vi "Laser_MAIN.vi"() -> ()   [LabVIEW 2013]
doc: "Пограмма управления мишенью лазерного источника ионов."
uses:
  <vilib>/Utility/miscctls.llb/LVPositionTypeDef.ctl
  <vilib>/Utility/inputDevices.llb/closeMouse.vi
panel:
  out "Текущая мишень:":string
  out "Флаг резерв. сохр.":bool
  in  "Шаг \nручного \nсдвига":string(combo)="5" caption="Шаг"
  in  "RightButton":bool
  in  "LeftButton":bool
  in  "DownButton":bool
  in  "UpButton":bool
  in  "М3":T1
  out "Знак перех. dX М10":i8
  out "Выстрелов осталось M10":u16=3
  in  "М10":T1
  in  "выстрел X М10":u16 step=1
  in  "выстрел Y М10":u16 step=1
  out "Знак перех. dX М9":i8
  out "Выстрелов осталось M9":u16=3
  in  "М9":T1
  in  "выстрел X М9":u16 step=1
  in  "выстрел Y М9":u16 step=1
  out "Выстрелов осталось M8":u16=3
  out "Знак перех. dX М8":i8
  in  "М8":T1
  in  "выстрел X М8":u16 step=1
  in  "выстрел Y М8":u16 step=1
  out "Выстрелов осталось M7":u16=3
  out "Знак перех. dX М7":i8
  in  "М7":T1
  in  "выстрел X М7":u16 step=1
  in  "выстрел Y М7":u16 step=1
  out "Выстрелов осталось M6":u16=3
  out "Знак перех. dX М6":i8
  in  "М6":T1
  in  "выстрел X М6":u16 step=1
  in  "выстрел Y М6":u16 step=1
  out "Выстрелов осталось M5":u16=3
  in  "М2":T1
  in  "М5":T1
  out "Знак перех. dX М5":i8
  in  "выстрел Y М5":u16 step=1
  in  "выстрел X М5":u16 step=1
  in  "М4":T1
  out "Знак перех. dX М4":i8
  in  "выстрел Y М4":u16 step=1
  in  "выстрел X М4":u16 step=1
  out "Знак перех. dX М3":i8
  in  "выстрел Y М3":u16 step=1
  in  "выстрел X М3":u16 step=1
  out "Знак перех. dX М2":i8
  in  "выстрел Y М2":u16 step=1
  in  "выстрел X М2":u16 step=1
  in  "выстрел Y М1":u16 step=1
  in  "выстрел X М1":u16 step=1
  out "Знак перех. dX М1":i8
  in  "М1":T1
  out "Выстрелов осталось M4":u16=3
  out "Выстрелов осталось M3":u16=3
  out "Выстрелов осталось M2":u16=3
  out "Выстрелов осталось M1":u16=3
  out "Статус":bool=TRUE caption="Готов!"
  in  "Tab control":enum32{" Мишени", " Настройки TCP"}(tab)
  in  "Перемотка пленки":bool
  in  "Фокус --":bool
  in  "Фокус +":bool
  in  "Сбросить конфигурацию":bool
  in  "Шаг вперед":bool
  in  "XY лазера":bool caption="осталось: 1"
  in  "текущ. инфо":bool caption="4"
  out "флаг закрытия с сохр.":bool
  in  "Загрузить настройки":bool
  in  "Конфигурация сохранена":bool
  in  "Мишень 10":picture
  in  "Мишень 9":picture
  in  "Мишень 8":picture
  in  "Мишень 7":picture
  in  "Мишень 6":picture
  in  "Упр. звуком":bool
  in  "Мишень 5":picture
  in  "Мишень 4":picture
  in  "Мишень 3":picture
  in  "Добавить мишень":bool
  in  "Мишень 2":picture
  in  "Мишень 1":picture
  in  "Выстрелов до перемотки пленки":u16=100
  out "Осталось:":u16(slide)=3 scale=100.0..1.0
  out "id мишени":u16=1
  in  "Счетчик выстрелов:":u32
  in  "TCP read data":string
  out "Slide X axis":u8(slide) max=100 scale=0.0..100.0
  out "Slide Y axis":u8(slide) max=50 step=1
  in  "Снимок сохранен":bool
  out "con err":bool caption="Connect"
  in  "Выстрел по мишени!":u32
  out "Счетчик мишеней":u8=3
  out "Соединение с блоком":bool
  out "Флаг соединения с прибором":bool caption="Connect"
  in  "порт":u16=10001
  in  "IP-адрес":string="172.16.21.200"
  in  "Disconnect":bool caption="Disconn"
  out "Соединение":bool
  in  "Connect":bool
  out "TCP error source":string
  in  "stop":bool
  out "code out":i32 format="%0.0f"
  out "read_error_indicator":bool
  in  "Connect 2":bool caption="Connect"
  in  "flag1":bool caption="Disconn"
  out "x+1":dbl
  out "TCP con ID":refnum<k5>
  out "Текущая конфигурация:":path
  out "Con.err.text":bool caption="Ошибка соединения с блоком..."
  # "Ручное управление \nлазером в пределах \nвыбранной мишени"
  # "Шаг перехода по Y, мм"
  # "Доп. настройки"
  # "Файлы"
  # "Мишени"
  # "Задано:"
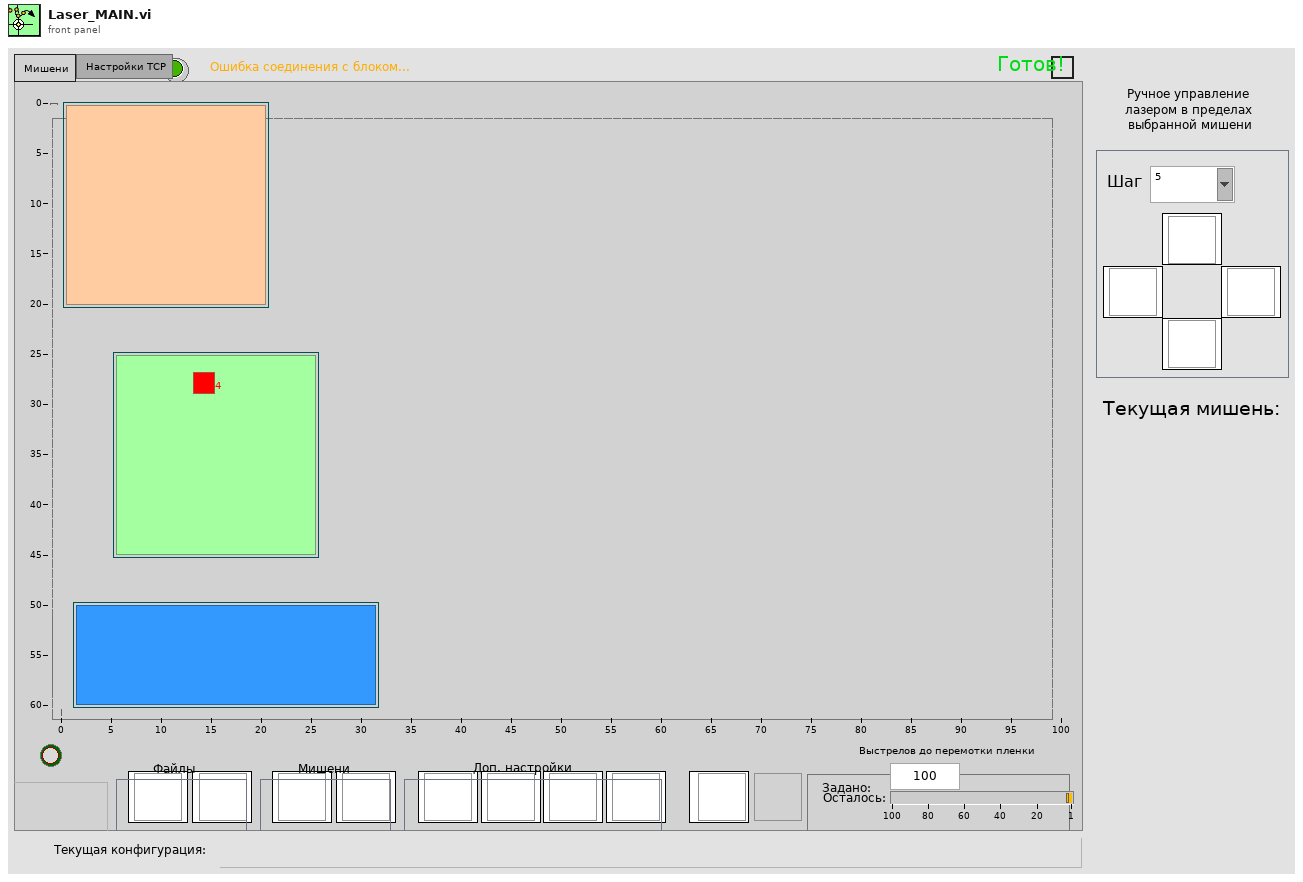
[diagram p1: front panel]
types:
  T1 = cluster{"Название мишени":string, "Х0_position":u16, "Y0_position":u16, "Длина, мм":u16, "Ширина, мм":u16, "Шаг перехода по горизонтали":dbl, "Шаг перехода по вертикали":dbl, "Выстрелов до перехода":u16, "Xo to send ":u16, "Yo to send":u16}
  T2 = enum8{"Enabled", "Disabled", "Disabled and Grayed Out"}
  T3 = typedef "LVPositionTypeDef.ctl" = cluster{"Left":i32, "Top":i32}
  T4 = typedef "imagedata.ctl" = cluster{"image type":i32, "image depth":i32, "image":u8[], "mask":u8[], "colors":u32[], "Rectangle":cluster{"left":i16, "top":i16, "right":i16, "bottom":i16}}
  T5 = cluster{"id команды":u8, "№ мишени":u8, "Коорд. выстрела X ст.байт":u8, "Коорд. выстрела X мл.байт":u8, "Коорд. выстрела Y cт.байт":u8, "Коорд. выстрела Y мл.байт":u8, "Знак dX":i8, "выст. до перех. cт. байт":u8, "выст. до перех. мл. байт":u8, "выст. до перем. пленки ст. байт":u8, "выст. до перем. пленки мл. байт":u8}
  T6 = cluster{"номер мишени (id)":u8, u8, u8, u8, u8, u8, u8, u8, u8, u8, u8, u8, u8, u8, u8, u8, u8, u8, u8, u8}
  T7 = cluster{"доп команда":u8, u8, u8, u8, u8, u8, u8, u8, u8, u8, u8, u8, u8, u8, u8, u8, u8, u8, u8, u8}
  T8 = cluster{"М1":cluster{"Название мишени":string, "Х0_position":u16, "Y0_position":u16, "Длина, мм":u16, "Ширина, мм":u16, "Шаг перехода по горизонтали":dbl, "Шаг перехода по вертикали":dbl, "Выстрелов до перехода":u16, "Xo to send ":u16, "Yo to send":u16}, "М2":cluster{"Название мишени":string, "Х0_position":u16, "Y0_position":u16, "Длина, мм":u16, "Ширина, мм":u16, "Шаг перехода по горизонтали":dbl, "Шаг перехода по вертикали":dbl, "Выстрелов до перехода":u16, "Xo to send ":u16, "Yo to send":u16}, "М3":cluster{"Название мишени":string, "Х0_position":u16, "Y0_position":u16, "Длина, мм":u16, "Ширина, мм":u16, "Шаг перехода по горизонтали":dbl, "Шаг перехода по вертикали":dbl, "Выстрелов до перехода":u16, "Xo to send ":u16, "Yo to send":u16}, "М4":cluster{"Название мишени":string, "Х0_position":u16, "Y0_position":u16, "Длина, мм":u16, "Ширина, мм":u16, "Шаг перехода по горизонтали":dbl, "Шаг перехода по вертикали":dbl, "Выстрелов до перехода":u16, "Xo to send ":u16, "Yo to send":u16}, "М5":cluster{"Название мишени":string, "Х0_position":u16, "Y0_position":u16, "Длина, мм":u16, "Ширина, мм":u16, "Шаг перехода по горизонтали":dbl, "Шаг перехода по вертикали":dbl, "Выстрелов до перехода":u16, "Xo to send ":u16, "Yo to send":u16}, "М6":cluster{"Название мишени":string, "Х0_position":u16, "Y0_position":u16, "Длина, мм":u16, "Ширина, мм":u16, "Шаг перехода по горизонтали":dbl, "Шаг перехода по вертикали":dbl, "Выстрелов до перехода":u16, "Xo to send ":u16, "Yo to send":u16}, "М7":cluster{"Название мишени":string, "Х0_position":u16, "Y0_position":u16, "Длина, мм":u16, "Ширина, мм":u16, "Шаг перехода по горизонтали":dbl, "Шаг перехода по вертикали":dbl, "Выстрелов до перехода":u16, "Xo to send ":u16, "Yo to send":u16}, "М8":cluster{"Название мишени":string, "Х0_position":u16, "Y0_position":u16, "Длина, мм":u16, "Ширина, мм":u16, "Шаг перехода по горизонтали":dbl, "Шаг перехода по вертикали":dbl, "Выстрелов до перехода":u16, "Xo to send ":u16, "Yo to send":u16}, "М9":cluster{"Название мишени":string, "Х0_position":u16, "Y0_position":u16, "Длина, мм":u16, "Ширина, мм":u16, "Шаг перехода по горизонтали":dbl, "Шаг перехода по вертикали":dbl, "Выстрелов до перехода":u16, "Xo to send ":u16, "Yo to send":u16}, "М10":cluster{"Название мишени":string, "Х0_position":u16, "Y0_position":u16, "Длина, мм":u16, "Ширина, мм":u16, "Шаг перехода по горизонтали":dbl, "Шаг перехода по вертикали":dbl, "Выстрелов до перехода":u16, "Xo to send ":u16, "Yo to send":u16}}
  T9 = cluster{"выстрел X М1":u16, "выстрел Y М1":u16, "выстрел X М2":u16, "выстрел Y М2":u16, "выстрел X М3":u16, "выстрел Y М3":u16, "выстрел X М4":u16, "выстрел Y М4":u16, "выстрел X М5":u16, "выстрел Y М5":u16}
  T10 = cluster{"выстрел X М6":u16, "выстрел Y М6":u16, "выстрел X М7":u16, "выстрел Y М7":u16, "выстрел X М8":u16, "выстрел Y М8":u16, "выстрел X М9":u16, "выстрел Y М9":u16, "выстрел X М10":u16, "выстрел Y М10":u16}
  T11 = cluster{"Знак перех. dX М1":i8, "Знак перех. dX М2":i8, "Знак перех. dX М3":i8, "Знак перех. dX М4":i8, "Знак перех. dX М5":i8, "Знак перех. dX М6":i8, "Знак перех. dX М7":i8, "Знак перех. dX М8":i8, "Знак перех. dX М9":i8, "Знак перех. dX М10":i8}
  T12 = cluster{"Мишень 1":picture, "Мишень 2":picture, "Мишень 3":picture, "Мишень 4":picture, "Мишень 5":picture, "Мишень 6":picture, "Мишень 7":picture, "Мишень 8":picture, "Мишень 9":picture, "Мишень 10":picture}
  T13 = cluster{"Visible":bool, "Visible":bool, "Visible":bool, "Visible":bool, "Visible":bool, "Visible":bool, "Visible":bool, "Visible":bool, "Visible":bool, "Visible":bool}
  T14 = cluster{"Выстрелов осталось M1 ":u16, "Выстрелов осталось M2":u16, "Выстрелов осталось M3":u16, "Выстрелов осталось M4":u16, "Выстрелов осталось M5":u16, "Выстрелов осталось M6":u16, "Выстрелов осталось M7":u16, "Выстрелов осталось M8":u16, "Выстрелов осталось M9":u16, "Выстрелов осталось M10":u16}
  T15 = cluster{"Счетчик мишеней":u32, "Счетчик мишеней":u32}
  T16 = cluster{"Счетчик мишеней":i32, "Счетчик мишеней":i32}
  T17 = cluster{"Мишень 1":refnum<vi>, "Мишень 2":refnum<vi>, "Мишень 3":refnum<vi>, "Мишень 4":refnum<vi>, "Мишень 5":refnum<vi>, "Мишень 6":refnum<vi>, "Мишень 7":refnum<vi>, "Мишень 8":refnum<vi>, "Мишень 9":refnum<vi>, "Мишень 10":refnum<vi>}
  T18 = cluster{"Pict Refnum":refnum<vi>, "Pict Refnum 2":refnum<vi>, "Pict Refnum 3":refnum<vi>, "Pict Refnum 4":refnum<vi>, "Pict Refnum 5":refnum<vi>, "Pict Refnum 6":refnum<vi>, "Pict Refnum 7":refnum<vi>, "Pict Refnum 8":refnum<vi>, "Picture in Refnum 9":refnum<vi>, "Pict Refnum 10":refnum<vi>}
  T19 = cluster{"1":u16, "2":u16, "3":u16, "4":u16, "5":u16, "6":u16, "7":u16, "8":u16, "9":u16, "10":u16}
  T20 = cluster{"default value 1":i8, "default value 1":i8, "default value 1":i8, "default value 1":i8, "default value 1":i8, "default value 1":i8, "default value 1":i8, "default value 1":i8, "default value 1":i8, "default value 1":i8}
  T21 = cluster{"Кластер параметров мишени":cluster{"Название мишени":string, "Х0_position":u16, "Y0_position":u16, "Длина, мм":u16, "Ширина, мм":u16, "Шаг перехода по горизонтали":dbl, "Шаг перехода по вертикали":dbl, "Выстрелов до перехода":u16, "Xo to send ":u16, "Yo to send":u16}, "Кластер параметров мишени":cluster{"Название мишени":string, "Х0_position":u16, "Y0_position":u16, "Длина, мм":u16, "Ширина, мм":u16, "Шаг перехода по горизонтали":dbl, "Шаг перехода по вертикали":dbl, "Выстрелов до перехода":u16, "Xo to send ":u16, "Yo to send":u16}, "Кластер параметров мишени":cluster{"Название мишени":string, "Х0_position":u16, "Y0_position":u16, "Длина, мм":u16, "Ширина, мм":u16, "Шаг перехода по горизонтали":dbl, "Шаг перехода по вертикали":dbl, "Выстрелов до перехода":u16, "Xo to send ":u16, "Yo to send":u16}, "Кластер параметров мишени":cluster{"Название мишени":string, "Х0_position":u16, "Y0_position":u16, "Длина, мм":u16, "Ширина, мм":u16, "Шаг перехода по горизонтали":dbl, "Шаг перехода по вертикали":dbl, "Выстрелов до перехода":u16, "Xo to send ":u16, "Yo to send":u16}, "Кластер параметров мишени":cluster{"Название мишени":string, "Х0_position":u16, "Y0_position":u16, "Длина, мм":u16, "Ширина, мм":u16, "Шаг перехода по горизонтали":dbl, "Шаг перехода по вертикали":dbl, "Выстрелов до перехода":u16, "Xo to send ":u16, "Yo to send":u16}, "Кластер параметров мишени":cluster{"Название мишени":string, "Х0_position":u16, "Y0_position":u16, "Длина, мм":u16, "Ширина, мм":u16, "Шаг перехода по горизонтали":dbl, "Шаг перехода по вертикали":dbl, "Выстрелов до перехода":u16, "Xo to send ":u16, "Yo to send":u16}, "Кластер параметров мишени":cluster{"Название мишени":string, "Х0_position":u16, "Y0_position":u16, "Длина, мм":u16, "Ширина, мм":u16, "Шаг перехода по горизонтали":dbl, "Шаг перехода по вертикали":dbl, "Выстрелов до перехода":u16, "Xo to send ":u16, "Yo to send":u16}, "Кластер параметров мишени":cluster{"Название мишени":string, "Х0_position":u16, "Y0_position":u16, "Длина, мм":u16, "Ширина, мм":u16, "Шаг перехода по горизонтали":dbl, "Шаг перехода по вертикали":dbl, "Выстрелов до перехода":u16, "Xo to send ":u16, "Yo to send":u16}, "Кластер параметров мишени":cluster{"Название мишени":string, "Х0_position":u16, "Y0_position":u16, "Длина, мм":u16, "Ширина, мм":u16, "Шаг перехода по горизонтали":dbl, "Шаг перехода по вертикали":dbl, "Выстрелов до перехода":u16, "Xo to send ":u16, "Yo to send":u16}, "Кластер параметров мишени":cluster{"Название мишени":string, "Х0_position":u16, "Y0_position":u16, "Длина, мм":u16, "Ширина, мм":u16, "Шаг перехода по горизонтали":dbl, "Шаг перехода по вертикали":dbl, "Выстрелов до перехода":u16, "Xo to send ":u16, "Yo to send":u16}}
  T22 = enum16{"Left Button", "Center Button", "Right Button", "Window Close"}
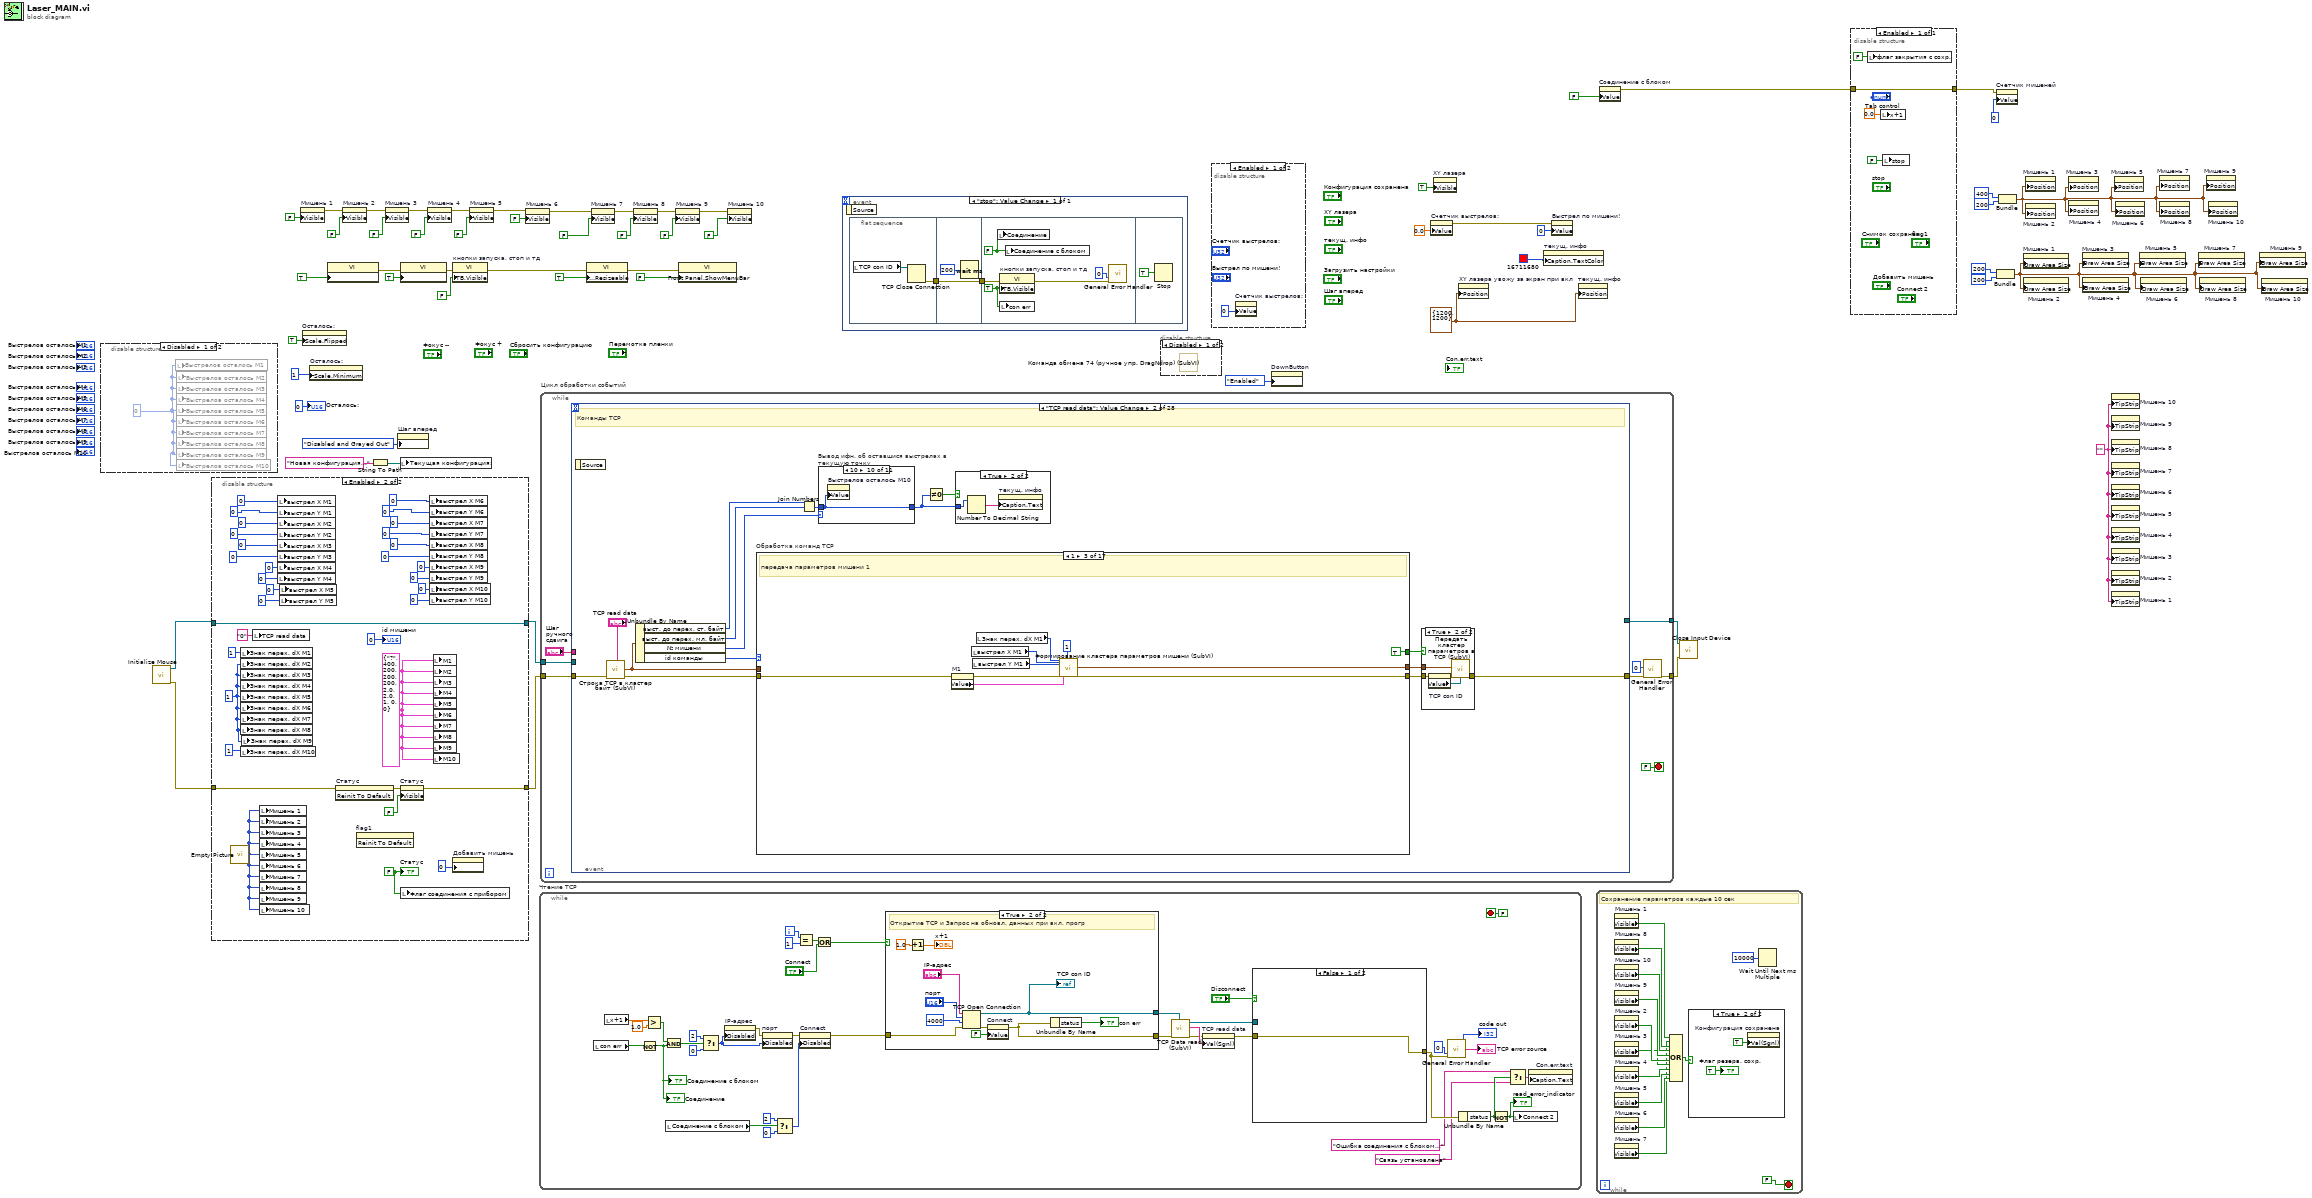
[diagram p0: block diagram]
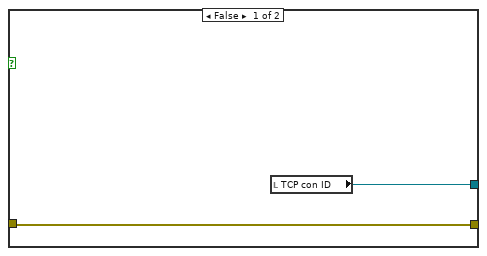
[diagram p5: hidden frame]
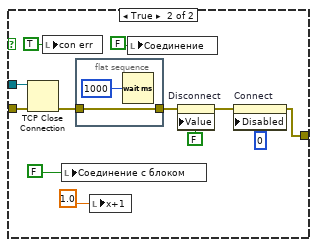
[diagram p6: hidden frame]
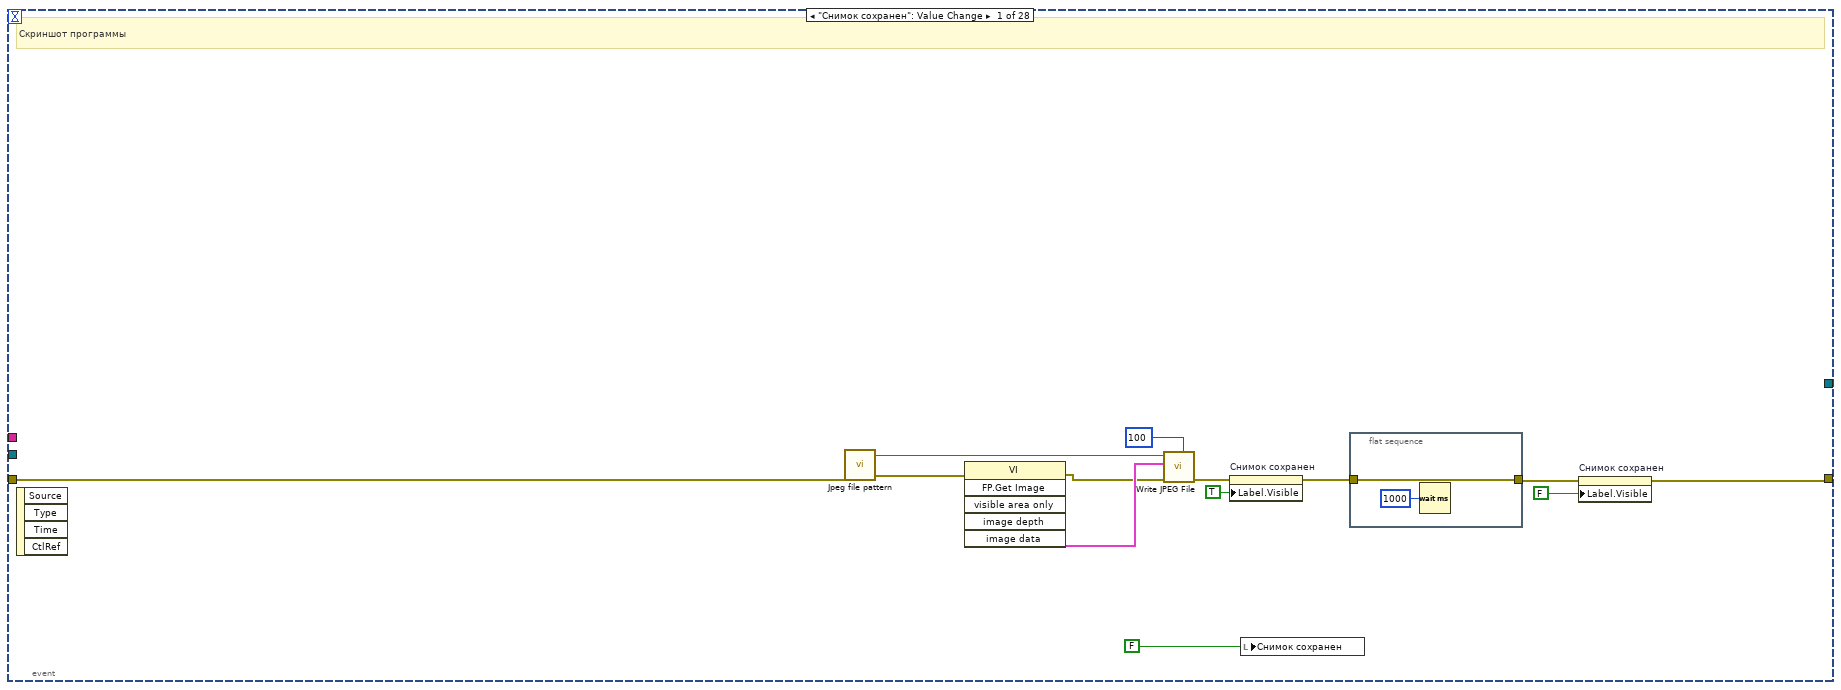
[diagram p9: hidden frame]
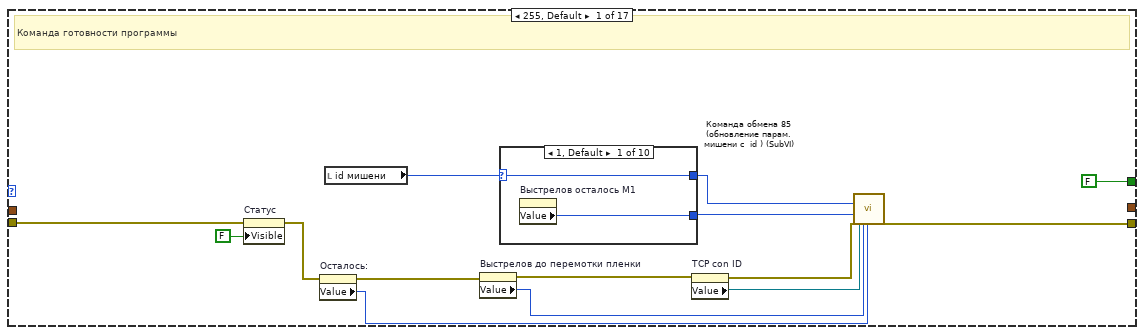
[diagram p12: hidden frame]
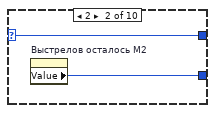
[diagram p13: hidden frame]
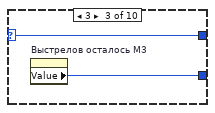
[diagram p14: hidden frame]
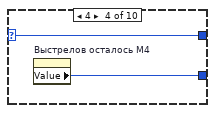
[diagram p15: hidden frame]
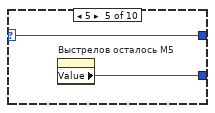
[diagram p16: hidden frame]
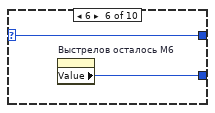
[diagram p17: hidden frame]
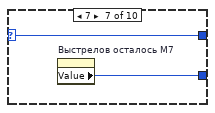
[diagram p18: hidden frame]
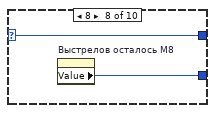
[diagram p19: hidden frame]
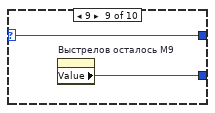
[diagram p20: hidden frame]
diagram:
  w8 = "" ("Tip Strip")
  w49 = T3 {"Left"=1200, "Top"=1200} ("Position")
  n1 = disable-structure shown="Disabled" {
    frame Disabled {
      w59 = u16 0
      n2 = local write "Выстрелов осталось M1"(w59) -> ()
      n3 = local write "Выстрелов осталось M2"(w59) -> ()
      n4 = local write "Выстрелов осталось M3"(w59) -> ()
      n5 = local write "Выстрелов осталось M4"(w59) -> ()
      n6 = local write "Выстрелов осталось M5"(w59) -> ()
      n7 = local write "Выстрелов осталось M6"(w59) -> ()
      n8 = local write "Выстрелов осталось M7"(w59) -> ()
      n9 = local write "Выстрелов осталось M8"(w59) -> ()
      n10 = local write "Выстрелов осталось M9"(w59) -> ()
      n11 = local write "Выстрелов осталось M10"(w59) -> ()
    }
    frame Enabled {
    }
  }
  n12 = call <vilib>:"Initialize Mouse.vi"() -> ("error out"=w51:errorcluster, "device ID"=w53:refnum<k1>)  [unwired: 1 in, 9 out]
  n13 = disable-structure shown="Enabled" {
    disable-tunnel: [_ w93] -> w54
    disable-tunnel: w53 -> [_ w93]
    disable-tunnel: [_ w64] -> w52
    disable-tunnel: w51 -> [_ w92]
    frame Disabled {
    }
    frame Enabled {
      w88 = i8 1 ("Выстрелов осталось M1")
      w89 = T1 {"Название мишени"="?", "Х0_position"=400, "Y0_position"=200, "Длина, мм"=200, "Ширина, мм"=200, "Шаг перехода по горизонтали"=2.0, "Шаг перехода по вертикали"=2.0, "Выстрелов до перехода"=1, "Xo to send "=0, "Yo to send"=0} ("Параметры М1")
      w61 = FALSE ("Готов")
      n14 = call "Empty Picture"() -> ("empty picture"=w65:picture)
      n15 = local write "Знак перех. dX М1"(i8 1 ("Знак перех. dX М1")) -> ()
      n16 = local write "Знак перех. dX М2"(w88) -> ()
      n17 = local write "Знак перех. dX М3"(w88) -> ()
      n18 = local write "Знак перех. dX М4"(w88) -> ()
      n19 = local write "Знак перех. dX М5"(w88) -> ()
      n20 = local write "Знак перех. dX М6"(w88) -> ()
      n21 = local write "Знак перех. dX М7"(w88) -> ()
      n22 = local write "Знак перех. dX М8"(w88) -> ()
      n23 = local write "Знак перех. dX М10"(i8 1 ("Выстрелов осталось M1")) -> ()
      n24 = local write "Знак перех. dX М9"(w88) -> ()
      n25 = local write "TCP read data"("0" ("TCP read data")) -> ()
      n26 = local write "Мишень 1"(w65) -> ()
      n27 = local write "Мишень 2"(w65) -> ()
      n28 = local write "Мишень 3"(w65) -> ()
      n29 = local write "Мишень 4"(w65) -> ()
      n30 = local write "Мишень 5"(w65) -> ()
      n31 = local write "Мишень 6"(w65) -> ()
      n32 = local write "Мишень 7"(w65) -> ()
      n33 = local write "Мишень 8"(w65) -> ()
      n34 = local write "Мишень 9"(w65) -> ()
      n35 = local write "Мишень 10"(w65) -> ()
      n36 = local write "выстрел X М1"(u16 0 ("Выстрелов осталось M1")) -> ()
      n37 = local write "выстрел Y М1"(u16 0 ("Выстрелов осталось M2")) -> ()
      n38 = local write "выстрел X М2"(u16 0 ("Выстрелов осталось M3")) -> ()
      n39 = local write "выстрел Y М2"(u16 0 ("Выстрелов осталось M4")) -> ()
      n40 = local write "выстрел X М3"(u16 0 ("Выстрелов осталось M5")) -> ()
      n41 = local write "выстрел Y М3"(u16 0 ("Выстрелов осталось M6")) -> ()
      n42 = local write "выстрел X М4"(u16 0 ("выстрел X М9")) -> ()
      n43 = local write "выстрел Y М4"(u16 0 ("выстрел Y М9")) -> ()
      n44 = local write "выстрел X М5"(u16 0 ("выстрел X М10")) -> ()
      n45 = local write "выстрел Y М5"(u16 0 ("выстрел Y М10")) -> ()
      n46 = invoke on="Статус" class="Bool (strict)" method="Reinit To Default"(error in=w92) -> (error out=w90:errorcluster)  [unwired: 2 in, 2 out]
      n47 = invoke on="flag1" class="Bool (strict)" method="Reinit To Default"() -> ()  [unwired: 3 in, 3 out]
      n48 = property on="Статус" class="Bool (strict)"(error in=w90, "Visible"=FALSE) -> (error out=w64:errorcluster)  [unwired: 1 in, 1 out]
      n49 = local write "Флаг соединения с прибором"(w61) -> ()
      n50 = local write "выстрел X М6"(u16 0 ("Выстрелов осталось M1")) -> ()
      n51 = local write "выстрел Y М6"(u16 0 ("Выстрелов осталось M2")) -> ()
      n52 = local write "выстрел X М7"(u16 0 ("Выстрелов осталось M3")) -> ()
      n53 = local write "выстрел Y М7"(u16 0 ("Выстрелов осталось M4")) -> ()
      n54 = local write "выстрел X М8"(u16 0 ("Выстрелов осталось M5")) -> ()
      n55 = local write "выстрел Y М8"(u16 0 ("Выстрелов осталось M6")) -> ()
      n56 = local write "выстрел X М9"(u16 0 ("выстрел X М9")) -> ()
      n57 = local write "выстрел Y М9"(u16 0 ("выстрел Y М9")) -> ()
      n58 = local write "выстрел X М10"(u16 0 ("выстрел X М10")) -> ()
      n59 = local write "выстрел Y М10"(u16 0 ("выстрел Y М10")) -> ()
      n60 = local write "М1"(w89) -> ()
      n61 = local write "М2"(w89) -> ()
      n62 = local write "М3"(w89) -> ()
      n63 = local write "М4"(w89) -> ()
      n64 = local write "М5"(w89) -> ()
      n65 = local write "М6"(w89) -> ()
      n66 = local write "М7"(w89) -> ()
      n67 = local write "М8"(w89) -> ()
      n68 = local write "М9"(w89) -> ()
      n69 = local write "М10"(w89) -> ()
      n70 = property on="Добавить мишень" class="Bool (strict)"("DisabledEnum"=i8 0 ("Выстрелов осталось M1")) -> ()  [unwired: 2 in, 2 out]
      "Статус" <- w61
      "id мишени" <- u16 0 ("id мишени")
    }
  }
  n71 = property on="Мишень 1" class="Pict"("Visible"=FALSE) -> (error out=w35:errorcluster)  [unwired: 2 in, 1 out]
  n72 = property on="Осталось:" class="Slide (strict)"("Scale.Flipped"=TRUE) -> ()  [unwired: 2 in, 2 out]
  n73 = property on="Осталось:" class="Slide (strict)"("Scale.Minimum"=u16 1 ("До перемотки осталось")) -> ()  [unwired: 2 in, 2 out]
  n74 = property class="VI"("Front Panel.Minimizeable"=TRUE ("Front Panel Window:Minimizable")) -> (error out=w41:errorcluster)  [unwired: 2 in, 1 out]
  n75 = property on="Мишень 2" class="Pict"(error in=w35, "Visible"=FALSE) -> (error out=w32:errorcluster)  [unwired: 1 in, 1 out]
  n76 = String To Path(string="Новая конфигурация...") -> (path=w7:path)
  n77 = property on="Мишень 3" class="Pict"(error in=w32, "Visible"=FALSE) -> (error out=w30:errorcluster)  [unwired: 1 in, 1 out]
  n78 = property on="Шаг вперед" class="Bool (strict)"("DisabledEnum"=T2."Disabled and Grayed Out" ("Disabled")) -> ()  [unwired: 2 in, 2 out]
  n79 = property class="VI"(error in=w41, "Front Panel.TitleBarVis"=TRUE ("Front Panel Window:Title Bar Visible")) -> (error out=w40:errorcluster)  [unwired: 1 in, 1 out]
  n80 = local write "Текущая конфигурация:"(w7) -> ()
  n81 = property on="Мишень 4" class="Pict"(error in=w30, "Visible"=FALSE) -> (error out=w28:errorcluster)  [unwired: 1 in, 1 out]
  n82 = property on="кнопки запуска, стоп и тд" class="VI"(error in=w40, "TB.Visible"=FALSE ("Tool Bar:Visible")) -> (error out=w39:errorcluster)  [unwired: 1 in, 1 out]
  n83 = property on="Мишень 5" class="Pict"(error in=w28, "Visible"=FALSE) -> (error out=w16:errorcluster)  [unwired: 1 in, 1 out]
  n84 = property on="Мишень 6" class="Pict"(error in=w16, "Visible"=FALSE) -> (error out=w17:errorcluster)  [unwired: 1 in, 1 out]
  n85 = while "Чтение TCP" {
    i -> [w124]
    stop <- FALSE stop-if-true
    n86 = local read "con err"() -> (w112:bool)
    n87 = local read "x+1"() -> (w115:dbl)
    n88 = Not(x=w112) -> (.not. x?=w101:bool)
    "Соединение" <- w101
    "Соединение с блоком" <- w101
    n89 = Greater?(x=w115, y=1.0) -> (0:w113:bool)
    n90 = And(x=w113, y=w101) -> (x .and. y?=w109:bool)
    n91 = local read "Соединение с блоком"() -> (w106:bool)
    n92 = Select(t=u8 2 ("Disabled"), s=w109, f=u8 0 ("Disabled")) -> (s? t:f=w130:u8)
    n93 = property on="IP-адрес" class="Str"("Disabled"=w130) -> (error out=w129:errorcluster)  [unwired: 2 in, 1 out]
    n94 = property on="порт" class="DigNum (strict)"(error in=w129, "Disabled"=w130) -> (error out=w128:errorcluster)  [unwired: 1 in, 1 out]
    n95 = Select(t=u8 2 ("Disabled"), s=w106, f=u8 0 ("Disabled")) -> (s? t:f=w117:u8)
    n96 = Equal?(x=w124, y=1) -> (x = y?=w125:bool)
    n97 = property on="Connect" class="Bool (strict)"(error in=w128, "Disabled"=w117) -> (error out=w122:errorcluster)  [unwired: 1 in, 1 out]
    n98 = Or(x=w125, y="Connect") -> (x .or. y?=w127:bool)
    n99 = case shown="True" w127 {
      tunnel: [w133 w134] -> w103
      tunnel: w122 -> [w133 w136]
      tunnel: [w132 w135] -> w102
      frame False {
        n100 = local read "TCP con ID"() -> (w132:refnum<k5>)
      }
      frame True {
        # "Открытие TCP и Запрос на обновл. данных при вкл. прогр"
        n101 = Increment(x=1.0) -> (x+1=→"x+1":dbl)
        n102 = TCP Open Connection(address="IP-адрес", remote port or service name="порт", timeout ms (60000)=4000, error in (no error)=w136) -> (connection ID=w135:refnum<k5>, error out=w138:errorcluster)  [unwired: 1 out]
        "TCP con ID" <- w135
        n103 = property on="Connect" class="Bool (strict)"(error in=w138, "Value"=FALSE ("Connect")) -> (error out=w134:errorcluster)  [unwired: 1 in, 1 out]
        n104 = Unbundle By Name(w134) -> ("status"=→"con err":bool)
      }
    }
    n105 = call "TCP Data read (SubVI).vi"("error in (no error)"=w103, "TCP Network Connection in"=w102) -> ("error out"=w104:errorcluster, "Read data"=w118:string, "TCP Network Connection out"=w120:refnum<k5>)  [unwired: 1 in, 6 out]
    n106 = property on="TCP read data" class="Str"(error in=w104, "Val(Sgnl)"=w118) -> (error out=w105:errorcluster)  [unwired: 1 in, 1 out]
    n107 = case shown="False" "Disconnect" {
      tunnel: [w145 w154] -> w100
      tunnel: w105 -> [w145 w153]
      tunnel: w120 -> [_ w152]
      frame False {
      }
      frame True {
        n108 = TCP Close Connection(connection ID=w152, error in (no error)=w153) -> (error out=w155:errorcluster)  [unwired: 2 out]
        n109 = local write "con err"(TRUE ("con err")) -> ()
        n110 = local write "Соединение с блоком"(FALSE ("Disconnect")) -> ()
        n111 = flat-sequence {
          tunnel: w155 -> [w158]
          tunnel: [w158] -> w150
          frame #0 {
            n112 = Wait (ms)(milliseconds to wait=u32 1000) -> ()  [unwired: 1 out]
          }
        }
        n113 = local write "x+1"(1.0 ("1")) -> ()
        n114 = local write "Соединение"(FALSE ("Disconnect")) -> ()
        n115 = property on="Disconnect" class="Bool (strict)"(error in=w150, "Value"=FALSE ("Disconnect")) -> (error out=w156:errorcluster)  [unwired: 1 in, 1 out]
        n116 = property on="Connect" class="Bool (strict)"(error in=w156, "Disabled"=u8 0) -> (error out=w154:errorcluster)  [unwired: 1 in, 1 out]
      }
    }
    n117 = call <vilib>:"General Error Handler.vi"("type of dialog (OK msg:1)"=u8 0, "error in (no error)"=w100) -> ("code out"=→"code out":i32, "source out"=→"TCP error source":string)  [unwired: 12 out]
    n118 = Unbundle By Name(w100) -> ("status"=w97:bool)
    n119 = Not(x=w97) -> (.not. x?=w98:bool)
    "read_error_indicator" <- w98
    n120 = Select(t="Ошибка соединения с блоком..." ("Caption.Text"), s=w97, f="Связь установлена" ("Caption.Text")) -> (s? t:f=w95:string)
    n121 = local write "Connect 2"(w98) -> ()
    n122 = property on="Con.err.text" class="Bool (strict)"("Caption.Text"=w95) -> ()  [unwired: 2 in, 2 out]
  }
  n123 = while "Цикл обработки событий" {
    tunnel: w52 -> [w166]
    tunnel: w54 -> [w165]
    tunnel: [w162] -> w50
    tunnel: [w161] -> w48
    stop <- FALSE stop-if-true
    n124 = event shown="[1] \"TCP read data\": Value Change" {
      selector: _ -> [_ _ _ _ _ _ _ _ _ _ _ _ _ _ _ _ _ _ _ _ _ _ _ _ _ _ _ _]
      dyn-events: _ -> [_ _ _ _ _ _ _ _ _ _ _ _ _ _ _ _ _ _ _ _ _ _ _ _ _ _ _ _]
      timeout: _ -> [_ _ _ _ _ _ _ _ _ _ _ _ _ _ _ _ _ _ _ _ _ _ _ _ _ _ _ _]
      tunnel: [w168 w197 w755 w867 w882 w917 w944 w970 w996 w1022 w1048 w1074 w1100 w1126 w1152 w1186 w1219 w1225 w1229 w1234 w1250 w1289 w1346 w1394 w1432 _ w1613 _] -> w163
      tunnel: w166 -> [w176 w196 w761 w871 w881 w918 w943 w969 w995 w1021 w1047 w1073 w1099 w1125 w1151 w1179 w1220 w1228 w1233 w1238 w1242 w1292 w1340 w1388 w1433 _ w1618 _]
      tunnel: w165 -> [_ _ _ w872 _ _ _ _ _ _ _ _ _ _ _ _ _ _ _ _ _ _ _ _ _ _ _ _]
      tunnel: [_ _ _ w870 _ _ _ _ _ _ _ _ _ _ _ _ _ _ _ _ _ _ _ _ _ _ _ _] -> w161
      tunnel: "Шаг \nручного \nсдвига" -> [_ _ _ _ _ _ _ _ _ _ _ _ _ _ _ _ _ _ _ _ w1244 w1294 w1342 w1390 _ _ _ _]
      event "Снимок сохранен": Value Change {
        # "Скриншот программы"
        n125 = event-data() -> ()  [unwired: 5 out]
        n126 = call "Jpeg file pattern.vi"("error in"=w176) -> ("path to JPG file"=w177:path, "error out"=w175:errorcluster)  [unwired: 7 in]
        n127 = invoke class="VI" method="FP.Get Image"(error in=w175) -> (error out=w174:errorcluster, "image data"=w178:T4)  [unwired: 5 in, 4 out]
        n128 = call <vilib>:"Write JPEG File.vi"("quality (80)"=100, "error in (no error)"=w174, "image data"=w178, "path to JPEG file"=w177) -> ("error out"=w171:errorcluster)  [unwired: 7 out]
        n129 = property on="Снимок сохранен" class="Bool (strict)"(error in=w171, "Label.Visible"=TRUE) -> (error out=w169:errorcluster)  [unwired: 1 in, 1 out]
        n130 = local write "Снимок сохранен"(FALSE ("Снимок")) -> ()
        n131 = flat-sequence {
          tunnel: [w182] -> w170
          tunnel: w169 -> [w182]
          frame #0 {
            n132 = Wait (ms)(milliseconds to wait=u32 1000) -> ()  [unwired: 1 out]
          }
        }
        n133 = property on="Снимок сохранен" class="Bool (strict)"(error in=w170, "Label.Visible"=FALSE) -> (error out=w168:errorcluster)  [unwired: 1 in, 1 out]
      }
      event "TCP read data": Value Change {
        # "Команды TCP"
        n134 = event-data() -> ()  [unwired: 2 out]
        n135 = call "Строка TCP в кластер байт (SubVI).vi"("TCP read data"="TCP read data", "error in"=w196) -> ("Кластер прочитанных байт"=w193:T5, "error out"=w190:errorcluster)  [unwired: 12 in]
        n136 = Unbundle By Name(w193) -> ("выст. до перех. cт. байт"=w188:u8, "выст. до перех. мл. байт"=w187:u8, "№ мишени"=w186:u8, "id команды"=w194:u8)
        n137 = case "Обработка команд TCP" shown="1" w194 {
          tunnel: w193 -> [_ _ _ _ _ _ _ _ _ _ _ _ _ w374 w459 w603 _]
          tunnel: w190 -> [w217 w241 w249 w259 w269 w279 w289 w299 w309 w319 w329 w339 w346 w365 w470 w602 _]
          tunnel: [w216 w241 w252 w262 w272 w282 w292 w302 w312 w322 w332 w342 w345 w355 w458 w599 _] -> w192
          tunnel: [_ _ w244 w254 w264 w274 w284 w294 w304 w314 w324 w334 w344 _ _ _ _] -> w191
          tunnel: [FALSE FALSE TRUE TRUE TRUE TRUE TRUE TRUE TRUE TRUE TRUE TRUE FALSE FALSE FALSE FALSE _] -> w189
          frame 255, Default {
            # "Команда готовности программы"
            n138 = property on="Статус" class="Bool (strict)"(error in=w217, "Visible"=FALSE) -> (error out=w218:errorcluster)  [unwired: 1 in, 1 out]
            n139 = property on="Осталось:" class="Slide (strict)"(error in=w218) -> (error out=w213:errorcluster, "Value"=w211:u16)  [unwired: 1 in, 1 out]
            n140 = local read "id мишени"() -> (w214:u16)
            n141 = property on="Выстрелов до перемотки пленки" class="DigNum (strict)"(error in=w213) -> (error out=w212:errorcluster, "Value"=w210:u16)  [unwired: 1 in, 1 out]
            n142 = case shown="1, Default" w214 {
              selector: w214 -> [w220 w222 w224 w226 w228 w230 w232 w234 w236 w238]
              tunnel: [w221 w223 w225 w227 w229 w231 w233 w235 w237 w239] -> w207
              tunnel: [w220 w222 w224 w226 w228 w230 w232 w234 w236 w238] -> w206
              frame 1, Default {
                n143 = property on="Выстрелов осталось M1" class="DigNum (strict)"() -> ("Value"=w221:u16)  [unwired: 2 in, 2 out]
              }
              frame 2 {
                n144 = property on="Выстрелов осталось M2" class="DigNum (strict)"() -> ("Value"=w223:u16)  [unwired: 2 in, 2 out]
              }
              frame 3 {
                n145 = property on="Выстрелов осталось M3" class="DigNum (strict)"() -> ("Value"=w225:u16)  [unwired: 2 in, 2 out]
              }
              frame 4 {
                n146 = property on="Выстрелов осталось M4" class="DigNum (strict)"() -> ("Value"=w227:u16)  [unwired: 2 in, 2 out]
              }
              frame 5 {
                n147 = property on="Выстрелов осталось M5" class="DigNum (strict)"() -> ("Value"=w229:u16)  [unwired: 2 in, 2 out]
              }
              frame 6 {
                n148 = property on="Выстрелов осталось M6" class="DigNum (strict)"() -> ("Value"=w231:u16)  [unwired: 2 in, 2 out]
              }
              frame 7 {
                n149 = property on="Выстрелов осталось M7" class="DigNum (strict)"() -> ("Value"=w233:u16)  [unwired: 2 in, 2 out]
              }
              frame 8 {
                n150 = property on="Выстрелов осталось M8" class="DigNum (strict)"() -> ("Value"=w235:u16)  [unwired: 2 in, 2 out]
              }
              frame 9 {
                n151 = property on="Выстрелов осталось M9" class="DigNum (strict)"() -> ("Value"=w237:u16)  [unwired: 2 in, 2 out]
              }
              frame 10 {
                n152 = property on="Выстрелов осталось M10" class="DigNum (strict)"() -> ("Value"=w239:u16)  [unwired: 2 in, 2 out]
              }
            }
            n153 = property on="TCP con ID" class="Ref (strict)"(error in=w212) -> (error out=w209:errorcluster, "Value"=w208:refnum<k5>)  [unwired: 1 in, 1 out]
            n154 = call "Команда обмена 85 (обновление парам. мишени с  id ) (SubVI).vi"("id мишени"=w206, "Выстрелов осталось"=w207, "error in"=w209, "TCP connection ID"=w208, "Выстрелов до перемотки"=w210, "До перемотки осталось"=w211) -> ("error out"=w216:errorcluster)  [unwired: 21 in]
          }
          frame 254 {
            # "Команда анализа активного соединения с прибором"
            "Флаг соединения с прибором" <- TRUE ("Флаг соединения с прибором")
          }
          frame 1 {
            # "передача параметров мишени 1"
            n155 = property on="М1" class="Clust (strict)"(error in=w249) -> (error out=w251:errorcluster, "Value"=w250:T1)  [unwired: 1 in, 1 out]
            n156 = local read "выстрел X М1"() -> (w246:u16)
            n157 = local read "выстрел Y М1"() -> (w245:u16)
            n158 = local read "Знак перех. dX М1"() -> (w247:i8)
            n159 = call "Формирование кластера параметров мишени (SubVI).vi"("Знак перемещения Dx"=w247, "выстрел X мишени"=w246, "выстрел Y мишени"=w245, "error in (no error)"=w251, "Параметры Мишени"=w250, "номер мишени (id)"=u8 1) -> ("Кластер параметров мишени"=w244:T6, "error out"=w252:errorcluster)  [unwired: 20 in]
          }
          frame 2 {
            # "передача параметров мишени 2"
            n160 = property on="М2" class="Clust (strict)"(error in=w259) -> (error out=w261:errorcluster, "Value"=w260:T1)  [unwired: 1 in, 1 out]
            n161 = local read "выстрел X М2"() -> (w256:u16)
            n162 = local read "выстрел Y М2"() -> (w255:u16)
            n163 = local read "Знак перех. dX М2"() -> (w257:i8)
            n164 = call "Формирование кластера параметров мишени (SubVI).vi"("Знак перемещения Dx"=w257, "выстрел X мишени"=w256, "выстрел Y мишени"=w255, "error in (no error)"=w261, "Параметры Мишени"=w260, "номер мишени (id)"=u8 2) -> ("Кластер параметров мишени"=w254:T6, "error out"=w262:errorcluster)  [unwired: 20 in]
          }
          frame 3 {
            # "передача параметров мишени 3"
            n165 = property on="М3" class="Clust (strict)"(error in=w269) -> (error out=w271:errorcluster, "Value"=w270:T1)  [unwired: 1 in, 1 out]
            n166 = local read "выстрел X М3"() -> (w266:u16)
            n167 = local read "выстрел Y М3"() -> (w265:u16)
            n168 = local read "Знак перех. dX М3"() -> (w267:i8)
            n169 = call "Формирование кластера параметров мишени (SubVI).vi"("Знак перемещения Dx"=w267, "выстрел X мишени"=w266, "выстрел Y мишени"=w265, "error in (no error)"=w271, "Параметры Мишени"=w270, "номер мишени (id)"=u8 3) -> ("Кластер параметров мишени"=w264:T6, "error out"=w272:errorcluster)  [unwired: 20 in]
          }
          frame 4 {
            # "передача параметров мишени 4"
            n170 = property on="М4" class="Clust (strict)"(error in=w279) -> (error out=w281:errorcluster, "Value"=w280:T1)  [unwired: 1 in, 1 out]
            n171 = local read "выстрел X М4"() -> (w276:u16)
            n172 = local read "выстрел Y М4"() -> (w275:u16)
            n173 = local read "Знак перех. dX М4"() -> (w277:i8)
            n174 = call "Формирование кластера параметров мишени (SubVI).vi"("Знак перемещения Dx"=w277, "выстрел X мишени"=w276, "выстрел Y мишени"=w275, "error in (no error)"=w281, "Параметры Мишени"=w280, "номер мишени (id)"=u8 4) -> ("Кластер параметров мишени"=w274:T6, "error out"=w282:errorcluster)  [unwired: 20 in]
          }
          frame 5 {
            # "передача параметров мишени 5"
            n175 = property on="М5" class="Clust (strict)"(error in=w289) -> (error out=w291:errorcluster, "Value"=w290:T1)  [unwired: 1 in, 1 out]
            n176 = local read "выстрел X М5"() -> (w286:u16)
            n177 = local read "выстрел Y М5"() -> (w285:u16)
            n178 = local read "Знак перех. dX М5"() -> (w287:i8)
            n179 = call "Формирование кластера параметров мишени (SubVI).vi"("Знак перемещения Dx"=w287, "выстрел X мишени"=w286, "выстрел Y мишени"=w285, "error in (no error)"=w291, "Параметры Мишени"=w290, "номер мишени (id)"=u8 5) -> ("Кластер параметров мишени"=w284:T6, "error out"=w292:errorcluster)  [unwired: 20 in]
          }
          frame 6 {
            # "передача параметров мишени 6"
            n180 = property on="М6" class="Clust (strict)"(error in=w299) -> (error out=w301:errorcluster, "Value"=w300:T1)  [unwired: 1 in, 1 out]
            n181 = local read "выстрел X М6"() -> (w296:u16)
            n182 = local read "выстрел Y М6"() -> (w295:u16)
            n183 = local read "Знак перех. dX М6"() -> (w297:i8)
            n184 = call "Формирование кластера параметров мишени (SubVI).vi"("Знак перемещения Dx"=w297, "выстрел X мишени"=w296, "выстрел Y мишени"=w295, "error in (no error)"=w301, "Параметры Мишени"=w300, "номер мишени (id)"=u8 6) -> ("Кластер параметров мишени"=w294:T6, "error out"=w302:errorcluster)  [unwired: 20 in]
          }
          frame 7 {
            # "передача параметров мишени 7"
            n185 = property on="М7" class="Clust (strict)"(error in=w309) -> (error out=w311:errorcluster, "Value"=w310:T1)  [unwired: 1 in, 1 out]
            n186 = local read "выстрел X М7"() -> (w306:u16)
            n187 = local read "выстрел Y М7"() -> (w305:u16)
            n188 = local read "Знак перех. dX М7"() -> (w307:i8)
            n189 = call "Формирование кластера параметров мишени (SubVI).vi"("Знак перемещения Dx"=w307, "выстрел X мишени"=w306, "выстрел Y мишени"=w305, "error in (no error)"=w311, "Параметры Мишени"=w310, "номер мишени (id)"=u8 7) -> ("Кластер параметров мишени"=w304:T6, "error out"=w312:errorcluster)  [unwired: 20 in]
          }
          frame 8 {
            # "передача параметров мишени 8"
            n190 = property on="М8" class="Clust (strict)"(error in=w319) -> (error out=w321:errorcluster, "Value"=w320:T1)  [unwired: 1 in, 1 out]
            n191 = local read "выстрел X М8"() -> (w316:u16)
            n192 = local read "выстрел Y М8"() -> (w315:u16)
            n193 = local read "Знак перех. dX М8"() -> (w317:i8)
            n194 = call "Формирование кластера параметров мишени (SubVI).vi"("Знак перемещения Dx"=w317, "выстрел X мишени"=w316, "выстрел Y мишени"=w315, "error in (no error)"=w321, "Параметры Мишени"=w320, "номер мишени (id)"=u8 8) -> ("Кластер параметров мишени"=w314:T6, "error out"=w322:errorcluster)  [unwired: 20 in]
          }
          frame 9 {
            # "передача параметров мишени 9"
            n195 = property on="М9" class="Clust (strict)"(error in=w329) -> (error out=w331:errorcluster, "Value"=w330:T1)  [unwired: 1 in, 1 out]
            n196 = local read "выстрел X М9"() -> (w326:u16)
            n197 = local read "выстрел Y М9"() -> (w325:u16)
            n198 = local read "Знак перех. dX М9"() -> (w327:i8)
            n199 = call "Формирование кластера параметров мишени (SubVI).vi"("Знак перемещения Dx"=w327, "выстрел X мишени"=w326, "выстрел Y мишени"=w325, "error in (no error)"=w331, "Параметры Мишени"=w330, "номер мишени (id)"=u8 9) -> ("Кластер параметров мишени"=w324:T6, "error out"=w332:errorcluster)  [unwired: 20 in]
          }
          frame 10 {
            # "передача параметров мишени 10"
            n200 = property on="М10" class="Clust (strict)"(error in=w339) -> (error out=w341:errorcluster, "Value"=w340:T1)  [unwired: 1 in, 1 out]
            n201 = local read "выстрел X М10"() -> (w336:u16)
            n202 = local read "выстрел Y М10"() -> (w335:u16)
            n203 = local read "Знак перех. dX М10"() -> (w337:i8)
            n204 = call "Формирование кластера параметров мишени (SubVI).vi"("Знак перемещения Dx"=w337, "выстрел X мишени"=w336, "выстрел Y мишени"=w335, "error in (no error)"=w341, "Параметры Мишени"=w340, "номер мишени (id)"=u8 10) -> ("Кластер параметров мишени"=w334:T6, "error out"=w342:errorcluster)  [unwired: 20 in]
          }
          frame 15 {
            # "Доп. команда"
            n205 = disable-structure shown="Disabled" {
              disable-tunnel: "Выстрелов до перемотки пленки" -> [w352 _]
              disable-tunnel: w346 -> [w351 w353]
              disable-tunnel: [w350 w353] -> w345
              disable-tunnel: [w349 _] -> w344
              frame Disabled {
                n206 = local read "id мишени"() -> (w348:u16)
                n207 = call "Команда обмена 5 (доп. команда) (SubVI).vi"("Выстрелов до перемотки"=w352, "error in"=w351, "номер мишени (id)"=w348) -> ("Кластер параметров 15-ой команды"=w349:T7, "error out"=w350:errorcluster)  [unwired: 23 in]
              }
              frame Enabled {
              }
            }
          }
          frame 170 {
            # "ВЫСТРЕЛ!"
            n208 = Unbundle By Name(w374) -> ("№ мишени"=w368:u8, "Коорд. выстрела X ст.байт"=w373:u8, "Коорд. выстрела X мл.байт"=w372:u8, "Коорд. выстрела Y cт.байт"=w371:u8, "Коорд. выстрела Y мл.байт"=w370:u8, "Знак dX"=w369:i8, "выст. до перем. пленки ст. байт"=w367:u8, "выст. до перем. пленки мл. байт"=w366:u8)
            n209 = Join Numbers(hi=w367, lo=w366) -> ((hi.lo)=w363:u16)
            n210 = property on="Осталось:" class="Slide (strict)"(error in=w365, "Value"=w363) -> (error out=w364:errorcluster)  [unwired: 1 in, 1 out]
            n211 = case shown="1, Default" w368 {
              tunnel: w373 -> [w385 w393 w400 w409 w417 w425 w433 w441 w449 w457]
              tunnel: w372 -> [w384 w392 w399 w408 w416 w424 w432 w440 w448 w456]
              tunnel: w371 -> [w383 w391 w398 w407 w415 w423 w431 w439 w447 w455]
              tunnel: w370 -> [w382 w390 w401 w406 w414 w422 w430 w438 w446 w454]
              tunnel: w369 -> [w380 w386 w396 w404 w410 w418 w426 w434 w442 w450]
              tunnel: w364 -> [w381 w389 w397 w405 w413 w421 w429 w437 w445 w453]
              tunnel: [w381 w389 w397 w405 w413 w421 w429 w437 w445 w453] -> w359
              frame 1, Default {
                n212 = Join Numbers(hi=w385, lo=w384) -> ((hi.lo)=w379:u16)
                n213 = Join Numbers(hi=w383, lo=w382) -> ((hi.lo)=w378:u16)
                n214 = local write "выстрел X М1"(w379) -> ()
                n215 = local write "выстрел Y М1"(w378) -> ()
                "Знак перех. dX М1" <- w380
              }
              frame 2 {
                n216 = Join Numbers(hi=w393, lo=w392) -> ((hi.lo)=w388:u16)
                n217 = Join Numbers(hi=w391, lo=w390) -> ((hi.lo)=w387:u16)
                n218 = local write "выстрел X М2"(w388) -> ()
                n219 = local write "выстрел Y М2"(w387) -> ()
                "Знак перех. dX М2" <- w386
              }
              frame 3 {
                n220 = Join Numbers(hi=w400, lo=w399) -> ((hi.lo)=w395:u16)
                n221 = Join Numbers(hi=w398, lo=w401) -> ((hi.lo)=w394:u16)
                n222 = local write "выстрел X М3"(w395) -> ()
                n223 = local write "выстрел Y М3"(w394) -> ()
                "Знак перех. dX М3" <- w396
              }
              frame 4 {
                n224 = Join Numbers(hi=w409, lo=w408) -> ((hi.lo)=w403:u16)
                n225 = Join Numbers(hi=w407, lo=w406) -> ((hi.lo)=w402:u16)
                n226 = local write "выстрел X М4"(w403) -> ()
                n227 = local write "выстрел Y М4"(w402) -> ()
                "Знак перех. dX М4" <- w404
              }
              frame 5 {
                n228 = Join Numbers(hi=w417, lo=w416) -> ((hi.lo)=w412:u16)
                n229 = Join Numbers(hi=w415, lo=w414) -> ((hi.lo)=w411:u16)
                n230 = local write "выстрел X М5"(w412) -> ()
                n231 = local write "выстрел Y М5"(w411) -> ()
                "Знак перех. dX М5" <- w410
              }
              frame 6 {
                n232 = Join Numbers(hi=w425, lo=w424) -> ((hi.lo)=w420:u16)
                n233 = Join Numbers(hi=w423, lo=w422) -> ((hi.lo)=w419:u16)
                n234 = local write "выстрел X М6"(w420) -> ()
                n235 = local write "выстрел Y М6"(w419) -> ()
                "Знак перех. dX М6" <- w418
              }
              frame 7 {
                n236 = Join Numbers(hi=w433, lo=w432) -> ((hi.lo)=w428:u16)
                n237 = Join Numbers(hi=w431, lo=w430) -> ((hi.lo)=w427:u16)
                n238 = local write "выстрел X М7"(w428) -> ()
                n239 = local write "выстрел Y М7"(w427) -> ()
                "Знак перех. dX М7" <- w426
              }
              frame 8 {
                n240 = Join Numbers(hi=w441, lo=w440) -> ((hi.lo)=w436:u16)
                n241 = Join Numbers(hi=w439, lo=w438) -> ((hi.lo)=w435:u16)
                n242 = local write "выстрел X М8"(w436) -> ()
                n243 = local write "выстрел Y М8"(w435) -> ()
                "Знак перех. dX М8" <- w434
              }
              frame 9 {
                n244 = Join Numbers(hi=w449, lo=w448) -> ((hi.lo)=w444:u16)
                n245 = Join Numbers(hi=w447, lo=w446) -> ((hi.lo)=w443:u16)
                n246 = local write "выстрел X М9"(w444) -> ()
                n247 = local write "выстрел Y М9"(w443) -> ()
                "Знак перех. dX М9" <- w442
              }
              frame 10 {
                n248 = Join Numbers(hi=w457, lo=w456) -> ((hi.lo)=w452:u16)
                n249 = Join Numbers(hi=w455, lo=w454) -> ((hi.lo)=w451:u16)
                n250 = local write "выстрел X М10"(w452) -> ()
                n251 = local write "выстрел Y М10"(w451) -> ()
                "Знак перех. dX М10" <- w450
              }
            }
            n252 = property on="XY лазера" class="Bool (strict)"(error in=w359, "Visible"=TRUE) -> (error out=w376:errorcluster)  [unwired: 1 in, 1 out]
            n253 = property on="текущ. инфо" class="Bool (strict)"(error in=w376, "Visible"=TRUE) -> (error out=w362:errorcluster)  [unwired: 1 in, 1 out]
            n254 = property on="Выстрел по мишени!" class="DigNum (strict)"(error in=w362) -> (error out=w361:errorcluster, "Value"=w360:u32)  [unwired: 1 in, 1 out]
            n255 = Increment(x=w360) -> (x+1=w377:u32)
            n256 = property on="Выстрел по мишени!" class="DigNum (strict)"(error in=w361, "Val(Sgnl)"=w377) -> (error out=w358:errorcluster)  [unwired: 1 in, 1 out]
            n257 = call "Управление звуком (SubVI).vi"("Звук выстрела"="Упр. звуком", "error in (no error)"=w358) -> ("error out"=w355:errorcluster)  [unwired: 7 in]
          }
          frame 171 {
            # "Текущее положение лазера, Готовность!"
            n258 = Unbundle By Name(w459) -> ("№ мишени"=w471:u8, "Коорд. выстрела X ст.байт"=w466:u8, "Коорд. выстрела X мл.байт"=w465:u8, "Знак dX"=w464:i8, "Коорд. выстрела Y cт.байт"=w463:u8, "Коорд. выстрела Y мл.байт"=w462:u8, "выст. до перем. пленки ст. байт"=w469:u8, "выст. до перем. пленки мл. байт"=w468:u8)
            n259 = Join Numbers(hi=w469, lo=w468) -> ((hi.lo)=w473:u16)
            n260 = property on="Осталось:" class="Slide (strict)"(error in=w470, "Value"=w473) -> (error out=w467:errorcluster)  [unwired: 1 in, 1 out]
            n261 = case shown="5" w471 {
              tunnel: [w486 w498 w510 w522 w534 w546 w558 w570 w582 w594] -> w458
              tunnel: w467 -> [w481 w493 w505 w517 w529 w541 w553 w565 w577 w589]
              tunnel: w466 -> [w490 w502 w514 w526 w538 w550 w562 w574 w586 w598]
              tunnel: w465 -> [w489 w501 w513 w525 w537 w549 w561 w573 w585 w597]
              tunnel: w464 -> [w479 w491 w503 w515 w527 w539 w551 w563 w575 w587]
              tunnel: w463 -> [w488 w500 w512 w524 w536 w548 w560 w572 w584 w596]
              tunnel: w462 -> [w487 w499 w511 w523 w535 w547 w559 w571 w583 w595]
              frame 1, Default {
                n262 = Join Numbers(hi=w490, lo=w489) -> ((hi.lo)=w483:u16)
                n263 = Join Numbers(hi=w488, lo=w487) -> ((hi.lo)=w480:u16)
                n264 = local write "Знак перех. dX М1"(w479) -> ()
                n265 = control-ref of="Мишень 1"() -> (w482:refnum<vi>)
                n266 = control-ref of="XY лазера"() -> (w485:refnum<vi>)
                n267 = control-ref of="текущ. инфо"() -> (w484:refnum<vi>)
                n268 = call "Положение лазера (SubVI).vi"("Мишень reference"=w482, "XY лазера reference"=w485, "Текущ. инфо reference"=w484, "error in"=w481, "X коорд."=w483, "Y коорд."=w480) -> ("error out"=w486:errorcluster)  [unwired: 21 in]
                n269 = local write "выстрел X М1"(w483) -> ()
                n270 = local write "выстрел Y М1"(w480) -> ()
              }
              frame 2 {
                n271 = Join Numbers(hi=w502, lo=w501) -> ((hi.lo)=w495:u16)
                n272 = Join Numbers(hi=w500, lo=w499) -> ((hi.lo)=w492:u16)
                n273 = local write "Знак перех. dX М2"(w491) -> ()
                n274 = control-ref of="Мишень 2"() -> (w494:refnum<vi>)
                n275 = control-ref of="XY лазера"() -> (w497:refnum<vi>)
                n276 = control-ref of="текущ. инфо"() -> (w496:refnum<vi>)
                n277 = call "Положение лазера (SubVI).vi"("Мишень reference"=w494, "XY лазера reference"=w497, "Текущ. инфо reference"=w496, "error in"=w493, "X коорд."=w495, "Y коорд."=w492) -> ("error out"=w498:errorcluster)  [unwired: 21 in]
                n278 = local write "выстрел X М2"(w495) -> ()
                n279 = local write "выстрел Y М2"(w492) -> ()
              }
              frame 3 {
                n280 = Join Numbers(hi=w514, lo=w513) -> ((hi.lo)=w507:u16)
                n281 = Join Numbers(hi=w512, lo=w511) -> ((hi.lo)=w504:u16)
                n282 = local write "Знак перех. dX М3"(w503) -> ()
                n283 = control-ref of="Мишень 3"() -> (w506:refnum<vi>)
                n284 = control-ref of="XY лазера"() -> (w509:refnum<vi>)
                n285 = control-ref of="текущ. инфо"() -> (w508:refnum<vi>)
                n286 = call "Положение лазера (SubVI).vi"("Мишень reference"=w506, "XY лазера reference"=w509, "Текущ. инфо reference"=w508, "error in"=w505, "X коорд."=w507, "Y коорд."=w504) -> ("error out"=w510:errorcluster)  [unwired: 21 in]
                n287 = local write "выстрел X М3"(w507) -> ()
                n288 = local write "выстрел Y М3"(w504) -> ()
              }
              frame 4 {
                n289 = Join Numbers(hi=w526, lo=w525) -> ((hi.lo)=w519:u16)
                n290 = Join Numbers(hi=w524, lo=w523) -> ((hi.lo)=w516:u16)
                n291 = local write "Знак перех. dX М4"(w515) -> ()
                n292 = control-ref of="Мишень 4"() -> (w518:refnum<vi>)
                n293 = control-ref of="XY лазера"() -> (w521:refnum<vi>)
                n294 = control-ref of="текущ. инфо"() -> (w520:refnum<vi>)
                n295 = call "Положение лазера (SubVI).vi"("Мишень reference"=w518, "XY лазера reference"=w521, "Текущ. инфо reference"=w520, "error in"=w517, "X коорд."=w519, "Y коорд."=w516) -> ("error out"=w522:errorcluster)  [unwired: 21 in]
                n296 = local write "выстрел X М4"(w519) -> ()
                n297 = local write "выстрел Y М4"(w516) -> ()
              }
              frame 5 {
                n298 = Join Numbers(hi=w538, lo=w537) -> ((hi.lo)=w531:u16)
                n299 = Join Numbers(hi=w536, lo=w535) -> ((hi.lo)=w528:u16)
                n300 = local write "Знак перех. dX М5"(w527) -> ()
                n301 = control-ref of="Мишень 5"() -> (w530:refnum<vi>)
                n302 = control-ref of="XY лазера"() -> (w533:refnum<vi>)
                n303 = control-ref of="текущ. инфо"() -> (w532:refnum<vi>)
                n304 = call "Положение лазера (SubVI).vi"("Мишень reference"=w530, "XY лазера reference"=w533, "Текущ. инфо reference"=w532, "error in"=w529, "X коорд."=w531, "Y коорд."=w528) -> ("error out"=w534:errorcluster)  [unwired: 21 in]
                n305 = local write "выстрел X М5"(w531) -> ()
                n306 = local write "выстрел Y М5"(w528) -> ()
              }
              frame 6 {
                n307 = Join Numbers(hi=w550, lo=w549) -> ((hi.lo)=w543:u16)
                n308 = Join Numbers(hi=w548, lo=w547) -> ((hi.lo)=w540:u16)
                n309 = local write "Знак перех. dX М6"(w539) -> ()
                n310 = control-ref of="Мишень 6"() -> (w542:refnum<vi>)
                n311 = control-ref of="XY лазера"() -> (w545:refnum<vi>)
                n312 = control-ref of="текущ. инфо"() -> (w544:refnum<vi>)
                n313 = call "Положение лазера (SubVI).vi"("Мишень reference"=w542, "XY лазера reference"=w545, "Текущ. инфо reference"=w544, "error in"=w541, "X коорд."=w543, "Y коорд."=w540) -> ("error out"=w546:errorcluster)  [unwired: 21 in]
                n314 = local write "выстрел X М6"(w543) -> ()
                n315 = local write "выстрел Y М6"(w540) -> ()
              }
              frame 7 {
                n316 = Join Numbers(hi=w562, lo=w561) -> ((hi.lo)=w555:u16)
                n317 = Join Numbers(hi=w560, lo=w559) -> ((hi.lo)=w552:u16)
                n318 = local write "Знак перех. dX М7"(w551) -> ()
                n319 = control-ref of="Мишень 7"() -> (w554:refnum<vi>)
                n320 = control-ref of="XY лазера"() -> (w557:refnum<vi>)
                n321 = control-ref of="текущ. инфо"() -> (w556:refnum<vi>)
                n322 = call "Положение лазера (SubVI).vi"("Мишень reference"=w554, "XY лазера reference"=w557, "Текущ. инфо reference"=w556, "error in"=w553, "X коорд."=w555, "Y коорд."=w552) -> ("error out"=w558:errorcluster)  [unwired: 21 in]
                n323 = local write "выстрел X М7"(w555) -> ()
                n324 = local write "выстрел Y М7"(w552) -> ()
              }
              frame 8 {
                n325 = Join Numbers(hi=w574, lo=w573) -> ((hi.lo)=w567:u16)
                n326 = Join Numbers(hi=w572, lo=w571) -> ((hi.lo)=w564:u16)
                n327 = local write "Знак перех. dX М8"(w563) -> ()
                n328 = control-ref of="Мишень 8"() -> (w566:refnum<vi>)
                n329 = control-ref of="XY лазера"() -> (w569:refnum<vi>)
                n330 = control-ref of="текущ. инфо"() -> (w568:refnum<vi>)
                n331 = call "Положение лазера (SubVI).vi"("Мишень reference"=w566, "XY лазера reference"=w569, "Текущ. инфо reference"=w568, "error in"=w565, "X коорд."=w567, "Y коорд."=w564) -> ("error out"=w570:errorcluster)  [unwired: 21 in]
                n332 = local write "выстрел X М8"(w567) -> ()
                n333 = local write "выстрел Y М8"(w564) -> ()
              }
              frame 9 {
                n334 = Join Numbers(hi=w586, lo=w585) -> ((hi.lo)=w579:u16)
                n335 = Join Numbers(hi=w584, lo=w583) -> ((hi.lo)=w576:u16)
                n336 = local write "Знак перех. dX М9"(w575) -> ()
                n337 = control-ref of="Мишень 9"() -> (w578:refnum<vi>)
                n338 = control-ref of="XY лазера"() -> (w581:refnum<vi>)
                n339 = control-ref of="текущ. инфо"() -> (w580:refnum<vi>)
                n340 = call "Положение лазера (SubVI).vi"("Мишень reference"=w578, "XY лазера reference"=w581, "Текущ. инфо reference"=w580, "error in"=w577, "X коорд."=w579, "Y коорд."=w576) -> ("error out"=w582:errorcluster)  [unwired: 21 in]
                n341 = local write "выстрел X М9"(w579) -> ()
                n342 = local write "выстрел Y М9"(w576) -> ()
              }
              frame 10 {
                n343 = Join Numbers(hi=w598, lo=w597) -> ((hi.lo)=w591:u16)
                n344 = Join Numbers(hi=w596, lo=w595) -> ((hi.lo)=w588:u16)
                n345 = local write "Знак перех. dX М10"(w587) -> ()
                n346 = control-ref of="Мишень 10"() -> (w590:refnum<vi>)
                n347 = control-ref of="XY лазера"() -> (w593:refnum<vi>)
                n348 = control-ref of="текущ. инфо"() -> (w592:refnum<vi>)
                n349 = call "Положение лазера (SubVI).vi"("Мишень reference"=w590, "XY лазера reference"=w593, "Текущ. инфо reference"=w592, "error in"=w589, "X коорд."=w591, "Y коорд."=w588) -> ("error out"=w594:errorcluster)  [unwired: 21 in]
                n350 = local write "выстрел X М10"(w591) -> ()
                n351 = local write "выстрел Y М10"(w588) -> ()
              }
            }
            n352 = property on="XY лазера" class="Bool (strict)"("Visible"=TRUE) -> ()  [unwired: 2 in, 2 out]
            n353 = property on="Шаг вперед" class="Bool (strict)"("DisabledEnum"=u8 0 ("y")) -> ()  [unwired: 2 in, 2 out]
            n354 = property on="текущ. инфо" class="Bool (strict)"("Visible"=TRUE) -> ()  [unwired: 2 in, 2 out]
            n355 = property on="Статус" class="Bool (strict)"("Caption.Text"="Готов!" ("Label.Text")) -> (error out=w474:errorcluster)  [unwired: 2 in, 1 out]
            n356 = property on="Статус" class="Bool (strict)"(error in=w474, "Caption.Position"=T3 {"Left"=970, "Top"=-32}) -> ()  [unwired: 1 in, 2 out]
            n357 = property on="Статус" class="Bool (strict)"("Caption.TextColor"=u32 56339 ("цвет")) -> ()  [unwired: 2 in, 2 out]
          }
          frame 172 {
            # "Команда занятости"
            n358 = Unbundle By Name(w603) -> ("№ мишени"=w614:u8, "Коорд. выстрела X ст.байт"=w610:u8, "Коорд. выстрела X мл.байт"=w609:u8, "Знак dX"=w601:i8, "Коорд. выстрела Y cт.байт"=w608:u8, "Коорд. выстрела Y мл.байт"=w607:u8, "выст. до перем. пленки ст. байт"=w613:u8, "выст. до перем. пленки мл. байт"=w612:u8)
            n359 = property on="XY лазера" class="Bool (strict)"("Visible"=FALSE) -> (error out=w617:errorcluster)  [unwired: 2 in, 1 out]
            n360 = property on="текущ. инфо" class="Bool (strict)"(error in=w617, "Visible"=FALSE) -> (error out=w618:errorcluster)  [unwired: 1 in, 1 out]
            n361 = Join Numbers(hi=w613, lo=w612) -> ((hi.lo)=w615:u16)
            n362 = property on="Осталось:" class="Slide (strict)"(error in=w602, "Value"=w615) -> (error out=w611:errorcluster)  [unwired: 1 in, 1 out]
            n363 = case shown="2" w614 {
              tunnel: [w631 w643 w655 w667 w679 w691 w703 w715 w727 w739] -> w599
              tunnel: w611 -> [w628 w640 w652 w664 w676 w688 w700 w712 w724 w736]
              tunnel: w610 -> [w635 w647 w659 w671 w683 w695 w707 w719 w731 w743]
              tunnel: w609 -> [w634 w646 w658 w670 w682 w694 w706 w718 w730 w742]
              tunnel: w601 -> [w624 w636 w648 w660 w672 w684 w696 w708 w720 w732]
              tunnel: w608 -> [w633 w645 w657 w669 w681 w693 w705 w717 w729 w741]
              tunnel: w607 -> [w632 w644 w656 w668 w680 w692 w704 w716 w728 w740]
              frame 1, Default {
                n364 = Join Numbers(hi=w635, lo=w634) -> ((hi.lo)=w625:u16)
                n365 = Join Numbers(hi=w633, lo=w632) -> ((hi.lo)=w626:u16)
                n366 = local write "Знак перех. dX М1"(w624) -> ()
                n367 = control-ref of="Мишень 1"() -> (w627:refnum<vi>)
                n368 = control-ref of="XY лазера"() -> (w630:refnum<vi>)
                n369 = control-ref of="текущ. инфо"() -> (w629:refnum<vi>)
                n370 = call "Положение лазера (SubVI).vi"("Мишень reference"=w627, "XY лазера reference"=w630, "Текущ. инфо reference"=w629, "error in"=w628, "X коорд."=w625, "Y коорд."=w626) -> ("error out"=w631:errorcluster)  [unwired: 21 in]
                n371 = local write "выстрел X М1"(w625) -> ()
                n372 = local write "выстрел Y М1"(w626) -> ()
              }
              frame 2 {
                n373 = Join Numbers(hi=w647, lo=w646) -> ((hi.lo)=w637:u16)
                n374 = Join Numbers(hi=w645, lo=w644) -> ((hi.lo)=w638:u16)
                n375 = local write "Знак перех. dX М2"(w636) -> ()
                n376 = control-ref of="Мишень 2"() -> (w639:refnum<vi>)
                n377 = control-ref of="XY лазера"() -> (w642:refnum<vi>)
                n378 = control-ref of="текущ. инфо"() -> (w641:refnum<vi>)
                n379 = call "Положение лазера (SubVI).vi"("Мишень reference"=w639, "XY лазера reference"=w642, "Текущ. инфо reference"=w641, "error in"=w640, "X коорд."=w637, "Y коорд."=w638) -> ("error out"=w643:errorcluster)  [unwired: 21 in]
                n380 = local write "выстрел X М2"(w637) -> ()
                n381 = local write "выстрел Y М2"(w638) -> ()
              }
              frame 3 {
                n382 = Join Numbers(hi=w659, lo=w658) -> ((hi.lo)=w649:u16)
                n383 = Join Numbers(hi=w657, lo=w656) -> ((hi.lo)=w650:u16)
                n384 = local write "Знак перех. dX М3"(w648) -> ()
                n385 = control-ref of="Мишень 3"() -> (w651:refnum<vi>)
                n386 = control-ref of="XY лазера"() -> (w654:refnum<vi>)
                n387 = control-ref of="текущ. инфо"() -> (w653:refnum<vi>)
                n388 = call "Положение лазера (SubVI).vi"("Мишень reference"=w651, "XY лазера reference"=w654, "Текущ. инфо reference"=w653, "error in"=w652, "X коорд."=w649, "Y коорд."=w650) -> ("error out"=w655:errorcluster)  [unwired: 21 in]
                n389 = local write "выстрел X М3"(w649) -> ()
                n390 = local write "выстрел Y М3"(w650) -> ()
              }
              frame 4 {
                n391 = Join Numbers(hi=w671, lo=w670) -> ((hi.lo)=w661:u16)
                n392 = Join Numbers(hi=w669, lo=w668) -> ((hi.lo)=w662:u16)
                n393 = local write "Знак перех. dX М4"(w660) -> ()
                n394 = control-ref of="Мишень 4"() -> (w663:refnum<vi>)
                n395 = control-ref of="XY лазера"() -> (w666:refnum<vi>)
                n396 = control-ref of="текущ. инфо"() -> (w665:refnum<vi>)
                n397 = call "Положение лазера (SubVI).vi"("Мишень reference"=w663, "XY лазера reference"=w666, "Текущ. инфо reference"=w665, "error in"=w664, "X коорд."=w661, "Y коорд."=w662) -> ("error out"=w667:errorcluster)  [unwired: 21 in]
                n398 = local write "выстрел X М4"(w661) -> ()
                n399 = local write "выстрел Y М4"(w662) -> ()
              }
              frame 5 {
                n400 = Join Numbers(hi=w683, lo=w682) -> ((hi.lo)=w673:u16)
                n401 = Join Numbers(hi=w681, lo=w680) -> ((hi.lo)=w674:u16)
                n402 = local write "Знак перех. dX М5"(w672) -> ()
                n403 = control-ref of="Мишень 5"() -> (w675:refnum<vi>)
                n404 = control-ref of="XY лазера"() -> (w678:refnum<vi>)
                n405 = control-ref of="текущ. инфо"() -> (w677:refnum<vi>)
                n406 = call "Положение лазера (SubVI).vi"("Мишень reference"=w675, "XY лазера reference"=w678, "Текущ. инфо reference"=w677, "error in"=w676, "X коорд."=w673, "Y коорд."=w674) -> ("error out"=w679:errorcluster)  [unwired: 21 in]
                n407 = local write "выстрел X М5"(w673) -> ()
                n408 = local write "выстрел Y М5"(w674) -> ()
              }
              frame 6 {
                n409 = Join Numbers(hi=w695, lo=w694) -> ((hi.lo)=w685:u16)
                n410 = Join Numbers(hi=w693, lo=w692) -> ((hi.lo)=w686:u16)
                n411 = local write "Знак перех. dX М6"(w684) -> ()
                n412 = control-ref of="Мишень 6"() -> (w687:refnum<vi>)
                n413 = control-ref of="XY лазера"() -> (w690:refnum<vi>)
                n414 = control-ref of="текущ. инфо"() -> (w689:refnum<vi>)
                n415 = call "Положение лазера (SubVI).vi"("Мишень reference"=w687, "XY лазера reference"=w690, "Текущ. инфо reference"=w689, "error in"=w688, "X коорд."=w685, "Y коорд."=w686) -> ("error out"=w691:errorcluster)  [unwired: 21 in]
                n416 = local write "выстрел X М6"(w685) -> ()
                n417 = local write "выстрел Y М6"(w686) -> ()
              }
              frame 7 {
                n418 = Join Numbers(hi=w707, lo=w706) -> ((hi.lo)=w697:u16)
                n419 = Join Numbers(hi=w705, lo=w704) -> ((hi.lo)=w698:u16)
                n420 = local write "Знак перех. dX М7"(w696) -> ()
                n421 = control-ref of="Мишень 7"() -> (w699:refnum<vi>)
                n422 = control-ref of="XY лазера"() -> (w702:refnum<vi>)
                n423 = control-ref of="текущ. инфо"() -> (w701:refnum<vi>)
                n424 = call "Положение лазера (SubVI).vi"("Мишень reference"=w699, "XY лазера reference"=w702, "Текущ. инфо reference"=w701, "error in"=w700, "X коорд."=w697, "Y коорд."=w698) -> ("error out"=w703:errorcluster)  [unwired: 21 in]
                n425 = local write "выстрел X М7"(w697) -> ()
                n426 = local write "выстрел Y М7"(w698) -> ()
              }
              frame 8 {
                n427 = Join Numbers(hi=w719, lo=w718) -> ((hi.lo)=w709:u16)
                n428 = Join Numbers(hi=w717, lo=w716) -> ((hi.lo)=w710:u16)
                n429 = local write "Знак перех. dX М8"(w708) -> ()
                n430 = control-ref of="Мишень 8"() -> (w711:refnum<vi>)
                n431 = control-ref of="XY лазера"() -> (w714:refnum<vi>)
                n432 = control-ref of="текущ. инфо"() -> (w713:refnum<vi>)
                n433 = call "Положение лазера (SubVI).vi"("Мишень reference"=w711, "XY лазера reference"=w714, "Текущ. инфо reference"=w713, "error in"=w712, "X коорд."=w709, "Y коорд."=w710) -> ("error out"=w715:errorcluster)  [unwired: 21 in]
                n434 = local write "выстрел X М8"(w709) -> ()
                n435 = local write "выстрел Y М8"(w710) -> ()
              }
              frame 9 {
                n436 = Join Numbers(hi=w731, lo=w730) -> ((hi.lo)=w721:u16)
                n437 = Join Numbers(hi=w729, lo=w728) -> ((hi.lo)=w722:u16)
                n438 = local write "Знак перех. dX М9"(w720) -> ()
                n439 = control-ref of="Мишень 9"() -> (w723:refnum<vi>)
                n440 = control-ref of="XY лазера"() -> (w726:refnum<vi>)
                n441 = control-ref of="текущ. инфо"() -> (w725:refnum<vi>)
                n442 = call "Положение лазера (SubVI).vi"("Мишень reference"=w723, "XY лазера reference"=w726, "Текущ. инфо reference"=w725, "error in"=w724, "X коорд."=w721, "Y коорд."=w722) -> ("error out"=w727:errorcluster)  [unwired: 21 in]
                n443 = local write "выстрел X М9"(w721) -> ()
                n444 = local write "выстрел Y М9"(w722) -> ()
              }
              frame 10 {
                n445 = Join Numbers(hi=w743, lo=w742) -> ((hi.lo)=w733:u16)
                n446 = Join Numbers(hi=w741, lo=w740) -> ((hi.lo)=w734:u16)
                n447 = local write "Знак перех. dX М10"(w732) -> ()
                n448 = control-ref of="Мишень 10"() -> (w735:refnum<vi>)
                n449 = control-ref of="XY лазера"() -> (w738:refnum<vi>)
                n450 = control-ref of="текущ. инфо"() -> (w737:refnum<vi>)
                n451 = call "Положение лазера (SubVI).vi"("Мишень reference"=w735, "XY лазера reference"=w738, "Текущ. инфо reference"=w737, "error in"=w736, "X коорд."=w733, "Y коорд."=w734) -> ("error out"=w739:errorcluster)  [unwired: 21 in]
                n452 = local write "выстрел X М10"(w733) -> ()
                n453 = local write "выстрел Y М10"(w734) -> ()
              }
            }
            n454 = property on="Статус" class="Bool (strict)"(error in=w618, "Visible"=TRUE) -> (error out=w604:errorcluster)  [unwired: 1 in, 1 out]
            n455 = property on="Статус" class="Bool (strict)"(error in=w604, "Caption.Text"="Идет перемещение..." ("Label.Text")) -> (error out=w605:errorcluster)  [unwired: 1 in, 1 out]
            n456 = property on="Статус" class="Bool (strict)"(error in=w605, "Caption.TextColor"=u32 16711680 ("цвет")) -> (error out=w606:errorcluster)  [unwired: 1 in, 1 out]
            n457 = property on="Статус" class="Bool (strict)"(error in=w606, "Caption.Position"=T3 {"Left"=800, "Top"=-32}) -> ()  [unwired: 1 in, 2 out]
          }
          frame 199 {
            # "Команда \"Блок на связи, режим ожидания\""
          }
        }
        n458 = Join Numbers(hi=w188, lo=w187) -> ((hi.lo)=w184:u16)
        n459 = case "Вывод ифн. об оставшися выстрелах в текущую точку" shown="10" w186 {
          tunnel: w184 -> [w744 w745 w746 w747 w748 w749 w750 w751 w752 w753 _]
          tunnel: [w744 w745 w746 w747 w748 w749 w750 w751 w752 w753 _] -> w185
          frame 1 {
            n460 = property on="Выстрелов осталось M1" class="DigNum (strict)"("Value"=w744) -> ()  [unwired: 2 in, 2 out]
          }
          frame 2 {
            n461 = property on="Выстрелов осталось M2" class="DigNum (strict)"("Value"=w745) -> ()  [unwired: 2 in, 2 out]
          }
          frame 3 {
            n462 = property on="Выстрелов осталось M3" class="DigNum (strict)"("Value"=w746) -> ()  [unwired: 2 in, 2 out]
          }
          frame 4 {
            n463 = property on="Выстрелов осталось M4" class="DigNum (strict)"("Value"=w747) -> ()  [unwired: 2 in, 2 out]
          }
          frame 5 {
            n464 = property on="Выстрелов осталось M5" class="DigNum (strict)"("Value"=w748) -> ()  [unwired: 2 in, 2 out]
          }
          frame 6 {
            n465 = property on="Выстрелов осталось M6" class="DigNum (strict)"("Value"=w749) -> ()  [unwired: 2 in, 2 out]
          }
          frame 7 {
            n466 = property on="Выстрелов осталось M7" class="DigNum (strict)"("Value"=w750) -> ()  [unwired: 2 in, 2 out]
          }
          frame 8 {
            n467 = property on="Выстрелов осталось M8" class="DigNum (strict)"("Value"=w751) -> ()  [unwired: 2 in, 2 out]
          }
          frame 9 {
            n468 = property on="Выстрелов осталось M9" class="DigNum (strict)"("Value"=w752) -> ()  [unwired: 2 in, 2 out]
          }
          frame 10 {
            n469 = property on="Выстрелов осталось M10" class="DigNum (strict)"("Value"=w753) -> ()  [unwired: 2 in, 2 out]
          }
          frame 11, Default {
          }
        }
        n470 = Not Equal To 0?(x=w185) -> (x != 0?=w183:bool)
        n471 = case shown="True" w183 {
          tunnel: w185 -> [_ w205]
          frame False {
          }
          frame True {
            n472 = Number To Decimal String(number=w205) -> (decimal integer string=w204:string)  [unwired: 1 in]
            n473 = property on="текущ. инфо" class="Bool (strict)"("Caption.Text"=w204) -> ()  [unwired: 2 in, 2 out]
          }
        }
        n474 = case shown="True" w189 {
          tunnel: [w198 w203] -> w197
          tunnel: w192 -> [w198 w200]
          tunnel: w191 -> [_ w199]
          frame False {
          }
          frame True {
            n475 = property on="TCP con ID" class="Ref (strict)"(error in=w200) -> (error out=w202:errorcluster, "Value"=w201:refnum<k5>)  [unwired: 1 in, 1 out]
            n476 = call "Передать кластер параметров в TCP (SubVI).vi"("Кластер параметров мишени"=w199, "error in"=w202, "TCP connection ID"=w201) -> ("error out"=w203:errorcluster)  [unwired: 11 in, 1 out]
          }
        }
      }
      event "Выстрел по мишени!": Value Change {
        # "Отрисовка точек на мишенях"
        n477 = event-data() -> ()  [unwired: 2 out]
        n478 = property on="id мишени" class="DigNum (strict)"(error in=w761) -> (error out=w763:errorcluster, "Value"=w766:u16)  [unwired: 1 in, 1 out]
        n479 = case "Считывание состояния \n  мишени до выстрела" shown="7" w766 {
          selector: w766 -> [w821 w826 w831 w836 w841 w846 w851 w856 w861 w866]
          tunnel: ["выстрел Y М1" "выстрел Y М2" "выстрел Y М3" "выстрел Y М4" "выстрел Y М5" "выстрел Y М6" "выстрел Y М7" "выстрел Y М8" "выстрел Y М9" "выстрел Y М10"] -> w759
          tunnel: ["выстрел X М1" "выстрел X М2" "выстрел X М3" "выстрел X М4" "выстрел X М5" "выстрел X М6" "выстрел X М7" "выстрел X М8" "выстрел X М9" "выстрел X М10"] -> w760
          tunnel: [w821 w826 w831 w836 w841 w846 w851 w856 w861 w866] -> w758
          tunnel: w763 -> [w820 w825 w830 w835 w840 w845 w850 w855 w860 w865]
          tunnel: [w820 w825 w830 w835 w840 w845 w850 w855 w860 w865] -> w762
          tunnel: ["Мишень 1" "Мишень 2" "Мишень 3" "Мишень 4" "Мишень 5" "Мишень 6" "Мишень 7" "Мишень 8" "Мишень 9" "Мишень 10"] -> w756
          frame 1, Default {
          }
          frame 2 {
          }
          frame 3 {
          }
          frame 4 {
          }
          frame 5 {
          }
          frame 6 {
          }
          frame 7 {
          }
          frame 8 {
          }
          frame 9 {
          }
          frame 10 {
          }
        }
        n480 = call "Добавить точку на рисунок (SubVI).vi"("in picture"=w756, "id мишени вх"=w758, "цвет"=u32 16777222, "error in"=w762, "dot х"=w760, "dot y"=w759) -> ("error out"=w765:errorcluster, "id мишени вых"=w757:u16, "out picture"=w764:picture)  [unwired: 11 in]
        n481 = case "Обновление мишени при выстреле" shown="1, Default" w757 {
          tunnel: w760 -> [w771 w776 w781 w785 w790 w795 w800 w805 w810 w815]
          tunnel: w759 -> [w770 w775 w780 w786 w791 w796 w801 w806 w811 w816]
          tunnel: w765 -> [w769 w774 w779 w783 w789 w794 w799 w804 w809 w814]
          tunnel: w764 -> [w767 w772 w777 w784 w787 w792 w797 w802 w807 w812]
          tunnel: [w768 w773 w778 w782 w788 w793 w798 w803 w808 w813] -> w755
          frame 1, Default {
            n482 = local write "выстрел X М1"(w771) -> ()
            n483 = property on="Мишень 1" class="Pict"(error in=w769, "Value"=w767) -> (error out=w768:errorcluster)  [unwired: 1 in, 1 out]
            n484 = local write "выстрел Y М1"(w770) -> ()
          }
          frame 2 {
            n485 = property on="Мишень 2" class="Pict"(error in=w774, "Value"=w772) -> (error out=w773:errorcluster)  [unwired: 1 in, 1 out]
            n486 = local write "выстрел X М2"(w776) -> ()
            n487 = local write "выстрел Y М2"(w775) -> ()
          }
          frame 3 {
            n488 = local write "выстрел X М3"(w781) -> ()
            n489 = property on="Мишень 3" class="Pict"(error in=w779, "Value"=w777) -> (error out=w778:errorcluster)  [unwired: 1 in, 1 out]
            n490 = local write "выстрел Y М3"(w780) -> ()
          }
          frame 4 {
            n491 = local write "выстрел X М4"(w785) -> ()
            n492 = property on="Мишень 4" class="Pict"(error in=w783, "Value"=w784) -> (error out=w782:errorcluster)  [unwired: 1 in, 1 out]
            n493 = local write "выстрел Y М4"(w786) -> ()
          }
          frame 5 {
            n494 = local write "выстрел X М5"(w790) -> ()
            n495 = local write "выстрел Y М5"(w791) -> ()
            n496 = property on="Мишень 5" class="Pict"(error in=w789, "Value"=w787) -> (error out=w788:errorcluster)  [unwired: 1 in, 1 out]
          }
          frame 6 {
            n497 = local write "выстрел X М6"(w795) -> ()
            n498 = local write "выстрел Y М6"(w796) -> ()
            n499 = property on="Мишень 6" class="Pict"(error in=w794, "Value"=w792) -> (error out=w793:errorcluster)  [unwired: 1 in, 1 out]
          }
          frame 7 {
            n500 = local write "выстрел X М7"(w800) -> ()
            n501 = local write "выстрел Y М7"(w801) -> ()
            n502 = property on="Мишень 7" class="Pict"(error in=w799, "Value"=w797) -> (error out=w798:errorcluster)  [unwired: 1 in, 1 out]
          }
          frame 8 {
            n503 = local write "выстрел X М8"(w805) -> ()
            n504 = local write "выстрел Y М8"(w806) -> ()
            n505 = property on="Мишень 8" class="Pict"(error in=w804, "Value"=w802) -> (error out=w803:errorcluster)  [unwired: 1 in, 1 out]
          }
          frame 9 {
            n506 = local write "выстрел X М9"(w810) -> ()
            n507 = local write "выстрел Y М9"(w811) -> ()
            n508 = property on="Мишень 9" class="Pict"(error in=w809, "Value"=w807) -> (error out=w808:errorcluster)  [unwired: 1 in, 1 out]
          }
          frame 10 {
            n509 = local write "выстрел X М10"(w815) -> ()
            n510 = local write "выстрел Y М10"(w816) -> ()
            n511 = property on="Мишень 10" class="Pict"(error in=w814, "Value"=w812) -> (error out=w813:errorcluster)  [unwired: 1 in, 1 out]
          }
        }
      }
      event Mouse Move {
        # "Работа с курсором - линейка"
        n512 = event-data() -> ()  [unwired: 2 out]
        n513 = control-ref of="This VI"() -> (w873:refnum<vi>)
        n514 = call "Линейка (SubVI).vi"("Mouse ID in"=w872, "VI reference"=w873, "error in (no error)"=w871) -> ("Mouse ID out"=w870:refnum<k1>, "Slide Horizontal"=→"Slide X axis":u8, "Slide Vertical"=→"Slide Y axis":u8, "error out"=w868:errorcluster)  [unwired: 13 in]
        n515 = local read "Выстрелов до перемотки пленки"() -> (w869:u16)
        n516 = property on="Осталось:" class="Slide (strict)"(error in=w868, "Scale.Maximum"=w869) -> (error out=w867:errorcluster)  [unwired: 1 in, 1 out]
      }
      event "Добавить мишень": Value Change {
        n517 = event-data() -> ("OldVal"=w880:bool)  [unwired: 1 out]
        n518 = property on="Добавить мишень" class="Bool (strict)"(error in=w881, "Value"=w880) -> (error out=w879:errorcluster)  [unwired: 1 in, 1 out]
        n519 = property on="Счетчик мишеней" class="DigNum (strict)"(error in=w879) -> (error out=w883:errorcluster, "Value"=w876:u8)  [unwired: 1 in, 1 out]
        n520 = Increment(x=w876) -> (x+1=w884:u8)
        "Счетчик мишеней" <- w884
        n521 = Greater Or Equal?(x=w876, y=u8 10) -> (x >= y?=w877:bool)
        n522 = case shown="True" w877 {
          frame False {
          }
          frame True {
            n523 = property on="Добавить мишень" class="Bool (strict)"("DisabledEnum"=T2."Disabled and Grayed Out" ("Disabled")) -> ()  [unwired: 2 in, 2 out]
          }
        }
        n524 = case shown="1" w884 {
          tunnel: w883 -> [w886 w889 w890 w893 w896 w899 w902 w905 w908 w911 w914]
          tunnel: [w886 w887 w891 w895 w898 w900 w903 w906 w909 w912 w915] -> w882
          frame 0, Default {
          }
          frame 1 {
            n525 = property on="Мишень 1" class="Pict"(error in=w889, "Visible"=TRUE) -> (error out=w887:errorcluster)  [unwired: 1 in, 1 out]
          }
          frame 2 {
            n526 = property on="Мишень 2" class="Pict"(error in=w890, "Visible"=TRUE) -> (error out=w891:errorcluster)  [unwired: 1 in, 1 out]
          }
          frame 3 {
            n527 = property on="Мишень 3" class="Pict"(error in=w893, "Visible"=TRUE) -> (error out=w895:errorcluster)  [unwired: 1 in, 1 out]
          }
          frame 4 {
            n528 = property on="Мишень 4" class="Pict"(error in=w896, "Visible"=TRUE) -> (error out=w898:errorcluster)  [unwired: 1 in, 1 out]
          }
          frame 5 {
            n529 = property on="Мишень 5" class="Pict"(error in=w899, "Visible"=TRUE) -> (error out=w900:errorcluster)  [unwired: 1 in, 1 out]
          }
          frame 6 {
            n530 = property on="Мишень 6" class="Pict"(error in=w902, "Visible"=TRUE) -> (error out=w903:errorcluster)  [unwired: 1 in, 1 out]
          }
          frame 7 {
            n531 = property on="Мишень 7" class="Pict"(error in=w905, "Visible"=TRUE) -> (error out=w906:errorcluster)  [unwired: 1 in, 1 out]
          }
          frame 8 {
            n532 = property on="Мишень 8" class="Pict"(error in=w908, "Visible"=TRUE) -> (error out=w909:errorcluster)  [unwired: 1 in, 1 out]
          }
          frame 9 {
            n533 = property on="Мишень 9" class="Pict"(error in=w911, "Visible"=TRUE) -> (error out=w912:errorcluster)  [unwired: 1 in, 1 out]
          }
          frame 10 {
            n534 = property on="Мишень 10" class="Pict"(error in=w914, "Visible"=TRUE) -> (error out=w915:errorcluster)  [unwired: 1 in, 1 out]
          }
        }
      }
      event "Мишень 1": Shortcut Menu Selection (User) {
        n535 = event-data() -> ("ItemTag"=w919:string)  [unwired: 1 out]
        n536 = case shown="\"Выбрать\"" w919 {
          tunnel: [w925 w933] -> w917
          tunnel: w918 -> [w920 w932]
          frame "Настроить", Default {
            n537 = call "Настройки мишени (Sub VI).vi"("Параметры мишеней вх"="М1", "error in"=w920) -> ("Параметры мишеней вых"=w924:T1, "error out"=w926:errorcluster)  [unwired: 16 in]
            n538 = Unbundle(w924) -> ("Название мишени"=w923:string, "Х0_position"=w931:u16, "Y0_position"=w930:u16, "Длина, мм"=w929:u16, "Ширина, мм"=w928:u16)  [unwired: 5 out]
            n539 = property on="М1" class="Clust (strict)"(error in=w926, "Val(Sgnl)"=w924) -> (error out=w925:errorcluster)  [unwired: 1 in, 1 out]
            n540 = Bundle("Х0_position"=w931, "Y0_position"=w930) -> (w922:cluster{"Х0_position":u16, "Y0_position":u16})  [unwired: 1 in]
            n541 = Bundle("Длина, мм"=w929, "Ширина, мм"=w928) -> (w921:cluster{"Длина, мм":u16, "Ширина, мм":u16})  [unwired: 1 in]
            n542 = property on="Мишень 1" class="Pict"("TipStrip"=w923) -> ()  [unwired: 2 in, 2 out]
            n543 = property on="Мишень 1" class="Pict"("Position"=w922) -> ()  [unwired: 2 in, 2 out]
            n544 = property on="Мишень 1" class="Pict"("Draw Area Size"=w921) -> ()  [unwired: 2 in, 2 out]
          }
          frame "Выбрать" {
            n545 = Two Button Dialog(message="Вы уверены, что хотите выбрать эту мишень?", 1:"Нет" ("F button name (\"Cancel\")"), 2:"Да" ("T button name (\"OK\")")) -> (T button?=w934:bool)
            n546 = case shown="True" w934 {
              tunnel: [w938 w940] -> w933
              tunnel: w932 -> [w938 w939]
              frame False {
              }
              frame True {
                w941 = u16 1 ("id мишени")
                n547 = property on="id мишени" class="DigNum (strict)"(error in=w939, "Value"=w941) -> (error out=w942:errorcluster)  [unwired: 1 in, 1 out]
                n548 = property on="id мишени" class="DigNum (strict)"(error in=w942, "Val(Sgnl)"=w941) -> (error out=w940:errorcluster)  [unwired: 1 in, 1 out]
              }
            }
          }
        }
      }
      event "Мишень 2": Shortcut Menu Selection (User) {
        n549 = event-data() -> ("ItemTag"=w945:string)  [unwired: 1 out]
        n550 = case shown="\"Настроить\", Default" w945 {
          tunnel: w943 -> [w953 w960]
          tunnel: [w947 w959] -> w944
          frame "Настроить", Default {
            n551 = call "Настройки мишени (Sub VI).vi"("Параметры мишеней вх"="М2", "error in"=w953) -> ("Параметры мишеней вых"=w948:T1, "error out"=w949:errorcluster)  [unwired: 16 in]
            n552 = Unbundle(w948) -> ("Название мишени"=w952:string, "Х0_position"=w957:u16, "Y0_position"=w956:u16, "Длина, мм"=w955:u16, "Ширина, мм"=w954:u16)  [unwired: 5 out]
            n553 = property on="М2" class="Clust (strict)"(error in=w949, "Val(Sgnl)"=w948) -> (error out=w947:errorcluster)  [unwired: 1 in, 1 out]
            n554 = Bundle("Х0_position"=w957, "Y0_position"=w956) -> (w951:cluster{"Х0_position":u16, "Y0_position":u16})  [unwired: 1 in]
            n555 = Bundle("Длина, мм"=w955, "Ширина, мм"=w954) -> (w950:cluster{"Длина, мм":u16, "Ширина, мм":u16})  [unwired: 1 in]
            n556 = property on="Мишень 2" class="Pict"("TipStrip"=w952) -> ()  [unwired: 2 in, 2 out]
            n557 = property on="Мишень 2" class="Pict"("Position"=w951) -> ()  [unwired: 2 in, 2 out]
            n558 = property on="Мишень 2" class="Pict"("Draw Area Size"=w950) -> ()  [unwired: 2 in, 2 out]
          }
          frame "Выбрать" {
            n559 = Two Button Dialog(message="Вы уверены, что хотите выбрать эту мишень?", 1:"Нет" ("F button name (\"Cancel\")"), 2:"Да" ("T button name (\"OK\")")) -> (T button?=w963:bool)
            n560 = case shown="True" w963 {
              tunnel: [w964 w966] -> w959
              tunnel: w960 -> [w964 w965]
              frame False {
              }
              frame True {
                w967 = u16 2 ("id мишени")
                n561 = property on="id мишени" class="DigNum (strict)"(error in=w965, "Value"=w967) -> (error out=w968:errorcluster)  [unwired: 1 in, 1 out]
                n562 = property on="id мишени" class="DigNum (strict)"(error in=w968, "Val(Sgnl)"=w967) -> (error out=w966:errorcluster)  [unwired: 1 in, 1 out]
              }
            }
          }
        }
      }
      event "Мишень 3": Shortcut Menu Selection (User) {
        n563 = event-data() -> ("ItemTag"=w971:string)  [unwired: 1 out]
        n564 = case shown="\"Настроить\", Default" w971 {
          tunnel: w969 -> [w979 w986]
          tunnel: [w972 w985] -> w970
          frame "Настроить", Default {
            n565 = call "Настройки мишени (Sub VI).vi"("Параметры мишеней вх"="М3", "error in"=w979) -> ("Параметры мишеней вых"=w973:T1, "error out"=w974:errorcluster)  [unwired: 16 in]
            n566 = Unbundle(w973) -> ("Название мишени"=w978:string, "Х0_position"=w983:u16, "Y0_position"=w982:u16, "Длина, мм"=w981:u16, "Ширина, мм"=w980:u16)  [unwired: 5 out]
            n567 = property on="М3" class="Clust (strict)"(error in=w974, "Val(Sgnl)"=w973) -> (error out=w972:errorcluster)  [unwired: 1 in, 1 out]
            n568 = Bundle("Х0_position"=w983, "Y0_position"=w982) -> (w977:cluster{"Х0_position":u16, "Y0_position":u16})  [unwired: 1 in]
            n569 = Bundle("Длина, мм"=w981, "Ширина, мм"=w980) -> (w976:cluster{"Длина, мм":u16, "Ширина, мм":u16})  [unwired: 1 in]
            n570 = property on="Мишень 3" class="Pict"("TipStrip"=w978) -> ()  [unwired: 2 in, 2 out]
            n571 = property on="Мишень 3" class="Pict"("Position"=w977) -> ()  [unwired: 2 in, 2 out]
            n572 = property on="Мишень 3" class="Pict"("Draw Area Size"=w976) -> ()  [unwired: 2 in, 2 out]
          }
          frame "Выбрать" {
            n573 = Two Button Dialog(message="Вы уверены, что хотите выбрать эту мишень?", 1:"Нет" ("F button name (\"Cancel\")"), 2:"Да" ("T button name (\"OK\")")) -> (T button?=w989:bool)
            n574 = case shown="True" w989 {
              tunnel: [w990 w992] -> w985
              tunnel: w986 -> [w990 w991]
              frame False {
              }
              frame True {
                w993 = u16 3 ("id мишени")
                n575 = property on="id мишени" class="DigNum (strict)"(error in=w991, "Value"=w993) -> (error out=w994:errorcluster)  [unwired: 1 in, 1 out]
                n576 = property on="id мишени" class="DigNum (strict)"(error in=w994, "Val(Sgnl)"=w993) -> (error out=w992:errorcluster)  [unwired: 1 in, 1 out]
              }
            }
          }
        }
      }
      event "Мишень 4": Shortcut Menu Selection (User) {
        n577 = event-data() -> ("ItemTag"=w997:string)  [unwired: 1 out]
        n578 = case shown="\"Настроить\", Default" w997 {
          tunnel: w995 -> [w1005 w1010]
          tunnel: [w998 w1011] -> w996
          frame "Настроить", Default {
            n579 = call "Настройки мишени (Sub VI).vi"("Параметры мишеней вх"="М4", "error in"=w1005) -> ("Параметры мишеней вых"=w999:T1, "error out"=w1000:errorcluster)  [unwired: 16 in]
            n580 = Unbundle(w999) -> ("Название мишени"=w1004:string, "Х0_position"=w1009:u16, "Y0_position"=w1008:u16, "Длина, мм"=w1007:u16, "Ширина, мм"=w1006:u16)  [unwired: 5 out]
            n581 = property on="М4" class="Clust (strict)"(error in=w1000, "Val(Sgnl)"=w999) -> (error out=w998:errorcluster)  [unwired: 1 in, 1 out]
            n582 = Bundle("Х0_position"=w1009, "Y0_position"=w1008) -> (w1003:cluster{"Х0_position":u16, "Y0_position":u16})  [unwired: 1 in]
            n583 = Bundle("Длина, мм"=w1007, "Ширина, мм"=w1006) -> (w1002:cluster{"Длина, мм":u16, "Ширина, мм":u16})  [unwired: 1 in]
            n584 = property on="Мишень 4" class="Pict"("TipStrip"=w1004) -> ()  [unwired: 2 in, 2 out]
            n585 = property on="Мишень 4" class="Pict"("Position"=w1003) -> ()  [unwired: 2 in, 2 out]
            n586 = property on="Мишень 4" class="Pict"("Draw Area Size"=w1002) -> ()  [unwired: 2 in, 2 out]
          }
          frame "Выбрать" {
            n587 = Two Button Dialog(message="Вы уверены, что хотите выбрать эту мишень?", 1:"Нет" ("F button name (\"Cancel\")"), 2:"Да" ("T button name (\"OK\")")) -> (T button?=w1015:bool)
            n588 = case shown="True" w1015 {
              tunnel: [w1016 w1018] -> w1011
              tunnel: w1010 -> [w1016 w1017]
              frame False {
              }
              frame True {
                w1019 = u16 4 ("id мишени")
                n589 = property on="id мишени" class="DigNum (strict)"(error in=w1017, "Value"=w1019) -> (error out=w1020:errorcluster)  [unwired: 1 in, 1 out]
                n590 = property on="id мишени" class="DigNum (strict)"(error in=w1020, "Val(Sgnl)"=w1019) -> (error out=w1018:errorcluster)  [unwired: 1 in, 1 out]
              }
            }
          }
        }
      }
      event "Мишень 5": Shortcut Menu Selection (User) {
        n591 = event-data() -> ("ItemTag"=w1023:string)  [unwired: 1 out]
        n592 = case shown="\"Настроить\", Default" w1023 {
          tunnel: w1021 -> [w1031 w1037]
          tunnel: [w1024 w1036] -> w1022
          frame "Настроить", Default {
            n593 = call "Настройки мишени (Sub VI).vi"("Параметры мишеней вх"="М5", "error in"=w1031) -> ("Параметры мишеней вых"=w1025:T1, "error out"=w1026:errorcluster)  [unwired: 16 in]
            n594 = Unbundle(w1025) -> ("Название мишени"=w1030:string, "Х0_position"=w1035:u16, "Y0_position"=w1034:u16, "Длина, мм"=w1033:u16, "Ширина, мм"=w1032:u16)  [unwired: 5 out]
            n595 = property on="М5" class="Clust (strict)"(error in=w1026, "Val(Sgnl)"=w1025) -> (error out=w1024:errorcluster)  [unwired: 1 in, 1 out]
            n596 = Bundle("Х0_position"=w1035, "Y0_position"=w1034) -> (w1029:cluster{"Х0_position":u16, "Y0_position":u16})  [unwired: 1 in]
            n597 = Bundle("Длина, мм"=w1033, "Ширина, мм"=w1032) -> (w1028:cluster{"Длина, мм":u16, "Ширина, мм":u16})  [unwired: 1 in]
            n598 = property on="Мишень 5" class="Pict"("TipStrip"=w1030) -> ()  [unwired: 2 in, 2 out]
            n599 = property on="Мишень 5" class="Pict"("Position"=w1029) -> ()  [unwired: 2 in, 2 out]
            n600 = property on="Мишень 5" class="Pict"("Draw Area Size"=w1028) -> ()  [unwired: 2 in, 2 out]
          }
          frame "Выбрать" {
            n601 = Two Button Dialog(message="Вы уверены, что хотите выбрать эту мишень?", 1:"Нет" ("F button name (\"Cancel\")"), 2:"Да" ("T button name (\"OK\")")) -> (T button?=w1041:bool)
            n602 = case shown="True" w1041 {
              tunnel: [w1042 w1044] -> w1036
              tunnel: w1037 -> [w1042 w1043]
              frame False {
              }
              frame True {
                w1045 = u16 5 ("id мишени")
                n603 = property on="id мишени" class="DigNum (strict)"(error in=w1043, "Value"=w1045) -> (error out=w1046:errorcluster)  [unwired: 1 in, 1 out]
                n604 = property on="id мишени" class="DigNum (strict)"(error in=w1046, "Val(Sgnl)"=w1045) -> (error out=w1044:errorcluster)  [unwired: 1 in, 1 out]
              }
            }
          }
        }
      }
      event "Мишень 6": Shortcut Menu Selection (User) {
        n605 = event-data() -> ("ItemTag"=w1049:string)  [unwired: 1 out]
        n606 = case shown="\"Настроить\", Default" w1049 {
          tunnel: w1047 -> [w1057 w1063]
          tunnel: [w1050 w1062] -> w1048
          frame "Настроить", Default {
            n607 = call "Настройки мишени (Sub VI).vi"("Параметры мишеней вх"="М6", "error in"=w1057) -> ("Параметры мишеней вых"=w1051:T1, "error out"=w1052:errorcluster)  [unwired: 16 in]
            n608 = Unbundle(w1051) -> ("Название мишени"=w1056:string, "Х0_position"=w1061:u16, "Y0_position"=w1060:u16, "Длина, мм"=w1059:u16, "Ширина, мм"=w1058:u16)  [unwired: 5 out]
            n609 = property on="М6" class="Clust (strict)"(error in=w1052, "Val(Sgnl)"=w1051) -> (error out=w1050:errorcluster)  [unwired: 1 in, 1 out]
            n610 = Bundle("Х0_position"=w1061, "Y0_position"=w1060) -> (w1055:cluster{"Х0_position":u16, "Y0_position":u16})  [unwired: 1 in]
            n611 = Bundle("Длина, мм"=w1059, "Ширина, мм"=w1058) -> (w1054:cluster{"Длина, мм":u16, "Ширина, мм":u16})  [unwired: 1 in]
            n612 = property on="Мишень 6" class="Pict"("TipStrip"=w1056) -> ()  [unwired: 2 in, 2 out]
            n613 = property on="Мишень 6" class="Pict"("Position"=w1055) -> ()  [unwired: 2 in, 2 out]
            n614 = property on="Мишень 6" class="Pict"("Draw Area Size"=w1054) -> ()  [unwired: 2 in, 2 out]
          }
          frame "Выбрать" {
            n615 = Two Button Dialog(message="Вы уверены, что хотите выбрать эту мишень?", 1:"Нет" ("F button name (\"Cancel\")"), 2:"Да" ("T button name (\"OK\")")) -> (T button?=w1067:bool)
            n616 = case shown="True" w1067 {
              tunnel: [w1068 w1070] -> w1062
              tunnel: w1063 -> [w1068 w1069]
              frame False {
              }
              frame True {
                w1071 = u16 6 ("id мишени")
                n617 = property on="id мишени" class="DigNum (strict)"(error in=w1069, "Value"=w1071) -> (error out=w1072:errorcluster)  [unwired: 1 in, 1 out]
                n618 = property on="id мишени" class="DigNum (strict)"(error in=w1072, "Val(Sgnl)"=w1071) -> (error out=w1070:errorcluster)  [unwired: 1 in, 1 out]
              }
            }
          }
        }
      }
      event "Мишень 7": Shortcut Menu Selection (User) {
        n619 = event-data() -> ("ItemTag"=w1075:string)  [unwired: 1 out]
        n620 = case shown="\"Настроить\", Default" w1075 {
          tunnel: w1073 -> [w1083 w1089]
          tunnel: [w1076 w1088] -> w1074
          frame "Настроить", Default {
            n621 = call "Настройки мишени (Sub VI).vi"("Параметры мишеней вх"="М7", "error in"=w1083) -> ("Параметры мишеней вых"=w1077:T1, "error out"=w1078:errorcluster)  [unwired: 16 in]
            n622 = Unbundle(w1077) -> ("Название мишени"=w1082:string, "Х0_position"=w1087:u16, "Y0_position"=w1086:u16, "Длина, мм"=w1085:u16, "Ширина, мм"=w1084:u16)  [unwired: 5 out]
            n623 = property on="М7" class="Clust (strict)"(error in=w1078, "Val(Sgnl)"=w1077) -> (error out=w1076:errorcluster)  [unwired: 1 in, 1 out]
            n624 = Bundle("Х0_position"=w1087, "Y0_position"=w1086) -> (w1081:cluster{"Х0_position":u16, "Y0_position":u16})  [unwired: 1 in]
            n625 = Bundle("Длина, мм"=w1085, "Ширина, мм"=w1084) -> (w1080:cluster{"Длина, мм":u16, "Ширина, мм":u16})  [unwired: 1 in]
            n626 = property on="Мишень 7" class="Pict"("TipStrip"=w1082) -> ()  [unwired: 2 in, 2 out]
            n627 = property on="Мишень 7" class="Pict"("Position"=w1081) -> ()  [unwired: 2 in, 2 out]
            n628 = property on="Мишень 7" class="Pict"("Draw Area Size"=w1080) -> ()  [unwired: 2 in, 2 out]
          }
          frame "Выбрать" {
            n629 = Two Button Dialog(message="Вы уверены, что хотите выбрать эту мишень?", 1:"Нет" ("F button name (\"Cancel\")"), 2:"Да" ("T button name (\"OK\")")) -> (T button?=w1093:bool)
            n630 = case shown="True" w1093 {
              tunnel: [w1094 w1096] -> w1088
              tunnel: w1089 -> [w1094 w1095]
              frame False {
              }
              frame True {
                w1097 = u16 7 ("id мишени")
                n631 = property on="id мишени" class="DigNum (strict)"(error in=w1095, "Value"=w1097) -> (error out=w1098:errorcluster)  [unwired: 1 in, 1 out]
                n632 = property on="id мишени" class="DigNum (strict)"(error in=w1098, "Val(Sgnl)"=w1097) -> (error out=w1096:errorcluster)  [unwired: 1 in, 1 out]
              }
            }
          }
        }
      }
      event "Мишень 8": Shortcut Menu Selection (User) {
        n633 = event-data() -> ("ItemTag"=w1101:string)  [unwired: 1 out]
        n634 = case shown="\"Настроить\", Default" w1101 {
          tunnel: w1099 -> [w1109 w1115]
          tunnel: [w1102 w1114] -> w1100
          frame "Настроить", Default {
            n635 = call "Настройки мишени (Sub VI).vi"("Параметры мишеней вх"="М8", "error in"=w1109) -> ("Параметры мишеней вых"=w1103:T1, "error out"=w1104:errorcluster)  [unwired: 16 in]
            n636 = Unbundle(w1103) -> ("Название мишени"=w1108:string, "Х0_position"=w1113:u16, "Y0_position"=w1112:u16, "Длина, мм"=w1111:u16, "Ширина, мм"=w1110:u16)  [unwired: 5 out]
            n637 = property on="М8" class="Clust (strict)"(error in=w1104, "Val(Sgnl)"=w1103) -> (error out=w1102:errorcluster)  [unwired: 1 in, 1 out]
            n638 = Bundle("Х0_position"=w1113, "Y0_position"=w1112) -> (w1107:cluster{"Х0_position":u16, "Y0_position":u16})  [unwired: 1 in]
            n639 = Bundle("Длина, мм"=w1111, "Ширина, мм"=w1110) -> (w1106:cluster{"Длина, мм":u16, "Ширина, мм":u16})  [unwired: 1 in]
            n640 = property on="Мишень 8" class="Pict"("TipStrip"=w1108) -> ()  [unwired: 2 in, 2 out]
            n641 = property on="Мишень 8" class="Pict"("Position"=w1107) -> ()  [unwired: 2 in, 2 out]
            n642 = property on="Мишень 8" class="Pict"("Draw Area Size"=w1106) -> ()  [unwired: 2 in, 2 out]
          }
          frame "Выбрать" {
            n643 = Two Button Dialog(message="Вы уверены, что хотите выбрать эту мишень?", 1:"Нет" ("F button name (\"Cancel\")"), 2:"Да" ("T button name (\"OK\")")) -> (T button?=w1119:bool)
            n644 = case shown="True" w1119 {
              tunnel: [w1120 w1122] -> w1114
              tunnel: w1115 -> [w1120 w1121]
              frame False {
              }
              frame True {
                w1123 = u16 8 ("id мишени")
                n645 = property on="id мишени" class="DigNum (strict)"(error in=w1121, "Value"=w1123) -> (error out=w1124:errorcluster)  [unwired: 1 in, 1 out]
                n646 = property on="id мишени" class="DigNum (strict)"(error in=w1124, "Val(Sgnl)"=w1123) -> (error out=w1122:errorcluster)  [unwired: 1 in, 1 out]
              }
            }
          }
        }
      }
      event "Мишень 9": Shortcut Menu Selection (User) {
        n647 = event-data() -> ("ItemTag"=w1127:string)  [unwired: 1 out]
        n648 = case shown="\"Настроить\", Default" w1127 {
          tunnel: w1125 -> [w1135 w1141]
          tunnel: [w1128 w1140] -> w1126
          frame "Настроить", Default {
            n649 = call "Настройки мишени (Sub VI).vi"("Параметры мишеней вх"="М9", "error in"=w1135) -> ("Параметры мишеней вых"=w1129:T1, "error out"=w1130:errorcluster)  [unwired: 16 in]
            n650 = Unbundle(w1129) -> ("Название мишени"=w1134:string, "Х0_position"=w1139:u16, "Y0_position"=w1138:u16, "Длина, мм"=w1137:u16, "Ширина, мм"=w1136:u16)  [unwired: 5 out]
            n651 = property on="М9" class="Clust (strict)"(error in=w1130, "Val(Sgnl)"=w1129) -> (error out=w1128:errorcluster)  [unwired: 1 in, 1 out]
            n652 = Bundle("Х0_position"=w1139, "Y0_position"=w1138) -> (w1133:cluster{"Х0_position":u16, "Y0_position":u16})  [unwired: 1 in]
            n653 = Bundle("Длина, мм"=w1137, "Ширина, мм"=w1136) -> (w1132:cluster{"Длина, мм":u16, "Ширина, мм":u16})  [unwired: 1 in]
            n654 = property on="Мишень 9" class="Pict"("TipStrip"=w1134) -> ()  [unwired: 2 in, 2 out]
            n655 = property on="Мишень 9" class="Pict"("Position"=w1133) -> ()  [unwired: 2 in, 2 out]
            n656 = property on="Мишень 9" class="Pict"("Draw Area Size"=w1132) -> ()  [unwired: 2 in, 2 out]
          }
          frame "Выбрать" {
            n657 = Two Button Dialog(message="Вы уверены, что хотите выбрать эту мишень?", 1:"Нет" ("F button name (\"Cancel\")"), 2:"Да" ("T button name (\"OK\")")) -> (T button?=w1145:bool)
            n658 = case shown="True" w1145 {
              tunnel: [w1146 w1148] -> w1140
              tunnel: w1141 -> [w1146 w1147]
              frame False {
              }
              frame True {
                w1149 = u16 9 ("id мишени")
                n659 = property on="id мишени" class="DigNum (strict)"(error in=w1147, "Value"=w1149) -> (error out=w1150:errorcluster)  [unwired: 1 in, 1 out]
                n660 = property on="id мишени" class="DigNum (strict)"(error in=w1150, "Val(Sgnl)"=w1149) -> (error out=w1148:errorcluster)  [unwired: 1 in, 1 out]
              }
            }
          }
        }
      }
      event "Мишень 10": Shortcut Menu Selection (User) {
        n661 = event-data() -> ("ItemTag"=w1153:string)  [unwired: 1 out]
        n662 = case shown="\"Настроить\", Default" w1153 {
          tunnel: w1151 -> [w1161 w1167]
          tunnel: [w1154 w1166] -> w1152
          frame "Настроить", Default {
            n663 = call "Настройки мишени (Sub VI).vi"("Параметры мишеней вх"="М10", "error in"=w1161) -> ("Параметры мишеней вых"=w1155:T1, "error out"=w1156:errorcluster)  [unwired: 16 in]
            n664 = Unbundle(w1155) -> ("Название мишени"=w1160:string, "Х0_position"=w1165:u16, "Y0_position"=w1164:u16, "Длина, мм"=w1163:u16, "Ширина, мм"=w1162:u16)  [unwired: 5 out]
            n665 = property on="М10" class="Clust (strict)"(error in=w1156, "Val(Sgnl)"=w1155) -> (error out=w1154:errorcluster)  [unwired: 1 in, 1 out]
            n666 = Bundle("Х0_position"=w1165, "Y0_position"=w1164) -> (w1159:cluster{"Х0_position":u16, "Y0_position":u16})  [unwired: 1 in]
            n667 = Bundle("Длина, мм"=w1163, "Ширина, мм"=w1162) -> (w1158:cluster{"Длина, мм":u16, "Ширина, мм":u16})  [unwired: 1 in]
            n668 = property on="Мишень 10" class="Pict"("TipStrip"=w1160) -> ()  [unwired: 2 in, 2 out]
            n669 = property on="Мишень 10" class="Pict"("Position"=w1159) -> ()  [unwired: 2 in, 2 out]
            n670 = property on="Мишень 10" class="Pict"("Draw Area Size"=w1158) -> ()  [unwired: 2 in, 2 out]
          }
          frame "Выбрать" {
            n671 = Two Button Dialog(message="Вы уверены, что хотите выбрать эту мишень?", 1:"Нет" ("F button name (\"Cancel\")"), 2:"Да" ("T button name (\"OK\")")) -> (T button?=w1171:bool)
            n672 = case shown="True" w1171 {
              tunnel: [w1172 w1174] -> w1166
              tunnel: w1167 -> [w1172 w1173]
              frame False {
              }
              frame True {
                w1175 = u16 10 ("id мишени")
                n673 = property on="id мишени" class="DigNum (strict)"(error in=w1173, "Value"=w1175) -> (error out=w1176:errorcluster)  [unwired: 1 in, 1 out]
                n674 = property on="id мишени" class="DigNum (strict)"(error in=w1176, "Val(Sgnl)"=w1175) -> (error out=w1174:errorcluster)  [unwired: 1 in, 1 out]
              }
            }
          }
        }
      }
      event "id мишени", "Выстрелов до перемотки пленки", "М1", "М2", "М3", "М4", "М5", "М6", "М7", "М8", "М9", "М10": Value Change {
        # "обновление информации по мишеням"
        n675 = event-data() -> ()  [unwired: 2 out]
        n676 = local read "id мишени"() -> (w1178:u16)
        n677 = property on="Осталось:" class="Slide (strict)"(error in=w1179) -> (error out=w1180:errorcluster, "Value"=w1182:u16)  [unwired: 1 in, 1 out]
        n678 = case shown="10" w1178 {
          selector: w1178 -> [w1190 w1193 w1196 w1199 w1202 w1205 w1208 w1211 w1214 w1217]
          tunnel: [w1191 w1194 w1197 w1200 w1203 w1206 w1209 w1212 w1215 w1218] -> w1187
          tunnel: [w1190 w1193 w1196 w1199 w1202 w1205 w1208 w1211 w1214 w1217] -> w1188
          tunnel: [w1189 w1192 w1195 w1198 w1201 w1204 w1207 w1210 w1213 w1216] -> w1177
          frame 1 {
            n679 = property on="Мишень 1" class="Pict"() -> ("TipStrip"=w1189:string)  [unwired: 2 in, 2 out]
            n680 = property on="Выстрелов осталось M1" class="DigNum (strict)"() -> ("Value"=w1191:u16)  [unwired: 2 in, 2 out]
          }
          frame 2, Default {
            n681 = property on="Мишень 2" class="Pict"() -> ("TipStrip"=w1192:string)  [unwired: 2 in, 2 out]
            n682 = property on="Выстрелов осталось M2" class="DigNum (strict)"() -> ("Value"=w1194:u16)  [unwired: 2 in, 2 out]
          }
          frame 3 {
            n683 = property on="Мишень 3" class="Pict"() -> ("TipStrip"=w1195:string)  [unwired: 2 in, 2 out]
            n684 = property on="Выстрелов осталось M3" class="DigNum (strict)"() -> ("Value"=w1197:u16)  [unwired: 2 in, 2 out]
          }
          frame 4 {
            n685 = property on="Мишень 4" class="Pict"() -> ("TipStrip"=w1198:string)  [unwired: 2 in, 2 out]
            n686 = property on="Выстрелов осталось M4" class="DigNum (strict)"() -> ("Value"=w1200:u16)  [unwired: 2 in, 2 out]
          }
          frame 5 {
            n687 = property on="Мишень 5" class="Pict"() -> ("TipStrip"=w1201:string)  [unwired: 2 in, 2 out]
            n688 = property on="Выстрелов осталось M5" class="DigNum (strict)"() -> ("Value"=w1203:u16)  [unwired: 2 in, 2 out]
          }
          frame 6 {
            n689 = property on="Мишень 6" class="Pict"() -> ("TipStrip"=w1204:string)  [unwired: 2 in, 2 out]
            n690 = property on="Выстрелов осталось M6" class="DigNum (strict)"() -> ("Value"=w1206:u16)  [unwired: 2 in, 2 out]
          }
          frame 7 {
            n691 = property on="Мишень 7" class="Pict"() -> ("TipStrip"=w1207:string)  [unwired: 2 in, 2 out]
            n692 = property on="Выстрелов осталось M7" class="DigNum (strict)"() -> ("Value"=w1209:u16)  [unwired: 2 in, 2 out]
          }
          frame 8 {
            n693 = property on="Мишень 8" class="Pict"() -> ("TipStrip"=w1210:string)  [unwired: 2 in, 2 out]
            n694 = property on="Выстрелов осталось M8" class="DigNum (strict)"() -> ("Value"=w1212:u16)  [unwired: 2 in, 2 out]
          }
          frame 9 {
            n695 = property on="Мишень 9" class="Pict"() -> ("TipStrip"=w1213:string)  [unwired: 2 in, 2 out]
            n696 = property on="Выстрелов осталось M9" class="DigNum (strict)"() -> ("Value"=w1215:u16)  [unwired: 2 in, 2 out]
          }
          frame 10 {
            n697 = property on="Мишень 10" class="Pict"() -> ("TipStrip"=w1216:string)  [unwired: 2 in, 2 out]
            n698 = property on="Выстрелов осталось M10" class="DigNum (strict)"() -> ("Value"=w1218:u16)  [unwired: 2 in, 2 out]
          }
        }
        "Текущая мишень:" <- w1177
        n699 = property on="Выстрелов до перемотки пленки" class="DigNum (strict)"(error in=w1180) -> (error out=w1181:errorcluster, "Value"=w1183:u16)  [unwired: 1 in, 1 out]
        n700 = property on="TCP con ID" class="Ref (strict)"(error in=w1181) -> (error out=w1184:errorcluster, "Value"=w1185:refnum<k5>)  [unwired: 1 in, 1 out]
        n701 = call "Команда обмена 85 (обновление парам. мишени с  id ) (SubVI).vi"("id мишени"=w1188, "Выстрелов осталось"=w1187, "error in"=w1184, "TCP connection ID"=w1185, "Выстрелов до перемотки"=w1183, "До перемотки осталось"=w1182) -> ("error out"=w1186:errorcluster)  [unwired: 21 in]
      }
      event "Шаг вперед": Value Change {
        n702 = event-data() -> ("OldVal"=w1223:bool)  [unwired: 1 out]
        n703 = local write "Шаг вперед"(w1223) -> ()
        n704 = property on="TCP con ID" class="Ref (strict)"(error in=w1220) -> (error out=w1222:errorcluster, "Value"=w1221:refnum<k5>)  [unwired: 1 in, 1 out]
        n705 = call "Команда обмена 86 (принудительный шаг вперед ) (SubVI).vi"("error in"=w1222, "TCP connection ID"=w1221) -> ("error out"=w1219:errorcluster)  [unwired: 25 in]
      }
      event "Фокус +": Value Change {
        n706 = event-data() -> ("OldVal"=w1224:bool)  [unwired: 1 out]
        n707 = local write "Фокус +"(w1224) -> ()
        n708 = property on="TCP con ID" class="Ref (strict)"(error in=w1228) -> (error out=w1226:errorcluster, "Value"=w1227:refnum<k5>)  [unwired: 1 in, 1 out]
        n709 = call "Команда обмена 87 (фокус +) (SubVI).vi"("error in"=w1226, "TCP connection ID"=w1227) -> ("error out"=w1225:errorcluster)  [unwired: 25 in]
      }
      event "Фокус --": Value Change {
        n710 = event-data() -> ("OldVal"=w1232:bool)  [unwired: 1 out]
        n711 = local write "Фокус --"(w1232) -> ()
        n712 = property on="TCP con ID" class="Ref (strict)"(error in=w1233) -> (error out=w1230:errorcluster, "Value"=w1231:refnum<k5>)  [unwired: 1 in, 1 out]
        n713 = call "Команда обмена 88 (фокус -) (SubVI).vi"("error in"=w1230, "TCP connection ID"=w1231) -> ("error out"=w1229:errorcluster)  [unwired: 25 in]
      }
      event "Перемотка пленки": Value Change {
        n714 = event-data() -> ("OldVal"=w1237:bool)  [unwired: 1 out]
        n715 = local write "Перемотка пленки"(w1237) -> ()
        n716 = property on="TCP con ID" class="Ref (strict)"(error in=w1238) -> (error out=w1235:errorcluster, "Value"=w1236:refnum<k5>)  [unwired: 1 in, 1 out]
        n717 = call "Команда обмена 89 (перемотка пленки) (SubVI).vi"("error in"=w1235, "TCP connection ID"=w1236) -> ("error out"=w1234:errorcluster)  [unwired: 25 in]
      }
      event "UpButton": Value Change {
        # "Ручной сдвиг мишени вверх"
        n718 = event-data() -> ("OldVal"=w1249:bool)  [unwired: 1 out]
        n719 = local write "UpButton"(w1249) -> ()
        n720 = property on="id мишени" class="DigNum (strict)"() -> ("Value"=w1245:u16)  [unwired: 2 in, 2 out]
        n721 = case shown="1, Default" w1245 {
          tunnel: [w1253 w1256 w1259 w1262 w1265 w1268 w1271 w1274 w1277 w1280] -> w1240
          tunnel: w1244 -> [w1253 w1256 w1259 w1262 w1265 w1268 w1271 w1274 w1277 w1280]
          tunnel: [w1252 w1255 w1258 w1261 w1264 w1267 w1270 w1273 w1276 w1279] -> w1243
          tunnel: w1242 -> [w1252 w1255 w1258 w1261 w1264 w1267 w1270 w1273 w1276 w1279]
          tunnel: [w1251 w1254 w1257 w1260 w1263 w1266 w1269 w1272 w1275 w1278] -> w1241
          frame 4 {
            n722 = control-ref of="Мишень 4"() -> (w1251:refnum<vi>)
          }
          frame 3 {
            n723 = control-ref of="Мишень 3"() -> (w1254:refnum<vi>)
          }
          frame 2 {
            n724 = control-ref of="Мишень 2"() -> (w1257:refnum<vi>)
          }
          frame 1, Default {
            n725 = control-ref of="Мишень 1"() -> (w1260:refnum<vi>)
          }
          frame 6 {
            n726 = control-ref of="Мишень 6"() -> (w1263:refnum<vi>)
          }
          frame 7 {
            n727 = control-ref of="Мишень 7"() -> (w1266:refnum<vi>)
          }
          frame 8 {
            n728 = control-ref of="Мишень 8"() -> (w1269:refnum<vi>)
          }
          frame 9 {
            n729 = control-ref of="Мишень 9"() -> (w1272:refnum<vi>)
          }
          frame 10 {
            n730 = control-ref of="Мишень 10"() -> (w1275:refnum<vi>)
          }
          frame 5 {
            n731 = control-ref of="Мишень 5"() -> (w1278:refnum<vi>)
          }
        }
        n732 = control-ref of="XY лазера"() -> (w1246:refnum<vi>)
        n733 = call "Анализ выхода за границы мишени (SubVI).vi"("Ref мишени"=w1241, "Ref XY лазера"=w1246, "error in"=w1243, "Шаг перехода"=w1240) -> ("Шаг перехода вых"=w1239:string, "вышел за рамки сверху"=w1247:bool, "error out"=w1248:errorcluster)  [unwired: 10 in, 3 out]
        n734 = case shown="False" w1247 {
          tunnel: [w1285 w1286] -> w1250
          tunnel: w1248 -> [w1282 w1286]
          tunnel: w1239 -> [w1281 _]
          frame False {
            n735 = property on="TCP con ID" class="Ref (strict)"(error in=w1282) -> (error out=w1284:errorcluster, "Value"=w1283:refnum<k5>)  [unwired: 1 in, 1 out]
            n736 = call "Команда обмена 70 (ручное упр. ВВЕРХ) (SubVI).vi"("Шаг перехода"=w1281, "error in"=w1284, "TCP connection ID"=w1283) -> ("error out"=w1285:errorcluster)  [unwired: 24 in]
          }
          frame True {
          }
        }
      }
      event "DownButton": Value Change {
        # "Ручной сдвиг мишени вниз"
        n737 = event-data() -> ("OldVal"=w1298:bool)  [unwired: 1 out]
        n738 = local write "DownButton"(w1298) -> ()
        n739 = property on="id мишени" class="DigNum (strict)"() -> ("Value"=w1295:u16)  [unwired: 2 in, 2 out]
        n740 = case shown="1, Default" w1295 {
          tunnel: [w1301 w1304 w1307 w1310 w1313 w1316 w1319 w1322 w1325 w1328] -> w1288
          tunnel: w1294 -> [w1301 w1304 w1307 w1310 w1313 w1316 w1319 w1322 w1325 w1328]
          tunnel: [w1300 w1303 w1306 w1309 w1312 w1315 w1318 w1321 w1324 w1327] -> w1293
          tunnel: w1292 -> [w1300 w1303 w1306 w1309 w1312 w1315 w1318 w1321 w1324 w1327]
          tunnel: [w1299 w1302 w1305 w1308 w1311 w1314 w1317 w1320 w1323 w1326] -> w1291
          frame 4 {
            n741 = control-ref of="Мишень 4"() -> (w1299:refnum<vi>)
          }
          frame 3 {
            n742 = control-ref of="Мишень 3"() -> (w1302:refnum<vi>)
          }
          frame 2 {
            n743 = control-ref of="Мишень 2"() -> (w1305:refnum<vi>)
          }
          frame 1, Default {
            n744 = control-ref of="Мишень 1"() -> (w1308:refnum<vi>)
          }
          frame 6 {
            n745 = control-ref of="Мишень 6"() -> (w1311:refnum<vi>)
          }
          frame 7 {
            n746 = control-ref of="Мишень 7"() -> (w1314:refnum<vi>)
          }
          frame 8 {
            n747 = control-ref of="Мишень 8"() -> (w1317:refnum<vi>)
          }
          frame 9 {
            n748 = control-ref of="Мишень 9"() -> (w1320:refnum<vi>)
          }
          frame 10 {
            n749 = control-ref of="Мишень 10"() -> (w1323:refnum<vi>)
          }
          frame 5 {
            n750 = control-ref of="Мишень 5"() -> (w1326:refnum<vi>)
          }
        }
        n751 = control-ref of="XY лазера"() -> (w1296:refnum<vi>)
        n752 = call "Анализ выхода за границы мишени (SubVI).vi"("Ref мишени"=w1291, "Ref XY лазера"=w1296, "error in"=w1293, "Шаг перехода"=w1288) -> ("Шаг перехода вых"=w1287:string, "вышел за рамки снизу"=w1290:bool, "error out"=w1297:errorcluster)  [unwired: 10 in, 3 out]
        n753 = case shown="False" w1290 {
          tunnel: [w1333 w1334] -> w1289
          tunnel: w1297 -> [w1330 w1334]
          tunnel: w1287 -> [w1329 _]
          frame False {
            n754 = property on="TCP con ID" class="Ref (strict)"(error in=w1330) -> (error out=w1332:errorcluster, "Value"=w1331:refnum<k5>)  [unwired: 1 in, 1 out]
            n755 = call "Команда обмена 71 (ручное упр. ВНИЗ) (SubVI).vi"("Шаг перехода"=w1329, "error in"=w1332, "TCP connection ID"=w1331) -> ("error out"=w1333:errorcluster)  [unwired: 24 in]
          }
          frame True {
          }
        }
      }
      event "LeftButton": Value Change {
        # "Ручной сдвиг мишени влево"
        n756 = event-data() -> ("OldVal"=w1337:bool)  [unwired: 1 out]
        n757 = local write "LeftButton"(w1337) -> ()
        n758 = property on="id мишени" class="DigNum (strict)"() -> ("Value"=w1343:u16)  [unwired: 2 in, 2 out]
        n759 = case shown="1, Default" w1343 {
          tunnel: [w1349 w1352 w1355 w1358 w1361 w1364 w1367 w1370 w1373 w1376] -> w1336
          tunnel: w1342 -> [w1349 w1352 w1355 w1358 w1361 w1364 w1367 w1370 w1373 w1376]
          tunnel: [w1348 w1351 w1354 w1357 w1360 w1363 w1366 w1369 w1372 w1375] -> w1341
          tunnel: w1340 -> [w1348 w1351 w1354 w1357 w1360 w1363 w1366 w1369 w1372 w1375]
          tunnel: [w1347 w1350 w1353 w1356 w1359 w1362 w1365 w1368 w1371 w1374] -> w1339
          frame 4 {
            n760 = control-ref of="Мишень 4"() -> (w1347:refnum<vi>)
          }
          frame 3 {
            n761 = control-ref of="Мишень 3"() -> (w1350:refnum<vi>)
          }
          frame 2 {
            n762 = control-ref of="Мишень 2"() -> (w1353:refnum<vi>)
          }
          frame 1, Default {
            n763 = control-ref of="Мишень 1"() -> (w1356:refnum<vi>)
          }
          frame 6 {
            n764 = control-ref of="Мишень 6"() -> (w1359:refnum<vi>)
          }
          frame 7 {
            n765 = control-ref of="Мишень 7"() -> (w1362:refnum<vi>)
          }
          frame 8 {
            n766 = control-ref of="Мишень 8"() -> (w1365:refnum<vi>)
          }
          frame 9 {
            n767 = control-ref of="Мишень 9"() -> (w1368:refnum<vi>)
          }
          frame 10 {
            n768 = control-ref of="Мишень 10"() -> (w1371:refnum<vi>)
          }
          frame 5 {
            n769 = control-ref of="Мишень 5"() -> (w1374:refnum<vi>)
          }
        }
        n770 = control-ref of="XY лазера"() -> (w1344:refnum<vi>)
        n771 = call "Анализ выхода за границы мишени (SubVI).vi"("Ref мишени"=w1339, "Ref XY лазера"=w1344, "error in"=w1341, "Шаг перехода"=w1336) -> ("Шаг перехода вых"=w1335:string, "вышел за рамки слева"=w1338:bool, "error out"=w1345:errorcluster)  [unwired: 10 in, 3 out]
        n772 = case shown="False" w1338 {
          tunnel: [w1381 w1382] -> w1346
          tunnel: w1345 -> [w1378 w1382]
          tunnel: w1335 -> [w1377 _]
          frame False {
            n773 = property on="TCP con ID" class="Ref (strict)"(error in=w1378) -> (error out=w1380:errorcluster, "Value"=w1379:refnum<k5>)  [unwired: 1 in, 1 out]
            n774 = call "Команда обмена 72 (ручное упр. ВЛЕВО) (SubVI).vi"("Шаг перехода"=w1377, "error in"=w1380, "TCP connection ID"=w1379) -> ("error out"=w1381:errorcluster)  [unwired: 24 in]
          }
          frame True {
          }
        }
      }
      event "RightButton": Value Change {
        # "Ручной сдвиг мишени влево"
        n775 = event-data() -> ("OldVal"=w1386:bool)  [unwired: 1 out]
        n776 = local write "RightButton"(w1386) -> ()
        n777 = property on="id мишени" class="DigNum (strict)"() -> ("Value"=w1391:u16)  [unwired: 2 in, 2 out]
        n778 = case shown="1, Default" w1391 {
          tunnel: [w1397 w1400 w1403 w1406 w1409 w1412 w1415 w1418 w1421 w1424] -> w1384
          tunnel: w1390 -> [w1397 w1400 w1403 w1406 w1409 w1412 w1415 w1418 w1421 w1424]
          tunnel: [w1396 w1399 w1402 w1405 w1408 w1411 w1414 w1417 w1420 w1423] -> w1389
          tunnel: w1388 -> [w1396 w1399 w1402 w1405 w1408 w1411 w1414 w1417 w1420 w1423]
          tunnel: [w1395 w1398 w1401 w1404 w1407 w1410 w1413 w1416 w1419 w1422] -> w1387
          frame 4 {
            n779 = control-ref of="Мишень 4"() -> (w1395:refnum<vi>)
          }
          frame 3 {
            n780 = control-ref of="Мишень 3"() -> (w1398:refnum<vi>)
          }
          frame 2 {
            n781 = control-ref of="Мишень 2"() -> (w1401:refnum<vi>)
          }
          frame 1, Default {
            n782 = control-ref of="Мишень 1"() -> (w1404:refnum<vi>)
          }
          frame 6 {
            n783 = control-ref of="Мишень 6"() -> (w1407:refnum<vi>)
          }
          frame 7 {
            n784 = control-ref of="Мишень 7"() -> (w1410:refnum<vi>)
          }
          frame 8 {
            n785 = control-ref of="Мишень 8"() -> (w1413:refnum<vi>)
          }
          frame 9 {
            n786 = control-ref of="Мишень 9"() -> (w1416:refnum<vi>)
          }
          frame 10 {
            n787 = control-ref of="Мишень 10"() -> (w1419:refnum<vi>)
          }
          frame 5 {
            n788 = control-ref of="Мишень 5"() -> (w1422:refnum<vi>)
          }
        }
        n789 = control-ref of="XY лазера"() -> (w1392:refnum<vi>)
        n790 = call "Анализ выхода за границы мишени (SubVI).vi"("Ref мишени"=w1387, "Ref XY лазера"=w1392, "error in"=w1389, "Шаг перехода"=w1384) -> ("Шаг перехода вых"=w1383:string, "вышел за рамки справа"=w1385:bool, "error out"=w1393:errorcluster)  [unwired: 10 in, 3 out]
        n791 = case shown="False" w1385 {
          tunnel: [w1429 w1430] -> w1394
          tunnel: w1393 -> [w1426 w1430]
          tunnel: w1383 -> [w1425 _]
          frame False {
            n792 = property on="TCP con ID" class="Ref (strict)"(error in=w1426) -> (error out=w1428:errorcluster, "Value"=w1427:refnum<k5>)  [unwired: 1 in, 1 out]
            n793 = call "Команда обмена 73 (ручное упр. ВПРАВО) (SubVI).vi"("Шаг перехода"=w1425, "error in"=w1428, "TCP connection ID"=w1427) -> ("error out"=w1429:errorcluster)  [unwired: 24 in]
          }
          frame True {
          }
        }
      }
      event "Конфигурация сохранена": Value Change {
        # "Сохранение конфигурации"
        n794 = event-data() -> ("OldVal"=w1434:bool)  [unwired: 1 out]
        n795 = flat-sequence {
          tunnel: w1434 -> [w1526]
          tunnel: w1433 -> [w1525]
          tunnel: [w1438] -> w1431
          tunnel: [w1545] -> w1432
          tunnel: w1431 -> [w1545]
          frame #0 {
            n796 = property on="Конфигурация сохранена" class="Bool (strict)"(error in=w1525, "Value"=w1526) -> (error out=w1495:errorcluster)  [unwired: 1 in, 1 out]
            n797 = local read "М10"() -> (w1515:T1)
            n798 = local read "выстрел X М1"() -> (w1474:u16)
            n799 = local read "выстрел Y М1"() -> (w1473:u16)
            n800 = local read "выстрел X М2"() -> (w1472:u16)
            n801 = local read "выстрел X М3"() -> (w1470:u16)
            n802 = local read "М1"() -> (w1524:T1)
            n803 = local read "М2"() -> (w1523:T1)
            n804 = local read "М3"() -> (w1522:T1)
            n805 = local read "М4"() -> (w1521:T1)
            n806 = local read "М5"() -> (w1520:T1)
            n807 = local read "М6"() -> (w1519:T1)
            n808 = local read "М7"() -> (w1518:T1)
            n809 = local read "М8"() -> (w1517:T1)
            n810 = local read "М9"() -> (w1516:T1)
            n811 = local read "выстрел Y М2"() -> (w1471:u16)
            n812 = local read "выстрел Y М3"() -> (w1469:u16)
            n813 = local read "выстрел X М4"() -> (w1468:u16)
            n814 = local read "выстрел X М5"() -> (w1466:u16)
            n815 = local read "выстрел Y М4"() -> (w1467:u16)
            n816 = local read "выстрел Y М5"() -> (w1465:u16)
            n817 = property on="Мишень 1" class="Pict"(error in=w1495) -> (error out=w1496:errorcluster, "Visible"=w1493:bool)  [unwired: 1 in, 1 out]
            n818 = property on="Мишень 2" class="Pict"(error in=w1496) -> (error out=w1497:errorcluster, "Visible"=w1492:bool)  [unwired: 1 in, 1 out]
            n819 = Bundle("М1"=w1524, "М2"=w1523, "М3"=w1522, "М4"=w1521, "М5"=w1520, "М6"=w1519, "М7"=w1518, "М8"=w1517, "М9"=w1516, "М10"=w1515) -> (w1451:T8)  [unwired: 1 in]
            n820 = Bundle("выстрел X М1"=w1474, "выстрел Y М1"=w1473, "выстрел X М2"=w1472, "выстрел Y М2"=w1471, "выстрел X М3"=w1470, "выстрел Y М3"=w1469, "выстрел X М4"=w1468, "выстрел Y М4"=w1467, "выстрел X М5"=w1466, "выстрел Y М5"=w1465) -> (w1443:T9)  [unwired: 1 in]
            n821 = property on="Мишень 3" class="Pict"(error in=w1497) -> (error out=w1498:errorcluster, "Visible"=w1491:bool)  [unwired: 1 in, 1 out]
            n822 = property on="Мишень 4" class="Pict"(error in=w1498) -> (error out=w1499:errorcluster, "Visible"=w1490:bool)  [unwired: 1 in, 1 out]
            n823 = local read "выстрел X М10"() -> (w1456:u16)
            n824 = local read "выстрел X М6"() -> (w1464:u16)
            n825 = local read "выстрел Y М10"() -> (w1455:u16)
            n826 = local read "Знак перех. dX М1"() -> (w1514:i8)
            n827 = local read "Знак перех. dX М2"() -> (w1513:i8)
            n828 = local read "Знак перех. dX М3"() -> (w1512:i8)
            n829 = local read "Знак перех. dX М4"() -> (w1511:i8)
            n830 = local read "Знак перех. dX М5"() -> (w1510:i8)
            n831 = local read "Знак перех. dX М6"() -> (w1509:i8)
            n832 = local read "Знак перех. dX М7"() -> (w1508:i8)
            n833 = local read "Знак перех. dX М8"() -> (w1507:i8)
            n834 = local read "Знак перех. dX М9"() -> (w1506:i8)
            n835 = local read "Знак перех. dX М10"() -> (w1505:i8)
            n836 = local read "выстрел Y М6"() -> (w1463:u16)
            n837 = local read "выстрел X М7"() -> (w1462:u16)
            n838 = local read "выстрел X М8"() -> (w1460:u16)
            n839 = local read "выстрел Y М7"() -> (w1461:u16)
            n840 = local read "выстрел Y М8"() -> (w1459:u16)
            n841 = local read "выстрел X М9"() -> (w1458:u16)
            n842 = local read "выстрел Y М9"() -> (w1457:u16)
            n843 = property on="Мишень 5" class="Pict"(error in=w1499) -> (error out=w1504:errorcluster, "Visible"=w1489:bool)  [unwired: 1 in, 1 out]
            n844 = property on="Мишень 6" class="Pict"(error in=w1504) -> (error out=w1503:errorcluster, "Visible"=w1488:bool)  [unwired: 1 in, 1 out]
            n845 = Bundle("выстрел X М6"=w1464, "выстрел Y М6"=w1463, "выстрел X М7"=w1462, "выстрел Y М7"=w1461, "выстрел X М8"=w1460, "выстрел Y М8"=w1459, "выстрел X М9"=w1458, "выстрел Y М9"=w1457, "выстрел X М10"=w1456, "выстрел Y М10"=w1455) -> (w1444:T10)  [unwired: 1 in]
            n846 = property on="Мишень 7" class="Pict"(error in=w1503) -> (error out=w1502:errorcluster, "Visible"=w1487:bool)  [unwired: 1 in, 1 out]
            n847 = Bundle("Знак перех. dX М1"=w1514, "Знак перех. dX М2"=w1513, "Знак перех. dX М3"=w1512, "Знак перех. dX М4"=w1511, "Знак перех. dX М5"=w1510, "Знак перех. dX М6"=w1509, "Знак перех. dX М7"=w1508, "Знак перех. dX М8"=w1507, "Знак перех. dX М9"=w1506, "Знак перех. dX М10"=w1505) -> (w1452:T11)  [unwired: 1 in]
            n848 = disable-structure shown="Disabled" {
              disable-tunnel: [w1528 _] -> w1442
              frame Disabled {
                n849 = local read "Мишень 1"() -> (w1538:picture)
                n850 = local read "Мишень 2"() -> (w1537:picture)
                n851 = local read "Мишень 3"() -> (w1536:picture)
                n852 = local read "Мишень 4"() -> (w1535:picture)
                n853 = local read "Мишень 5"() -> (w1534:picture)
                n854 = local read "Мишень 6"() -> (w1533:picture)
                n855 = local read "Мишень 7"() -> (w1532:picture)
                n856 = local read "Мишень 8"() -> (w1531:picture)
                n857 = local read "Мишень 9"() -> (w1530:picture)
                n858 = local read "Мишень 10"() -> (w1529:picture)
                n859 = Bundle("Мишень 1"=w1538, "Мишень 2"=w1537, "Мишень 3"=w1536, "Мишень 4"=w1535, "Мишень 5"=w1534, "Мишень 6"=w1533, "Мишень 7"=w1532, "Мишень 8"=w1531, "Мишень 9"=w1530, "Мишень 10"=w1529) -> (w1528:T12)  [unwired: 1 in]
              }
              frame Enabled {
              }
            }
            n860 = property on="Мишень 8" class="Pict"(error in=w1502) -> (error out=w1501:errorcluster, "Visible"=w1486:bool)  [unwired: 1 in, 1 out]
            n861 = property on="Мишень 9" class="Pict"(error in=w1501) -> (error out=w1500:errorcluster, "Visible"=w1485:bool)  [unwired: 1 in, 1 out]
            n862 = local read "Выстрелов осталось M1"() -> (w1484:u16)
            n863 = local read "Выстрелов осталось M2"() -> (w1483:u16)
            n864 = local read "Выстрелов осталось M3"() -> (w1482:u16)
            n865 = local read "Выстрелов осталось M4"() -> (w1481:u16)
            n866 = local read "Выстрелов осталось M5"() -> (w1480:u16)
            n867 = local read "Выстрелов осталось M6"() -> (w1479:u16)
            n868 = local read "Выстрелов осталось M7"() -> (w1478:u16)
            n869 = local read "Выстрелов осталось M8"() -> (w1477:u16)
            n870 = local read "Выстрелов осталось M9"() -> (w1476:u16)
            n871 = local read "Выстрелов осталось M10"() -> (w1475:u16)
            n872 = property on="Мишень 10" class="Pict"(error in=w1500) -> (error out=w1449:errorcluster, "Visible"=w1494:bool)  [unwired: 1 in, 1 out]
            n873 = Bundle("Visible"=w1493, "Visible"=w1492, "Visible"=w1491, "Visible"=w1490, "Visible"=w1489, "Visible"=w1488, "Visible"=w1487, "Visible"=w1486, "Visible"=w1485, "Visible"=w1494) -> (w1450:T13)  [unwired: 1 in]
            n874 = property on="текущ. инфо" class="Bool (strict)"(error in=w1449) -> (error out=w1448:errorcluster, "Position"=w1447:T3)  [unwired: 1 in, 1 out]
            n875 = Bundle("Выстрелов осталось M1"=w1484, "Выстрелов осталось M2"=w1483, "Выстрелов осталось M3"=w1482, "Выстрелов осталось M4"=w1481, "Выстрелов осталось M5"=w1480, "Выстрелов осталось M6"=w1479, "Выстрелов осталось M7"=w1478, "Выстрелов осталось M8"=w1477, "Выстрелов осталось M9"=w1476, "Выстрелов осталось M10"=w1475) -> (w1454:T14)  [unwired: 1 in]
            n876 = property on="XY лазера" class="Bool (strict)"(error in=w1448) -> (error out=w1445:errorcluster, "Position"=w1446:T3)  [unwired: 1 in, 1 out]
            n877 = local read "id мишени"() -> (w1453:u16)
            n878 = local read "Флаг резерв. сохр."() -> (w1435:bool)
            n879 = call "Фиксироание всех параметров (SubVI).vi"("Параметры всех мишеней"=w1451, "Видимость мишеней"=w1450, "error in"=w1445, "полож. красной точки лазера"=w1446, "полож. текущ. инф."=w1447, "Знаки Dx всех мишеней"=w1452, "Текущ. положение лазера на мишенях 1 - 5"=w1443, "текущий id мишени"=w1453, "Выстрелов осталось по всем мишеням"=w1454, "Текущ. положение лазера на мишенях 6 - 10"=w1444) -> ("Строка параметров мишеней для сохранения"=w1439:string, "error out"=w1441:errorcluster)  [unwired: 16 in]
            n880 = call "Запись в файл (SubVI).vi"("Резервное сохр."=w1435, "error in"=w1441, "Строка параметров мишеней для сохранения"=w1439) -> ("error out"=w1440:errorcluster, "Путь к файлу"=w1436:path)  [unwired: 6 in, 1 out]
            n881 = Not A Number/Path/Refnum?(number/path/refnum=w1436) -> (NaN/Path/Refnum?=w1437:bool)
            n882 = case shown="False" w1437 {
              tunnel: w1436 -> [w1527 _]
              frame False {
                "Текущая конфигурация:" <- w1527
              }
              frame True {
              }
            }
            n883 = disable-structure shown="Enabled" {
              disable-tunnel: w1442 -> [w1541 _]
              disable-tunnel: w1440 -> [w1540 w1542]
              disable-tunnel: [w1539 w1542] -> w1438
              frame Disabled {
                n884 = call "Сохр. рисунков мишеней в файл (SubVI).vi"("error in"=w1540, "Кластер рисунков всех мишеней"=w1541) -> ("error out"=w1539:errorcluster)  [unwired: 13 in]
              }
              frame Enabled {
              }
            }
          }
          frame #1 {
            n885 = local read "флаг закрытия с сохр."() -> (w1544:bool)
            n886 = property on="Флаг резерв. сохр." class="Bool (strict)"("Value"=FALSE ("Флаг резерв. сохр.")) -> ()  [unwired: 2 in, 2 out]
            n887 = Quit LabVIEW(quit? (T)=w1544) -> ()
          }
        }
      }
      event "Сбросить конфигурацию": Value Change {
        # "Сброс текущей конфигурации"
        n888 = event-data() -> ("OldVal"=w1550:bool)  [unwired: 1 out]
        n889 = local write "Сбросить конфигурацию"(w1550) -> ()
        n890 = Two Button Dialog(message="Вы уверены, что хотите СБРОСИТЬ текущую конфигурацию?", 1:"Нет" ("F button name (\"Cancel\")"), 2:"Да" ("T button name (\"OK\")")) -> (T button?=w1546:bool)
        n891 = case shown="True" w1546 {
          frame False {
          }
          frame True {
            w1556 = T3 {"Left"=1200, "Top"=1000} ("Position")
            w1579 = i8 1 ("Выстрелов осталось M1")
            w1603 = T1 {"Название мишени"="?", "Х0_position"=400, "Y0_position"=200, "Длина, мм"=200, "Ширина, мм"=200, "Шаг перехода по горизонтали"=2.0, "Шаг перехода по вертикали"=2.0, "Выстрелов до перехода"=1, "Xo to send "=0, "Yo to send"=0} ("Параметры М1")
            w1610 = "" ("Tip Strip")
            n892 = property on="Мишень 1" class="Pict"("Visible"=FALSE) -> (error out=w1559:errorcluster)  [unwired: 2 in, 1 out]
            n893 = local write "Знак перех. dX М1"(i8 1 ("Знак перех. dX М1")) -> ()
            n894 = local write "Знак перех. dX М2"(w1579) -> ()
            n895 = local write "Знак перех. dX М3"(w1579) -> ()
            n896 = local write "Знак перех. dX М4"(w1579) -> ()
            n897 = local write "Знак перех. dX М5"(w1579) -> ()
            n898 = local write "Знак перех. dX М6"(w1579) -> ()
            n899 = local write "Знак перех. dX М7"(w1579) -> ()
            n900 = local write "Знак перех. dX М8"(w1579) -> ()
            n901 = local write "Знак перех. dX М10"(i8 1 ("Выстрелов осталось M1")) -> ()
            n902 = local write "Знак перех. dX М9"(w1579) -> ()
            n903 = local write "выстрел X М1"(u16 0 ("Выстрелов осталось M1")) -> ()
            n904 = local write "выстрел Y М1"(u16 0 ("Выстрелов осталось M2")) -> ()
            n905 = local write "выстрел X М2"(u16 0 ("Выстрелов осталось M3")) -> ()
            n906 = local write "выстрел Y М2"(u16 0 ("Выстрелов осталось M4")) -> ()
            n907 = local write "выстрел X М3"(u16 0 ("Выстрелов осталось M5")) -> ()
            n908 = local write "выстрел Y М3"(u16 0 ("Выстрелов осталось M6")) -> ()
            n909 = local write "выстрел X М4"(u16 0 ("выстрел X М9")) -> ()
            n910 = local write "выстрел Y М4"(u16 0 ("выстрел Y М9")) -> ()
            n911 = local write "выстрел X М5"(u16 0 ("выстрел X М10")) -> ()
            n912 = local write "выстрел Y М5"(u16 0 ("выстрел Y М10")) -> ()
            n913 = property on="Мишень 2" class="Pict"(error in=w1559, "Visible"=FALSE) -> (error out=w1562:errorcluster)  [unwired: 1 in, 1 out]
            n914 = local write "Осталось:"(u16 0 ("До перемотки осталось")) -> ()
            n915 = property on="Мишень 3" class="Pict"(error in=w1562, "Visible"=FALSE) -> (error out=w1564:errorcluster)  [unwired: 1 in, 1 out]
            n916 = String To Path(string="Новая конфигурация...") -> (path=w1554:path)
            n917 = local write "Текущая конфигурация:"(w1554) -> ()
            n918 = property on="Мишень 4" class="Pict"(error in=w1564, "Visible"=FALSE) -> (error out=w1566:errorcluster)  [unwired: 1 in, 1 out]
            n919 = call "Empty Picture"() -> ("empty picture"=w1578:picture)
            n920 = property on="Мишень 5" class="Pict"(error in=w1566, "Visible"=FALSE) -> (error out=w1577:errorcluster)  [unwired: 1 in, 1 out]
            n921 = local write "выстрел X М6"(u16 0 ("Выстрелов осталось M1")) -> ()
            n922 = local write "выстрел Y М6"(u16 0 ("Выстрелов осталось M2")) -> ()
            n923 = local write "выстрел X М7"(u16 0 ("Выстрелов осталось M3")) -> ()
            n924 = local write "выстрел Y М7"(u16 0 ("Выстрелов осталось M4")) -> ()
            n925 = local write "выстрел X М8"(u16 0 ("Выстрелов осталось M5")) -> ()
            n926 = local write "выстрел Y М8"(u16 0 ("Выстрелов осталось M6")) -> ()
            n927 = local write "выстрел X М9"(u16 0 ("выстрел X М9")) -> ()
            n928 = local write "выстрел Y М9"(u16 0 ("выстрел Y М9")) -> ()
            n929 = local write "выстрел X М10"(u16 0 ("выстрел X М10")) -> ()
            n930 = local write "выстрел Y М10"(u16 0 ("выстрел Y М10")) -> ()
            n931 = local write "Мишень 1"(w1578) -> ()
            n932 = local write "Мишень 2"(w1578) -> ()
            n933 = local write "Мишень 3"(w1578) -> ()
            n934 = local write "Мишень 4"(w1578) -> ()
            n935 = local write "Мишень 5"(w1578) -> ()
            n936 = local write "Мишень 6"(w1578) -> ()
            n937 = local write "Мишень 7"(w1578) -> ()
            n938 = local write "Мишень 8"(w1578) -> ()
            n939 = local write "Мишень 9"(w1578) -> ()
            n940 = local write "Мишень 10"(w1578) -> ()
            n941 = property on="Шаг вперед" class="Bool (strict)"("DisabledEnum"=T2."Disabled and Grayed Out" ("Disabled")) -> ()  [unwired: 2 in, 2 out]
            n942 = property on="Мишень 6" class="Pict"(error in=w1577, "Visible"=FALSE) -> (error out=w1576:errorcluster)  [unwired: 1 in, 1 out]
            n943 = property on="Счетчик выстрелов:" class="DigNum (strict)"("Value"=u32 0 ("Счетчик выстрелов:")) -> ()  [unwired: 2 in, 2 out]
            n944 = property on="Мишень 7" class="Pict"(error in=w1576, "Visible"=FALSE) -> (error out=w1573:errorcluster)  [unwired: 1 in, 1 out]
            n945 = local write "id мишени"(u16 0 ("id мишени")) -> ()
            n946 = local write "М1"(w1603) -> ()
            n947 = local write "М2"(w1603) -> ()
            n948 = local write "М3"(w1603) -> ()
            n949 = local write "М4"(w1603) -> ()
            n950 = local write "М5"(w1603) -> ()
            n951 = local write "М6"(w1603) -> ()
            n952 = local write "М7"(w1603) -> ()
            n953 = local write "М8"(w1603) -> ()
            n954 = local write "М9"(w1603) -> ()
            n955 = local write "М10"(w1603) -> ()
            n956 = property on="Мишень 8" class="Pict"(error in=w1573, "Visible"=FALSE) -> (error out=w1571:errorcluster)  [unwired: 1 in, 1 out]
            n957 = property on="Выстрел по мишени!" class="DigNum (strict)"("Value"=u32 0 ("Выстрел по мишени!")) -> ()  [unwired: 2 in, 2 out]
            n958 = property on="Мишень 10" class="Pict"("TipStrip"=w1610) -> ()  [unwired: 2 in, 2 out]
            n959 = property on="Мишень 9" class="Pict"("TipStrip"=w1610) -> ()  [unwired: 2 in, 2 out]
            n960 = property on="Мишень 8" class="Pict"("TipStrip"=w1610) -> ()  [unwired: 2 in, 2 out]
            n961 = property on="Мишень 7" class="Pict"("TipStrip"=w1610) -> ()  [unwired: 2 in, 2 out]
            n962 = property on="Мишень 6" class="Pict"("TipStrip"=w1610) -> ()  [unwired: 2 in, 2 out]
            n963 = property on="Мишень 5" class="Pict"("TipStrip"=w1610) -> ()  [unwired: 2 in, 2 out]
            n964 = property on="Мишень 4" class="Pict"("TipStrip"=w1610) -> ()  [unwired: 2 in, 2 out]
            n965 = property on="Мишень 3" class="Pict"("TipStrip"=w1610) -> ()  [unwired: 2 in, 2 out]
            n966 = property on="Мишень 2" class="Pict"("TipStrip"=w1610) -> ()  [unwired: 2 in, 2 out]
            n967 = property on="Мишень 1" class="Pict"("TipStrip"=w1610) -> ()  [unwired: 2 in, 2 out]
            n968 = property on="Мишень 9" class="Pict"(error in=w1571, "Visible"=FALSE) -> (error out=w1569:errorcluster)  [unwired: 1 in, 1 out]
            n969 = property on="Мишень 10" class="Pict"(error in=w1569, "Visible"=FALSE) -> ()  [unwired: 1 in, 2 out]
            n970 = property on="Счетчик мишеней" class="DigNum (strict)"("Value"=u32 0 ("Выстрел по мишени!")) -> ()  [unwired: 2 in, 2 out]
            n971 = Bundle("Счетчик мишеней"=u32 200, "Счетчик мишеней"=u32 200) -> (w1609:T15)  [unwired: 1 in]
            n972 = Bundle("Счетчик мишеней"=400, "Счетчик мишеней"=200) -> (w1608:T16)  [unwired: 1 in]
            n973 = property on="Мишень 1" class="Pict"("Draw Area Size"=w1609) -> ()  [unwired: 2 in, 2 out]
            n974 = property on="Мишень 2" class="Pict"("Draw Area Size"=w1609) -> ()  [unwired: 2 in, 2 out]
            n975 = property on="Мишень 1" class="Pict"("Position"=w1608) -> ()  [unwired: 2 in, 2 out]
            n976 = property on="Мишень 2" class="Pict"("Position"=w1608) -> ()  [unwired: 2 in, 2 out]
            n977 = property on="XY лазера увожу за экран при вкл" class="Bool (strict)"("Position"=w1556) -> ()  [unwired: 2 in, 2 out]
            n978 = property on="Мишень 3" class="Pict"("Position"=w1608) -> ()  [unwired: 2 in, 2 out]
            n979 = property on="Мишень 4" class="Pict"("Position"=w1608) -> ()  [unwired: 2 in, 2 out]
            n980 = property on="Мишень 3" class="Pict"("Draw Area Size"=w1609) -> ()  [unwired: 2 in, 2 out]
            n981 = property on="Мишень 4" class="Pict"("Draw Area Size"=w1609) -> ()  [unwired: 2 in, 2 out]
            n982 = property on="Мишень 5" class="Pict"("Position"=w1608) -> ()  [unwired: 2 in, 2 out]
            n983 = property on="Мишень 6" class="Pict"("Position"=w1608) -> ()  [unwired: 2 in, 2 out]
            n984 = property on="Мишень 5" class="Pict"("Draw Area Size"=w1609) -> ()  [unwired: 2 in, 2 out]
            n985 = property on="Мишень 6" class="Pict"("Draw Area Size"=w1609) -> ()  [unwired: 2 in, 2 out]
            n986 = property on="текущ. инфо" class="Bool (strict)"("Position"=w1556) -> ()  [unwired: 2 in, 2 out]
            n987 = property on="Мишень 7" class="Pict"("Position"=w1608) -> ()  [unwired: 2 in, 2 out]
            n988 = property on="Мишень 8" class="Pict"("Position"=w1608) -> ()  [unwired: 2 in, 2 out]
            n989 = property on="Мишень 7" class="Pict"("Draw Area Size"=w1609) -> ()  [unwired: 2 in, 2 out]
            n990 = property on="Мишень 8" class="Pict"("Draw Area Size"=w1609) -> ()  [unwired: 2 in, 2 out]
            n991 = property on="Мишень 9" class="Pict"("Position"=w1608) -> ()  [unwired: 2 in, 2 out]
            n992 = property on="Мишень 10" class="Pict"("Position"=w1608) -> ()  [unwired: 2 in, 2 out]
            n993 = property on="Мишень 9" class="Pict"("Draw Area Size"=w1609) -> ()  [unwired: 2 in, 2 out]
            n994 = property on="Мишень 10" class="Pict"("Draw Area Size"=w1609) -> ()  [unwired: 2 in, 2 out]
          }
        }
      }
      event "Загрузить настройки": Value Change {
        # "Восстановление конфигурации из файла"
        n995 = event-data() -> ("OldVal"=w1619:bool)  [unwired: 1 out]
        n996 = property on="Загрузить \nнастройки" class="Bool (strict)"(error in=w1618, "Value"=w1619) -> (error out=w1615:errorcluster)  [unwired: 1 in, 1 out]
        n997 = Read from Text File(prompt (Open existing file)="Укажите  файл конфигурации...", error in=w1615) -> (refnum out=w1612:refnum<file>, text=w1616:string, cancelled=w1611:bool, error out=w1614:errorcluster)  [unwired: 2 in]
        n998 = case shown="False" w1611 {
          tunnel: w1616 -> [w1707 _]
          tunnel: w1614 -> [w1630 w1717]
          tunnel: [w1629 w1717] -> w1613
          tunnel: w1612 -> [w1626 _]
          frame False {
            n999 = control-ref of="Мишень 1"() -> (w1705:refnum<vi>)
            n1000 = control-ref of="Мишень 2"() -> (w1704:refnum<vi>)
            n1001 = control-ref of="Мишень 3"() -> (w1703:refnum<vi>)
            n1002 = control-ref of="Мишень 4"() -> (w1702:refnum<vi>)
            n1003 = control-ref of="Мишень 5"() -> (w1701:refnum<vi>)
            n1004 = control-ref of="Мишень 6"() -> (w1700:refnum<vi>)
            n1005 = control-ref of="Мишень 7"() -> (w1699:refnum<vi>)
            n1006 = control-ref of="Мишень 8"() -> (w1698:refnum<vi>)
            n1007 = control-ref of="Мишень 9"() -> (w1697:refnum<vi>)
            n1008 = control-ref of="Мишень 10"() -> (w1696:refnum<vi>)
            n1009 = Refnum to Path(1:w1626) -> (0:w1625:path)
            n1010 = Bundle("Мишень 1"=w1705, "Мишень 2"=w1704, "Мишень 3"=w1703, "Мишень 4"=w1702, "Мишень 5"=w1701, "Мишень 6"=w1700, "Мишень 7"=w1699, "Мишень 8"=w1698, "Мишень 9"=w1697, "Мишень 10"=w1696) -> (w1695:T17)  [unwired: 1 in]
            n1011 = call "Строку в параметры мишени (SubVI).vi"("Параметры мишени строка"=w1707) -> ("Кластер параметров мишени"=w1642:T1, "Остаток строки параметров"=w1708:string)  [unwired: 13 in]
            n1012 = call "Строку в параметры мишени (SubVI).vi"("Параметры мишени строка"=w1708) -> ("Кластер параметров мишени"=w1641:T1, "Остаток строки параметров"=w1716:string)  [unwired: 13 in]
            n1013 = call "Строку в параметры мишени (SubVI).vi"("Параметры мишени строка"=w1716) -> ("Кластер параметров мишени"=w1640:T1, "Остаток строки параметров"=w1714:string)  [unwired: 13 in]
            n1014 = call "Строку в параметры мишени (SubVI).vi"("Параметры мишени строка"=w1714) -> ("Кластер параметров мишени"=w1639:T1, "Остаток строки параметров"=w1715:string)  [unwired: 13 in]
            n1015 = call "Строку в параметры мишени (SubVI).vi"("Параметры мишени строка"=w1715) -> ("Кластер параметров мишени"=w1638:T1, "Остаток строки параметров"=w1710:string)  [unwired: 13 in]
            n1016 = call "Строку в параметры мишени (SubVI).vi"("Параметры мишени строка"=w1710) -> ("Кластер параметров мишени"=w1637:T1, "Остаток строки параметров"=w1711:string)  [unwired: 13 in]
            n1017 = call "Строку в параметры мишени (SubVI).vi"("Параметры мишени строка"=w1711) -> ("Кластер параметров мишени"=w1636:T1, "Остаток строки параметров"=w1713:string)  [unwired: 13 in]
            n1018 = call "Строку в параметры мишени (SubVI).vi"("Параметры мишени строка"=w1713) -> ("Кластер параметров мишени"=w1635:T1, "Остаток строки параметров"=w1712:string)  [unwired: 13 in]
            n1019 = call "Строку в параметры мишени (SubVI).vi"("Параметры мишени строка"=w1712) -> ("Кластер параметров мишени"=w1634:T1, "Остаток строки параметров"=w1709:string)  [unwired: 13 in]
            n1020 = call "Строку в параметры мишени (SubVI).vi"("Параметры мишени строка"=w1709) -> ("Кластер параметров мишени"=w1633:T1, "Остаток строки параметров"=w1706:string)  [unwired: 13 in]
            n1021 = call "Упр. видимостью мишеней (SubVI).vi"("Строка параметров видимости мишеней"=w1706, "Кластер reference"=w1695) -> ("Кластер reference out"=w1627:T18, "Остаток строки"=w1694:string, "Кол-во видимых мишеней"=w1628:u8)  [unwired: 11 in]
            n1022 = call "Строку в числовые данные мишеней (SubVI).vi"("Строка с числовыми параметрами мишени"=w1694) -> ("Остаток строки"=w1681:string, "Кластер числовых параметров мишеней"=w1693:T19)  [unwired: 25 in]
            n1023 = call "Строку в числовые данные мишеней (SubVI).vi"("Строка с числовыми параметрами мишени"=w1681) -> ("Остаток строки"=w1670:string, "Кластер числовых параметров мишеней"=w1682:T19)  [unwired: 25 in]
            n1024 = call "Строку в числовые данные мишеней (SubVI).vi"("Строка с числовыми параметрами мишени"=w1670) -> ("Остаток строки"=w1658:string, "Кластер числовых параметров мишеней"=w1659:T19)  [unwired: 25 in]
            n1025 = call "Строка параметров в I8 (SubVI).vi"("Строка чисел параметров мишеней"=w1658) -> ("Остаток строки"=w1645:string, "Кластер чисел типа I8"=w1657:T20)  [unwired: 17 in]
            n1026 = Match Pattern(string=w1645, regular expression="-----") -> (after substring=w1643:string)  [unwired: 1 in, 3 out]
            n1027 = local write "Текущая конфигурация:"(w1625) -> ()
            n1028 = local write "Счетчик мишеней"(w1628) -> ()
            n1029 = Decimal String To Number(string=w1643, default (0L)=u16 0 ("default (0 I32)")) -> (number=w1620:u16)  [unwired: 1 in, 1 out]
            n1030 = property on="id мишени" class="DigNum (strict)"("Val(Sgnl)"=w1620) -> ()  [unwired: 2 in, 2 out]
            n1031 = Unbundle(w1693) -> ("1"=w1692:u16, "2"=w1691:u16, "3"=w1690:u16, "4"=w1689:u16, "5"=w1688:u16, "6"=w1687:u16, "7"=w1686:u16, "8"=w1685:u16, "9"=w1684:u16, "10"=w1683:u16)
            n1032 = local write "М1"(w1642) -> ()
            n1033 = local write "М2"(w1641) -> ()
            n1034 = local write "М3"(w1640) -> ()
            n1035 = local write "М4"(w1639) -> ()
            n1036 = local write "М5"(w1638) -> ()
            n1037 = local write "М6"(w1637) -> ()
            n1038 = local write "М7"(w1636) -> ()
            n1039 = local write "М8"(w1635) -> ()
            n1040 = local write "М9"(w1634) -> ()
            n1041 = local write "М10"(w1633) -> ()
            n1042 = call "Строку в коор. выстрела лазера (SubVI).vi"("Строка числовых параметров мишеней"=w1643) -> ("Положение XY лазера"=w1624:cluster{i32, i32}, "Положение информации о выстреле"=w1623:cluster{i32, i32})  [unwired: 25 in]
            n1043 = local write "Выстрелов осталось M1"(w1692) -> ()
            n1044 = local write "Выстрелов осталось M2"(w1691) -> ()
            n1045 = local write "Выстрелов осталось M3"(w1690) -> ()
            n1046 = local write "Выстрелов осталось M4"(w1689) -> ()
            n1047 = local write "Выстрелов осталось M5"(w1688) -> ()
            n1048 = local write "Выстрелов осталось M6"(w1687) -> ()
            n1049 = local write "Выстрелов осталось M7"(w1686) -> ()
            n1050 = local write "Выстрелов осталось M8"(w1685) -> ()
            n1051 = local write "Выстрелов осталось M9"(w1684) -> ()
            n1052 = local write "Выстрелов осталось M10"(w1683) -> ()
            n1053 = property on="XY лазера" class="Bool (strict)"("Position"=w1624) -> (error out=w1621:errorcluster)  [unwired: 2 in, 1 out]
            n1054 = Bundle("Кластер параметров мишени"=w1642, "Кластер параметров мишени"=w1641, "Кластер параметров мишени"=w1640, "Кластер параметров мишени"=w1639, "Кластер параметров мишени"=w1638, "Кластер параметров мишени"=w1637, "Кластер параметров мишени"=w1636, "Кластер параметров мишени"=w1635, "Кластер параметров мишени"=w1634, "Кластер параметров мишени"=w1633) -> (w1632:T21)  [unwired: 1 in]
            n1055 = property on="текущ. инфо" class="Bool (strict)"(error in=w1621, "Position"=w1623) -> (error out=w1622:errorcluster)  [unwired: 1 in, 1 out]
            n1056 = call "Восстановление мишеней (SubVI).vi"("error in"=w1630, "Параметры всех мишеней"=w1632, "Кластер reference"=w1627) -> ("error out"=w1631:errorcluster)  [unwired: 12 in]
            n1057 = Unbundle(w1682) -> ("1"=w1680:u16, "2"=w1679:u16, "3"=w1678:u16, "4"=w1677:u16, "5"=w1676:u16, "6"=w1675:u16, "7"=w1674:u16, "8"=w1673:u16, "9"=w1672:u16, "10"=w1671:u16)
            n1058 = local write "выстрел X М1"(w1680) -> ()
            n1059 = local write "выстрел Y М1"(w1679) -> ()
            n1060 = local write "выстрел X М2"(w1678) -> ()
            n1061 = local write "выстрел Y М2"(w1677) -> ()
            n1062 = local write "выстрел X М3"(w1676) -> ()
            n1063 = local write "выстрел Y М3"(w1675) -> ()
            n1064 = local write "выстрел X М4"(w1674) -> ()
            n1065 = local write "выстрел Y М4"(w1673) -> ()
            n1066 = local write "выстрел X М5"(w1672) -> ()
            n1067 = local write "выстрел Y М5"(w1671) -> ()
            n1068 = Unbundle(w1659) -> ("1"=w1660:u16, "2"=w1661:u16, "3"=w1662:u16, "4"=w1663:u16, "5"=w1664:u16, "6"=w1665:u16, "7"=w1666:u16, "8"=w1667:u16, "9"=w1668:u16, "10"=w1669:u16)
            n1069 = local write "выстрел X М6"(w1660) -> ()
            n1070 = local write "выстрел Y М6"(w1661) -> ()
            n1071 = local write "выстрел X М7"(w1662) -> ()
            n1072 = local write "выстрел Y М7"(w1663) -> ()
            n1073 = local write "выстрел X М8"(w1664) -> ()
            n1074 = local write "выстрел Y М8"(w1665) -> ()
            n1075 = local write "выстрел X М9"(w1666) -> ()
            n1076 = local write "выстрел Y М9"(w1667) -> ()
            n1077 = local write "выстрел X М10"(w1668) -> ()
            n1078 = local write "выстрел Y М10"(w1669) -> ()
            n1079 = Unbundle(w1657) -> ("default value 1"=w1656:i8, "default value 1"=w1655:i8, "default value 1"=w1654:i8, "default value 1"=w1653:i8, "default value 1"=w1652:i8, "default value 1"=w1651:i8, "default value 1"=w1650:i8, "default value 1"=w1649:i8, "default value 1"=w1648:i8, "default value 1"=w1647:i8)
            n1080 = local write "Знак перех. dX М1"(w1656) -> ()
            n1081 = local write "Знак перех. dX М2"(w1655) -> ()
            n1082 = local write "Знак перех. dX М3"(w1654) -> ()
            n1083 = local write "Знак перех. dX М4"(w1653) -> ()
            n1084 = local write "Знак перех. dX М5"(w1652) -> ()
            n1085 = local write "Знак перех. dX М6"(w1651) -> ()
            n1086 = local write "Знак перех. dX М7"(w1650) -> ()
            n1087 = local write "Знак перех. dX М8"(w1649) -> ()
            n1088 = local write "Знак перех. dX М10"(w1647) -> ()
            n1089 = local write "Знак перех. dX М9"(w1648) -> ()
            n1090 = Merge Errors(w1631, w1622) -> (w1629:errorcluster)
          }
          frame True {
          }
        }
      }
      event Panel Close? {
        # "Защита и сохранение при закрытии программы"
        n1091 = event-data() -> ()  [unwired: 2 out]
        n1092 = call <vilib>:"Three Button Dialog.vi"("Allow user to close window? (TRUE)"=TRUE, "Right Button Text (\"Cancel\")"="Отмена" ("message"), "Center Button Text (\"No\")"="Закрыть программу \nбез сохранений" ("message"), "Left Button Text (\"Yes\")"="Сохранить текущую конфигурацию \nи закрыть программу" ("message"), "message"="Вы уверены, что хотите закрыть программу?") -> ("Which Button?"=w1724:T22)  [unwired: 6 in]
        n1093 = case shown="\"Left Button\"" w1724 {
          tunnel: [w1726 FALSE ("Discard?") TRUE ("Value (Signaling)") TRUE ("Discard?")] -> w1721
          frame "Left Button" {
            n1094 = flat-sequence {
              tunnel: [w1729] -> w1728
              tunnel: w1728 -> [w1733]
              tunnel: [w1733] -> w1727
              tunnel: [TRUE ("Discard?")] -> w1725
              tunnel: w1727 -> [w1736]
              tunnel: [w1735] -> w1726
              tunnel: w1725 -> [w1735]
              frame #0 {
                n1095 = local read "TCP con ID"() -> (w1730:refnum<k5>)
                n1096 = TCP Close Connection(connection ID=w1730) -> (error out=w1729:errorcluster)  [unwired: 1 in, 2 out]
              }
              frame #1 {
                n1097 = property on="Конфигурация сохранена" class="Bool (strict)"("Val(Sgnl)"=TRUE ("Value (Signaling)")) -> ()  [unwired: 2 in, 2 out]
                "флаг закрытия с сохр." <- TRUE ("флаг закрытия")
              }
              frame #2 {
                w1740 = FALSE ("Запись в файл")
                w1739 = TRUE ("Tool Bar:Visible")
                n1098 = local write "Соединение"(w1740) -> ()
                n1099 = property on="кнопки запуска, стоп и тд" class="VI"(error in=w1736, "TB.Visible"=w1739) -> (error out=w1738:errorcluster)  [unwired: 1 in, 1 out]
                n1100 = local write "con err"(w1739) -> ()
                n1101 = local write "Соединение с блоком"(w1740) -> ()
                n1102 = call <vilib>:"General Error Handler.vi"("type of dialog (OK msg:1)"=u32 0 ("milliseconds to wait"), "error in (no error)"=w1738) -> ()  [unwired: 14 out]
              }
            }
          }
          frame "Center Button" {
            w1746 = FALSE ("Запись в файл")
            w1745 = TRUE ("Tool Bar:Visible")
            n1103 = local read "TCP con ID"() -> (w1747:refnum<k5>)
            n1104 = TCP Close Connection(connection ID=w1747) -> (error out=w1741:errorcluster)  [unwired: 1 in, 2 out]
            n1105 = flat-sequence {
              tunnel: [w1749] -> w1742
              tunnel: w1741 -> [w1749]
              frame #0 {
                n1106 = Wait (ms)(milliseconds to wait=u32 200) -> ()  [unwired: 1 out]
              }
            }
            n1107 = local write "Соединение"(w1746) -> ()
            n1108 = property on="кнопки запуска, стоп и тд" class="VI"(error in=w1742, "TB.Visible"=w1745) -> (error out=w1744:errorcluster)  [unwired: 1 in, 1 out]
            n1109 = local write "con err"(w1745) -> ()
            n1110 = local write "Соединение с блоком"(w1746) -> ()
            n1111 = call <vilib>:"General Error Handler.vi"("type of dialog (OK msg:1)"=u32 0 ("milliseconds to wait"), "error in (no error)"=w1744) -> ()  [unwired: 14 out]
          }
          frame "Right Button" {
            n1112 = local write "флаг закрытия с сохр."(FALSE ("флаг закрытия с сохр.")) -> ()
          }
          frame "Window Close" {
          }
        }
        n1113 = event-data("Discard?"=w1721) -> ()  [unwired: 1 in, 1 out]
      }
    }
    n1114 = call <vilib>:"General Error Handler.vi"("type of dialog (OK msg:1)"=u8 0, "error in (no error)"=w163) -> ("error out"=w162:errorcluster)  [unwired: 13 out]
  }
  n1115 = property class="VI"(error in=w39, "Front Panel.Resizeable"=TRUE ("Front Panel Window:Resizable")) -> (error out=w38:errorcluster)  [unwired: 1 in, 1 out]
  n1116 = property on="Мишень 7" class="Pict"(error in=w17, "Visible"=FALSE) -> (error out=w20:errorcluster)  [unwired: 1 in, 1 out]
  n1117 = property on="Мишень 8" class="Pict"(error in=w20, "Visible"=FALSE) -> (error out=w22:errorcluster)  [unwired: 1 in, 1 out]
  n1118 = property on="Мишень 9" class="Pict"(error in=w22, "Visible"=FALSE) -> (error out=w24:errorcluster)  [unwired: 1 in, 1 out]
  n1119 = property class="VI"(error in=w38, "Front Panel.ShowMenuBar"=FALSE ("Front Panel Window:Show Menu Bar")) -> ()  [unwired: 1 in, 2 out]
  n1120 = property on="Мишень 10" class="Pict"(error in=w24, "Visible"=FALSE) -> ()  [unwired: 1 in, 2 out]
  n1121 = event shown="[0] \"stop\": Value Change" {
    selector: _ -> [_]
    dyn-events: _ -> [_]
    timeout: _ -> [_]
    event "stop": Value Change {
      n1122 = event-data() -> ()  [unwired: 2 out]
      n1123 = flat-sequence {
        tunnel: [w1756] -> w1755
        tunnel: w1755 -> [w1759]
        tunnel: [w1759] -> w1754
        tunnel: w1754 -> [w1760]
        frame #0 {
          n1124 = local read "TCP con ID"() -> (w1757:refnum<k5>)
          n1125 = TCP Close Connection(connection ID=w1757) -> (error out=w1756:errorcluster)  [unwired: 1 in, 2 out]
        }
        frame #1 {
          n1126 = Wait (ms)(milliseconds to wait=u32 200) -> ()  [unwired: 1 out]
        }
        frame #2 {
          w1764 = FALSE ("Запись в файл")
          w1763 = TRUE ("Tool Bar:Visible")
          n1127 = local write "Соединение"(w1764) -> ()
          n1128 = property on="кнопки запуска, стоп и тд" class="VI"(error in=w1760, "TB.Visible"=w1763) -> (error out=w1762:errorcluster)  [unwired: 1 in, 1 out]
          n1129 = local write "con err"(w1763) -> ()
          n1130 = local write "Соединение с блоком"(w1764) -> ()
          n1131 = call <vilib>:"General Error Handler.vi"("type of dialog (OK msg:1)"=u32 0 ("milliseconds to wait"), "error in (no error)"=w1762) -> ()  [unwired: 14 out]
        }
        frame #3 {
          n1132 = Stop(stop? (T)=TRUE) -> ()
        }
      }
    }
  }
  n1133 = disable-structure shown="Disabled" {
    frame Disabled {
      n1134 = call "Команда обмена 74 (ручное упр. DragNdrop) (SubVI).vi"() -> ()  [unwired: 27 in, 1 out]
    }
    frame Enabled {
    }
  }
  n1135 = disable-structure shown="Enabled" {
    frame Enabled {
      n1136 = property on="Счетчик выстрелов:" class="DigNum (strict)"("Value"=u32 0 ("Счетчик выстрелов:")) -> ()  [unwired: 2 in, 2 out]
    }
    frame Disabled {
    }
  }
  n1137 = property on="DownButton" class="Bool (strict)"("DisabledEnum"=T2."Enabled" ("Disabled")) -> ()  [unwired: 2 in, 2 out]
  n1138 = property on="Счетчик выстрелов:" class="DigNum (strict)"("Value"=0.0 ("Счетчик выстрелов:")) -> (error out=w56:errorcluster)  [unwired: 2 in, 1 out]
  n1139 = property on="XY лазера" class="Bool (strict)"("Visible"=TRUE) -> ()  [unwired: 2 in, 2 out]
  n1140 = property on="XY лазера увожу за экран при вкл" class="Bool (strict)"("Position"=w49) -> ()  [unwired: 2 in, 2 out]
  n1141 = property on="текущ. инфо" class="Bool (strict)"("Caption.TextColor"=u32 16711680 ("цвет")) -> ()  [unwired: 2 in, 2 out]
  n1142 = property on="Выстрел по мишени!" class="DigNum (strict)"(error in=w56, "Value"=u32 0 ("Выстрел по мишени!")) -> ()  [unwired: 1 in, 2 out]
  n1143 = property on="текущ. инфо" class="Bool (strict)"("Position"=w49) -> ()  [unwired: 2 in, 2 out]
  n1144 = while {
    stop <- FALSE stop-if-true
    # "Сохранение параметров каждые 10 сек"
    n1145 = property on="Мишень 1" class="Pict"() -> ("Visible"=w1779:bool)  [unwired: 2 in, 2 out]
    n1146 = property on="Мишень 8" class="Pict"() -> ("Visible"=w1778:bool)  [unwired: 2 in, 2 out]
    n1147 = property on="Мишень 10" class="Pict"() -> ("Visible"=w1777:bool)  [unwired: 2 in, 2 out]
    n1148 = property on="Мишень 9" class="Pict"() -> ("Visible"=w1776:bool)  [unwired: 2 in, 2 out]
    n1149 = property on="Мишень 2" class="Pict"() -> ("Visible"=w1775:bool)  [unwired: 2 in, 2 out]
    n1150 = property on="Мишень 3" class="Pict"() -> ("Visible"=w1774:bool)  [unwired: 2 in, 2 out]
    n1151 = property on="Мишень 4" class="Pict"() -> ("Visible"=w1773:bool)  [unwired: 2 in, 2 out]
    n1152 = property on="Мишень 5" class="Pict"() -> ("Visible"=w1772:bool)  [unwired: 2 in, 2 out]
    n1153 = property on="Мишень 6" class="Pict"() -> ("Visible"=w1771:bool)  [unwired: 2 in, 2 out]
    n1154 = property on="Мишень 7" class="Pict"() -> ("Visible"=w1768:bool)  [unwired: 2 in, 2 out]
    n1155 = Compound Arithmetic op=OR(w1779, w1768, w1778, w1777, w1776, w1775, w1774, w1773, w1772, w1771) -> (w1769:bool)
    n1156 = case shown="True" w1769 {
      frame False {
      }
      frame True {
        n1157 = property on="Конфигурация сохранена" class="Bool (strict)"("Val(Sgnl)"=TRUE ("Value (Signaling)")) -> ()  [unwired: 2 in, 2 out]
        "Флаг резерв. сохр." <- TRUE ("Флаг резерв. сохр.")
      }
    }
    n1158 = Wait Until Next ms Multiple(millisecond multiple=u32 10000) -> ()  [unwired: 1 out]
  }
  n1159 = property on="Соединение с блоком" class="Bool (strict)"("Value"=FALSE ("Connected")) -> (error out=w37:errorcluster)  [unwired: 2 in, 1 out]
  n1160 = call-poly <vilib>:"Close Input Device.vi"("error in (no error)"=w50, "device ID"=w48) -> ()  [unwired: 9 out]
  n1161 = disable-structure shown="Enabled" {
    disable-tunnel: [w1783] -> w26
    disable-tunnel: w37 -> [w1783]
    frame Enabled {
      n1162 = local write "флаг закрытия с сохр."(FALSE ("флаг закрытия с сохр.")) -> ()
      n1163 = local write "x+1"(0.0 ("x+1")) -> ()
      n1164 = local write "stop"(FALSE ("Boolean")) -> ()
    }
  }
  n1165 = property on="Счетчик мишеней" class="DigNum (strict)"(error in=w26, "Value"=u16 0 ("Счетчик мишеней")) -> ()  [unwired: 1 in, 2 out]
  n1166 = Bundle("Счетчик мишеней"=u32 200, "Счетчик мишеней"=u32 200) -> (w9:T15)  [unwired: 1 in]
  n1167 = Bundle("Счетчик мишеней"=400, "Счетчик мишеней"=200) -> (w10:T16)  [unwired: 1 in]
  n1168 = property on="Мишень 1" class="Pict"("Draw Area Size"=w9) -> ()  [unwired: 2 in, 2 out]
  n1169 = property on="Мишень 2" class="Pict"("Draw Area Size"=w9) -> ()  [unwired: 2 in, 2 out]
  n1170 = property on="Мишень 1" class="Pict"("Position"=w10) -> ()  [unwired: 2 in, 2 out]
  n1171 = property on="Мишень 2" class="Pict"("Position"=w10) -> ()  [unwired: 2 in, 2 out]
  n1172 = property on="Мишень 3" class="Pict"("Position"=w10) -> ()  [unwired: 2 in, 2 out]
  n1173 = property on="Мишень 4" class="Pict"("Position"=w10) -> ()  [unwired: 2 in, 2 out]
  n1174 = property on="Мишень 3" class="Pict"("Draw Area Size"=w9) -> ()  [unwired: 2 in, 2 out]
  n1175 = property on="Мишень 4" class="Pict"("Draw Area Size"=w9) -> ()  [unwired: 2 in, 2 out]
  n1176 = property on="Мишень 10" class="Pict"("TipStrip"=w8) -> ()  [unwired: 2 in, 2 out]
  n1177 = property on="Мишень 9" class="Pict"("TipStrip"=w8) -> ()  [unwired: 2 in, 2 out]
  n1178 = property on="Мишень 8" class="Pict"("TipStrip"=w8) -> ()  [unwired: 2 in, 2 out]
  n1179 = property on="Мишень 7" class="Pict"("TipStrip"=w8) -> ()  [unwired: 2 in, 2 out]
  n1180 = property on="Мишень 6" class="Pict"("TipStrip"=w8) -> ()  [unwired: 2 in, 2 out]
  n1181 = property on="Мишень 5" class="Pict"("TipStrip"=w8) -> ()  [unwired: 2 in, 2 out]
  n1182 = property on="Мишень 4" class="Pict"("TipStrip"=w8) -> ()  [unwired: 2 in, 2 out]
  n1183 = property on="Мишень 3" class="Pict"("TipStrip"=w8) -> ()  [unwired: 2 in, 2 out]
  n1184 = property on="Мишень 2" class="Pict"("TipStrip"=w8) -> ()  [unwired: 2 in, 2 out]
  n1185 = property on="Мишень 1" class="Pict"("TipStrip"=w8) -> ()  [unwired: 2 in, 2 out]
  n1186 = property on="Мишень 5" class="Pict"("Position"=w10) -> ()  [unwired: 2 in, 2 out]
  n1187 = property on="Мишень 6" class="Pict"("Position"=w10) -> ()  [unwired: 2 in, 2 out]
  n1188 = property on="Мишень 5" class="Pict"("Draw Area Size"=w9) -> ()  [unwired: 2 in, 2 out]
  n1189 = property on="Мишень 6" class="Pict"("Draw Area Size"=w9) -> ()  [unwired: 2 in, 2 out]
  n1190 = property on="Мишень 7" class="Pict"("Position"=w10) -> ()  [unwired: 2 in, 2 out]
  n1191 = property on="Мишень 8" class="Pict"("Position"=w10) -> ()  [unwired: 2 in, 2 out]
  n1192 = property on="Мишень 7" class="Pict"("Draw Area Size"=w9) -> ()  [unwired: 2 in, 2 out]
  n1193 = property on="Мишень 8" class="Pict"("Draw Area Size"=w9) -> ()  [unwired: 2 in, 2 out]
  n1194 = property on="Мишень 9" class="Pict"("Position"=w10) -> ()  [unwired: 2 in, 2 out]
  n1195 = property on="Мишень 10" class="Pict"("Position"=w10) -> ()  [unwired: 2 in, 2 out]
  n1196 = property on="Мишень 9" class="Pict"("Draw Area Size"=w9) -> ()  [unwired: 2 in, 2 out]
  n1197 = property on="Мишень 10" class="Pict"("Draw Area Size"=w9) -> ()  [unwired: 2 in, 2 out]
  "Осталось:" <- u16 0 ("До перемотки осталось")
